vi "Autonomous Independent.vi"() -> ()   [LabVIEW 2014]
doc: "This VI is called when autonomous begins, and will automatically be terminated when autonomous ends. You can carry out timed or sensor driven robot movement independently without needing to return to the caller."
uses:
  Robot Global Data.vi
  <vilib>/Rock Robotics/Network Tables/SD Write Number.vi
  <vilib>/Rock Robotics/Network Tables/SD Read Number.vi
  <vilib>/Rock Robotics/WPI/RobotDrive/WPI_RobotDriveMecanumDrive_Cartesian.vi
  <vilib>/Rock Robotics/Network Tables/SD Write Numeric Array.vi
panel:
  out "Current Movement, for debugging":T1 {"Z Joystick Value" scale=-1.0..1.0; "Y Joystick Value" scale=1.0..-1.0; "X Joystick Value" scale=-1.0..1.0}
  in  "Array of robot movements":T2(array[cluster]) {"Z Joystick Value" scale=-1.0..1.0; "Y Joystick Value" scale=1.0..-1.0; "X Joystick Value" scale=-1.0..1.0}
  # "Be sure to right-click and choose Data Operations>>Make Current Value default if you want to save the array values with the VI"
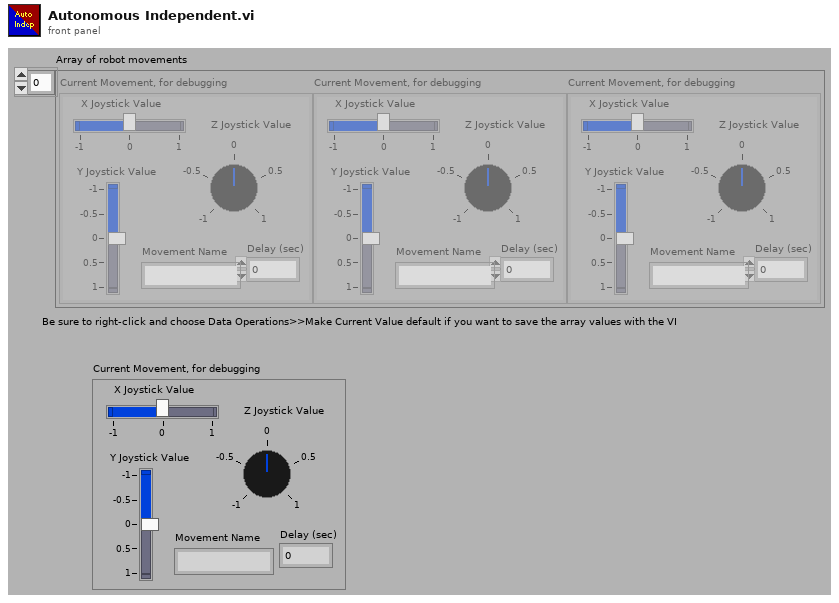
[diagram p1: front panel]
types:
  T1 = cluster{"X Joystick Value":dbl, "Y Joystick Value":dbl, "Z Joystick Value":dbl, "Delay (sec)":dbl, "Movement Name":string}
  T2 = cluster{"X Joystick Value":dbl, "Y Joystick Value":dbl, "Z Joystick Value":dbl, "Delay (sec)":dbl, "Movement Name":string}[]
  T3 = typedef "WPI_RobotDriveDevRef.ctl" = cluster{"DevStatus":errorcluster, "Motors[]":T4[], "Square Inputs":bool, "Max Output":dbl}
  T4 = typedef "WPI_MotorControlDeviceRef.ctl" = cluster{"DeviceStatus":errorcluster, "Type":T5, "PWM":cluster{"Controller":T6, "PWM Channel":T7, "DeadBand":T8}, "CAN":cluster{"Device Number":u8, "Control Mode":T9, "Semaphore":T10, "Max Vout":dbl, "TalonSRX Control Mode":T11}, "Invert":bool, "TransformRef":T12, "InvTransformRef":T12}
  T5 = typedef "WPI_MotorControlType.ctl" = enum16{"PWM", "CAN", "CANTalonSRX"}
  T6 = typedef "FPGA_TypedefDigitalModule.ctl" = enum16{"Controller 1"}
  T7 = typedef "FPGA_DIOPWMChannel.ctl" = enum8{"PWM 0", "PWM 1", "PWM 2", "PWM 3", "PWM 4", "PWM 5", "PWM 6", "PWM 7", "PWM 8", "PWM 9", "PWM MXP 0", "PWM MXP 1", "PWM MXP 2", "PWM MXP 3", "PWM MXP 4", "PWM MXP 5", "PWM MXP 6", "PWM MXP 7", "PWM MXP 8", "PWM MXP 9", "Invalid"}
  T8 = typedef "WPI_PWMDeadband.ctl" = cluster{"Name":string, "maxPositivePwm":i32, "minPositivePwm":i32, "centerPwm":i32, "maxNegativePwm":i32, "minNegativePwm":i32, "angularRange":u16}
  T9 = typedef "WPI_CANJaguar_ControlMode.ctl" = enum8{"Percent VBus", "Current", "Speed", "Position", "Voltage"}
  T10 = typedef "Semaphore RefNum" = refnum<k1>
  T11 = typedef "WPI_CANTalonSRX_APIControlMode.ctl" = enum8{"Percent VBus", "Speed", "Position", "Slave", "Unchanged / Invalid"}
  T12 = typedef "WPI_PWMTransform_ConPane.ctl" = refnum<vi>
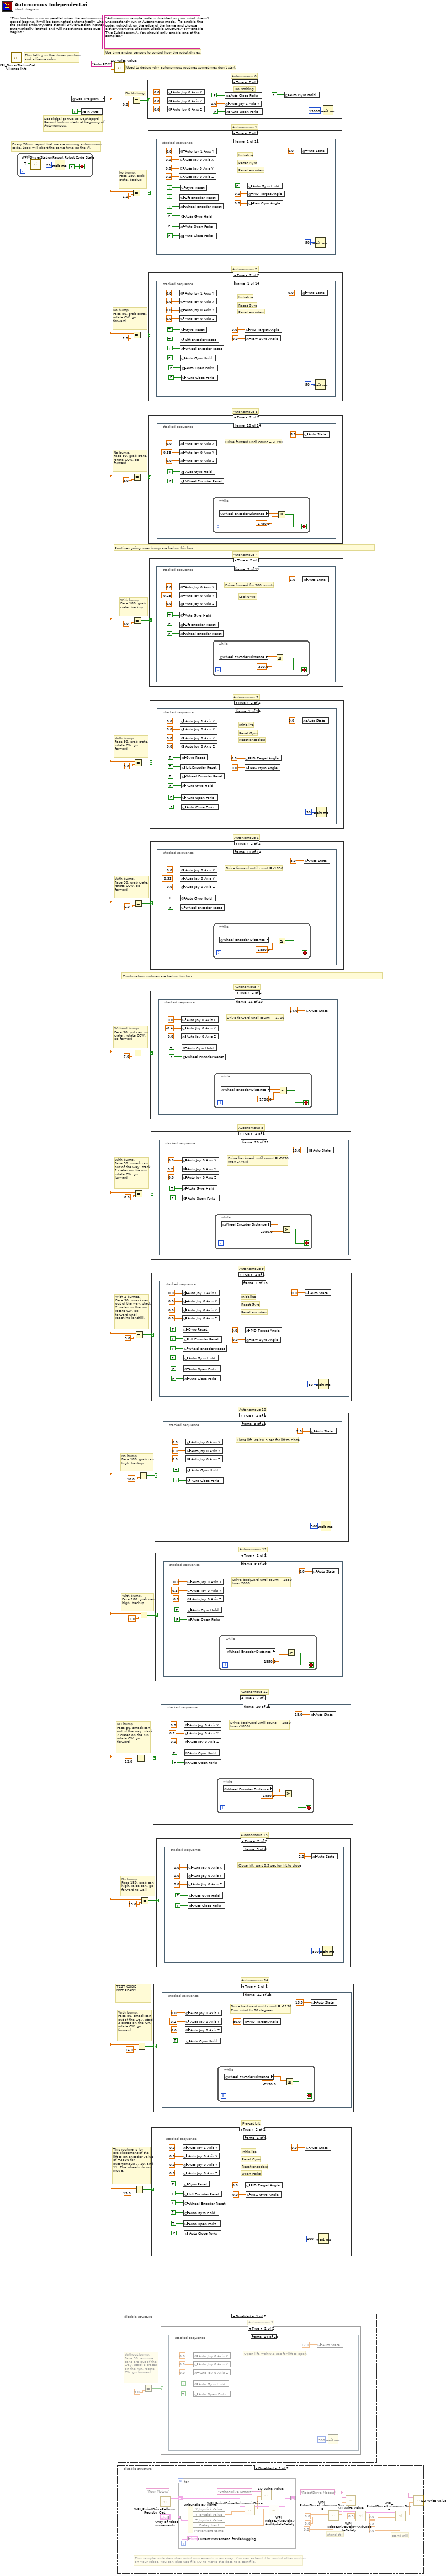
[diagram p0: block diagram]
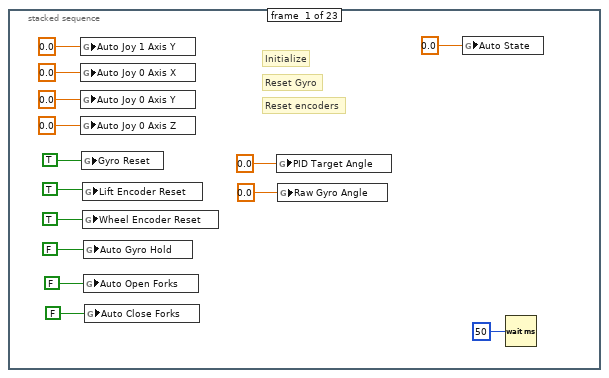
[diagram p3: hidden frame]
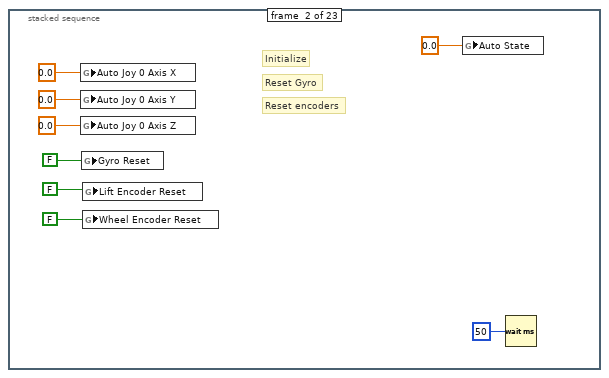
[diagram p4: hidden frame]
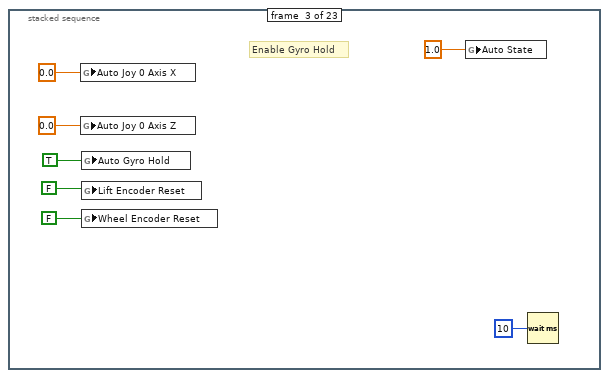
[diagram p5: hidden frame]
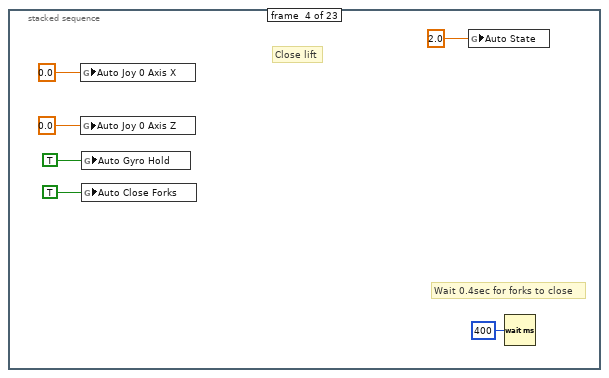
[diagram p6: hidden frame]
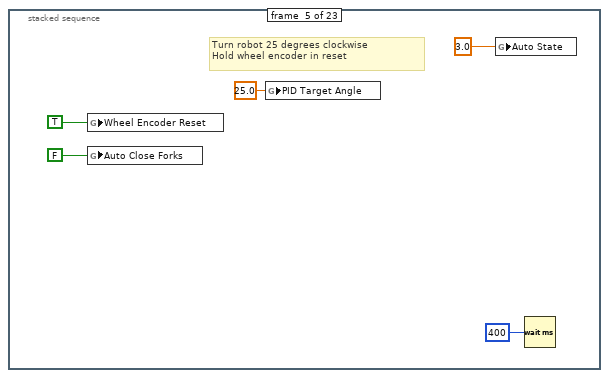
[diagram p7: hidden frame]
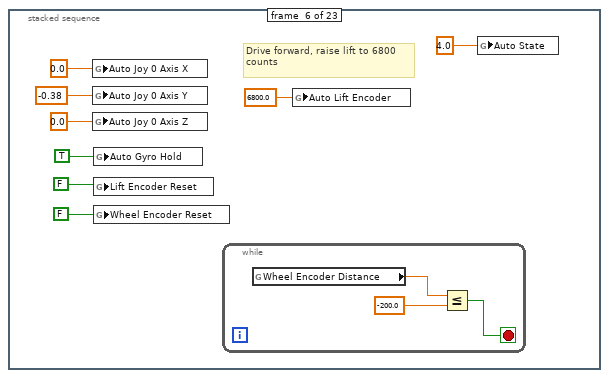
[diagram p8: hidden frame]
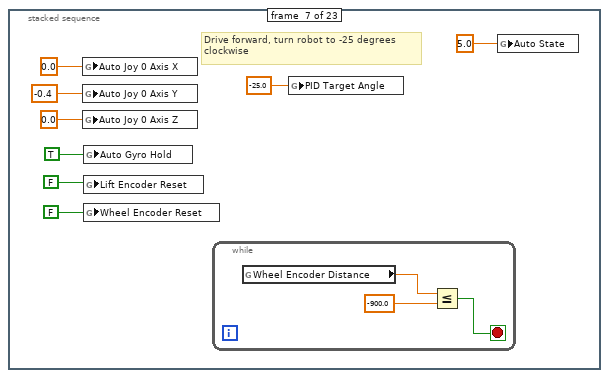
[diagram p9: hidden frame]
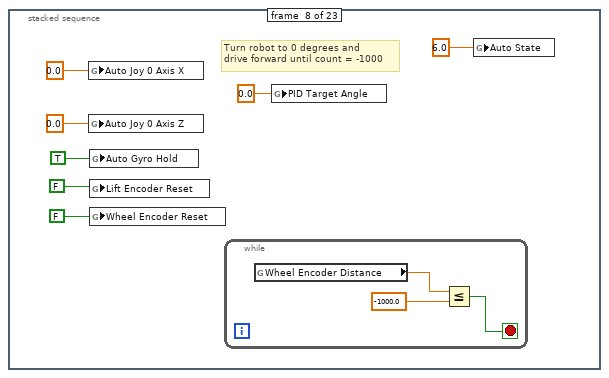
[diagram p10: hidden frame]
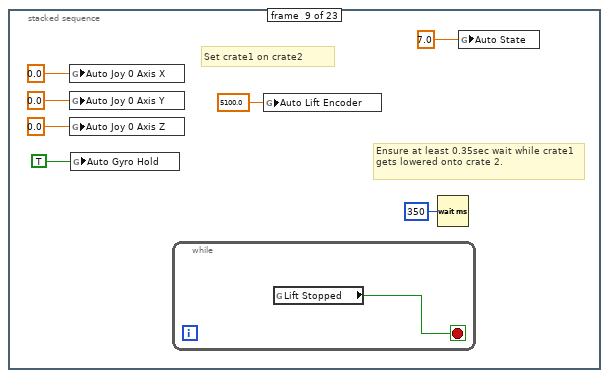
[diagram p11: hidden frame]
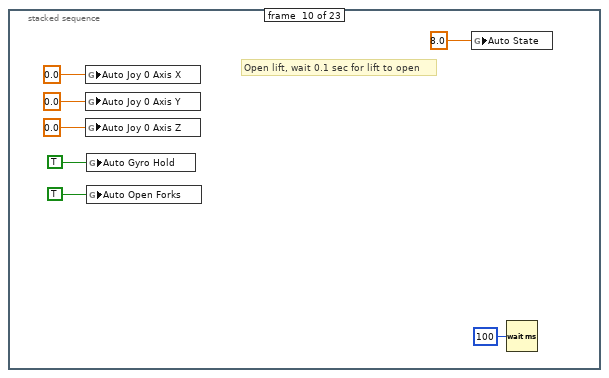
[diagram p12: hidden frame]
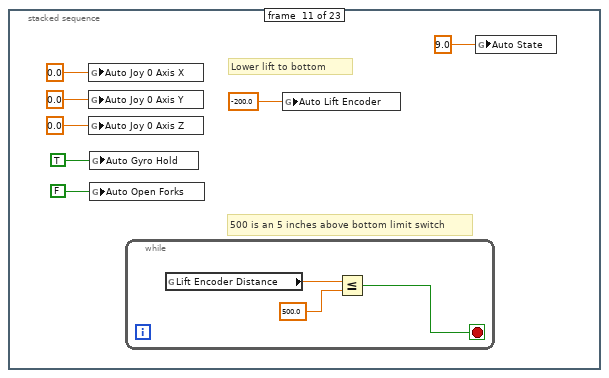
[diagram p13: hidden frame]
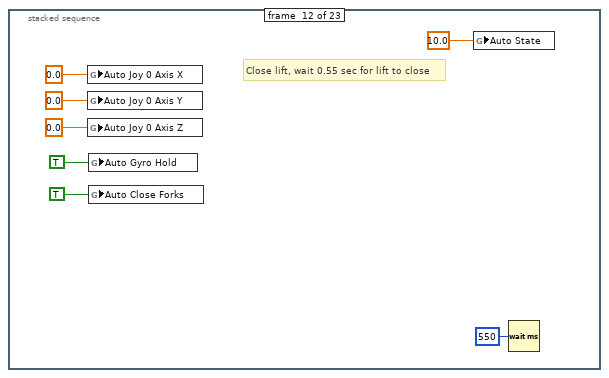
[diagram p14: hidden frame]
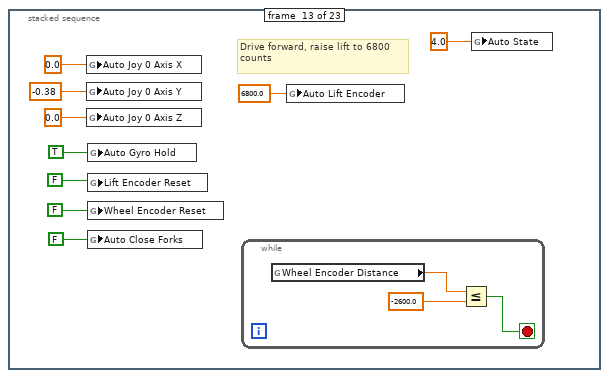
[diagram p15: hidden frame]
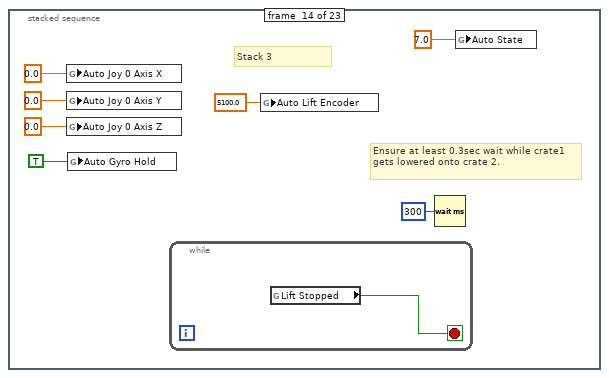
[diagram p16: hidden frame]
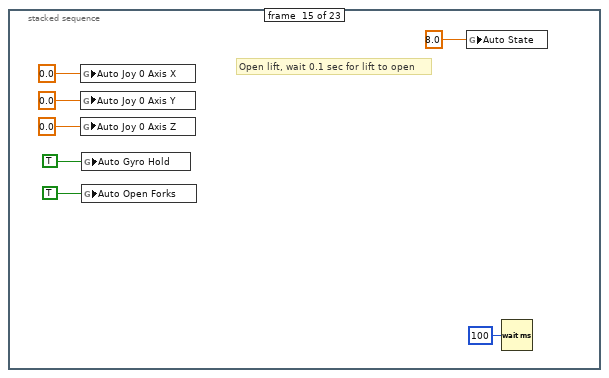
[diagram p17: hidden frame]
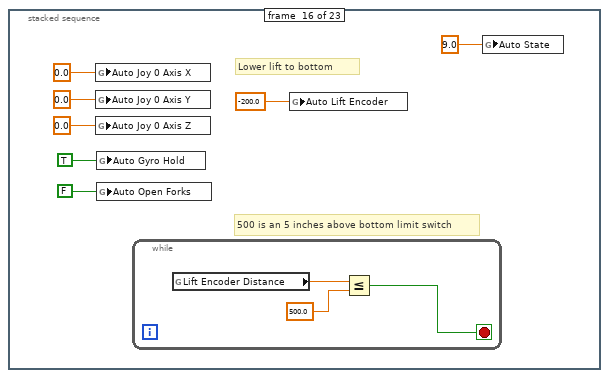
[diagram p18: hidden frame]
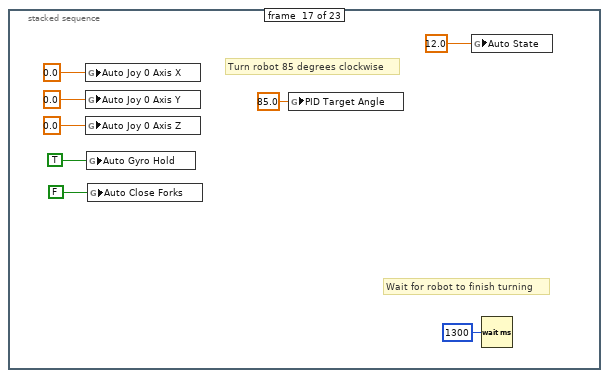
[diagram p19: hidden frame]
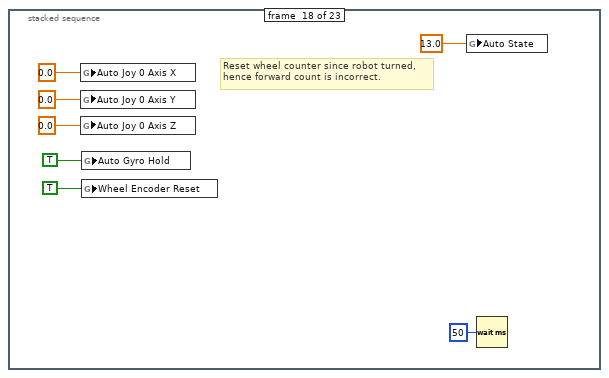
[diagram p20: hidden frame]
diagram:
  (unwired) "Autonomous sample code is disabled so your robot doesn't unexpectantly run in Autonomous mode.  To enable this code, right-click on the edge of the frame and choose either \"Remove Diagram Disable Structure\" or \"Enable This Subdiagram\". You should only enable one of the samples."
  (unwired) "This function is run in parallel when the autonomous period begins. It will be terminated automatically when the period ends.\n\nNote that all Driver Station inputs are automatically latched and will not change once auto begins."
  # "TEST CODE\nNOT READY"
  # "With bump.\nFace 90, smack can out of the way, stack 3 crates on the run, rotate CW, go forward"
  # "Autonomous 14"
  # "No bump.\nFace 180, grab can high, raise can, go forward to wall"
  # "Autonomous 13"
  # "Used to debug why autonomous routines sometimes don't start."
  # "NO bump.\nFace 90, smack can out of the way, stack 2 crates on the run, rotate CW, go forward"
  # "Autonomous 12"
  # "With bump.\nFace 180, grab can high, backup"
  # "Autonomous 11"
  # "No bump.\nFace 180, grab can high, backup"
  # "Autonomous 10"
  # "Set global to true so Dashboard Record funtion starts at begining of Autonomous."
  # "This routine is for pre-placement of the lift to an encoder value of +3500 for autonomous 7, 10, and 11. The wheels do not move."
  # "Pre-set Lift"
  # "With 2 bumps.\nFace 90, smack can out of the way, stack 2 crates on the run, rotate CW, go forward until reaching landfill."
  # "Autonomous 9"
  # "With bump.\nFace 90, smack can out of the way, stack 2 crates on the run, rotate CW, go forward"
  # "Autonomous 8"
  # "Without bump.\nFace 90, put can on crate , rotate CCW, go forward"
  # "Autonomous 7"
  # "Combination routines are below this box."
  # "With bump.\nFace 90, grab crate, rotate CCW, go forward"
  # "Autonomous 6"
  # "With bump.\nFace 90, grab crate, rotate CW, go forward"
  # "Autonomous 5"
  # "Routines going over bump are below this box."
  # "With bump.\nFace 180, grab crate, backup"
  # "Autonomous 4"
  # "No bump.\nFace 90, grab crate, rotate CCW, go forward"
  # "Autonomous 3"
  # "No bump.\nFace 90, grab crate, rotate CW, go forward"
  # "No bump.\nFace 180, grab crate, backup"
  # "Do Nothing"
  # "Autonomous 2"
  # "Autonomous 1"
  # "Autonomous 0"
  # "Every 20ms, report that we are running autonomous\ncode. Loop will abort the same time as the VI."
  # "Use time and/or sensors to control how the robot drives."
  # "This tells you the driver position\nand alliance color"
  n1 = call <vilib>:"WPI_DriverStationGet Alliance Info.vi"() -> ()  [unwired: 12 out]
  n2 = while {
    stop <- FALSE stop-if-true
    n3 = call <vilib>:"WPI_DriverStationReport Robot Code State.vi"("Autonomous"=TRUE) -> ()  [unwired: 10 in, 1 out]
    n4 = Wait (ms)(milliseconds to wait=u32 20) -> ()  [unwired: 1 out]
  }
  n5 = global read "Robot Global Data.vi" "Auto  Program"() -> (w1:dbl)
  n6 = global write "Robot Global Data.vi" "In Auto"(TRUE ("In Auto")) -> ()
  n7 = call-poly <vilib>:"SD Write Value.vi"("Numeric"=w1, "Name"="Auto PGM") -> ()  [unwired: 8 in, 2 out]
  n8 = disable-structure shown="Disabled" {
    frame Disabled {
      w50 = "RobotDrive Motors" ("Name")
      # "stand still"
      # "stand still"
      # "This sample code describes robot movements in an array. You can extend it to control other motors\non your robot. You can also use file I/O to move the data to a text file."
      n9 = call <vilib>:"WPI_RobotDriveRefNum Registry Get.vi"("refnum name"="Four Motors") -> ("RobotDriveDevRef"=w52:T3)  [unwired: 1 in, 9 out]
      n10 = for {
        shift-right: [w60] -> _
        shift-left: w52 -> [w61]
        tunnel: "Array of robot movements" -> [w56] mode=indexing
        n11 = Unbundle By Name(w56) -> ("X Joystick Value"=w59:dbl, "Y Joystick Value"=w58:dbl, "Z Joystick Value"=w55:dbl, "Delay (sec)"=w57:dbl)  [unwired: 1 out]
        n12 = call-poly <vilib>:"WPI_RobotDriveHolonomicDrive.vi"("Rotation"=w55, "Y"=w58, "X"=w59, "RobotDriveDevRef"=w61) -> ("Motor Values"=w54:dbl[], "RobotDriveDevRef"=w62:T3)  [unwired: 5 in, 1 out]
        n13 = call-poly <vilib>:"SD Write Value.vi"("Numeric Array"=w54, "Name"="RobotDrive Motors") -> ()  [unwired: 8 in, 2 out]
        n14 = call <vilib>:"WPI_RobotDriveDelayAndUpdateSafety.vi"("Delay (s)"=w57, "RobotDriveDevRef"=w62) -> ("RobotDriveDevRef 2"=w60:T3)  [unwired: 8 in, 1 out]
        "Current Movement, for debugging" <- w56
      }
      n15 = call-poly <vilib>:"WPI_RobotDriveHolonomicDrive.vi"("Rotation"=0.0, "Y"=0.0 ("X axis value"), "X"=0.0 ("X axis value")) -> ("Motor Values"=w48:dbl[], "RobotDriveDevRef"=w43:T3)  [unwired: 6 in, 1 out]
      n16 = call-poly <vilib>:"SD Write Value.vi"("Numeric Array"=w48, "Name"=w50) -> ()  [unwired: 8 in, 2 out]
      n17 = call <vilib>:"WPI_RobotDriveDelayAndUpdateSafety.vi"("Delay (s)"=0.5, "RobotDriveDevRef"=w43) -> ("RobotDriveDevRef 2"=w44:T3)  [unwired: 8 in, 1 out]
      n18 = call-poly <vilib>:"WPI_RobotDriveHolonomicDrive.vi"("Rotation"=0.0 ("X axis value"), "Y"=0.0 ("X axis value"), "X"=0.0 ("X axis value"), "RobotDriveDevRef"=w44) -> ("Motor Values"=w49:dbl[])  [unwired: 5 in, 2 out]
      n19 = call-poly <vilib>:"SD Write Value.vi"("Numeric Array"=w49, "Name"=w50) -> ()  [unwired: 8 in, 2 out]
    }
    frame Enabled {
    }
  }
  n20 = disable-structure shown="Disabled" {
    frame Disabled {
      # "Without bump.\nFace 90, assume cans are out of the way, stack 3 crates on the run, rotate CW, go forward"
      # "Autonomous 9"
      n21 = Equal?(y=9.0) -> (x=w64:dbl, x = y?=w65:bool)
      n22 = case shown="True" w65 {
        frame False {
        }
        frame True {
          n23 = stacked-sequence {
            frame #0 {
              # "Reset encoders"
              # "Reset Gyro"
              # "Initialize"
              n24 = global write "Robot Global Data.vi" "Auto Joy 1 Axis Y"(0.0 ("Auto Joy 0 Axis X")) -> ()
              n25 = global write "Robot Global Data.vi" "Auto Joy 0 Axis X"(0.0 ("Auto Joy 0 Axis X")) -> ()
              n26 = global write "Robot Global Data.vi" "Auto Joy 0 Axis Y"(0.0 ("Auto Joy 0 Axis X")) -> ()
              n27 = global write "Robot Global Data.vi" "Auto Joy 0 Axis Z"(0.0 ("Auto Joy 0 Axis X")) -> ()
              n28 = global write "Robot Global Data.vi" "Gyro Reset"(TRUE ("Auto Gyro Hold")) -> ()
              n29 = global write "Robot Global Data.vi" "Lift Encoder Reset"(TRUE ("Auto Gyro Hold")) -> ()
              n30 = global write "Robot Global Data.vi" "Wheel Encoder Reset"(TRUE ("Wheel Encoder Reset")) -> ()
              n31 = global write "Robot Global Data.vi" "Auto Gyro Hold"(FALSE ("Auto Gyro Hold")) -> ()
              n32 = global write "Robot Global Data.vi" "Auto Open Forks"(FALSE ("Auto Gyro Hold")) -> ()
              n33 = global write "Robot Global Data.vi" "Auto Close Forks"(FALSE ("Auto Gyro Hold")) -> ()
              n34 = global write "Robot Global Data.vi" "PID Target Angle"(0.0 ("Auto Joy 0 Axis Z")) -> ()
              n35 = global write "Robot Global Data.vi" "Raw Gyro Angle"(0.0 ("Auto Joy 0 Axis Z")) -> ()
              n36 = global write "Robot Global Data.vi" "Auto State"(0.0 ("Auto State")) -> ()
              n37 = Wait (ms)(milliseconds to wait=u32 50) -> ()  [unwired: 1 out]
            }
            frame #1 {
              # "Adjust this wait so it is long enought to allow alliance robots to get cans out of our way.\nSet to 2.0 seconds."
              # "Reset encoders"
              # "Reset Gyro"
              # "Initialize"
              n38 = global write "Robot Global Data.vi" "Auto Joy 0 Axis X"(0.0 ("Auto Joy 0 Axis X")) -> ()
              n39 = global write "Robot Global Data.vi" "Auto Joy 0 Axis Y"(0.0 ("Auto Joy 0 Axis X")) -> ()
              n40 = global write "Robot Global Data.vi" "Auto Joy 0 Axis Z"(0.0 ("Auto Joy 0 Axis X")) -> ()
              n41 = global write "Robot Global Data.vi" "Gyro Reset"(FALSE ("Auto Gyro Hold")) -> ()
              n42 = global write "Robot Global Data.vi" "Lift Encoder Reset"(FALSE ("Auto Gyro Hold")) -> ()
              n43 = global write "Robot Global Data.vi" "Wheel Encoder Reset"(FALSE ("Wheel Encoder Reset")) -> ()
              n44 = global write "Robot Global Data.vi" "Auto State"(0.0 ("Auto State")) -> ()
              n45 = Wait (ms)(milliseconds to wait=u32 2000) -> ()  [unwired: 1 out]
            }
            frame #2 {
              # "Drive forward"
              n46 = global write "Robot Global Data.vi" "Auto Joy 0 Axis X"(0.0 ("Auto Joy 0 Axis X")) -> ()
              n47 = global write "Robot Global Data.vi" "Auto Joy 0 Axis Z"(0.0 ("Auto Joy 0 Axis X")) -> ()
              n48 = global write "Robot Global Data.vi" "Auto Gyro Hold"(TRUE ("Auto Gyro Hold")) -> ()
              n49 = global write "Robot Global Data.vi" "Lift Encoder Reset"(FALSE ("Auto Gyro Hold")) -> ()
              n50 = global write "Robot Global Data.vi" "Wheel Encoder Reset"(FALSE ("Wheel Encoder Reset")) -> ()
              n51 = while {
                stop <- w97 stop-if-true
                n52 = global read "Robot Global Data.vi" "Wheel Encoder Distance"() -> (w99:dbl)
                n53 = Less Or Equal?(x=w99, y=-10.0) -> (x <= y?=w97:bool)
              }
              n54 = call-poly <vilib>:"SD Read Value.vi"("Name"="Speed1") -> ("Numeric"=w89:dbl)  [unwired: 8 in, 2 out]
              n55 = global write "Robot Global Data.vi" "Auto Joy 0 Axis Y"(w89) -> ()
              n56 = global write "Robot Global Data.vi" "Auto State"(1.0 ("Auto State")) -> ()
            }
            frame #3 {
              # "Wait 0.5sec for forks to close"
              # "Close lift, keep plowing forward"
              n57 = global write "Robot Global Data.vi" "Auto Joy 0 Axis X"(0.0 ("Auto Joy 0 Axis X")) -> ()
              n58 = global write "Robot Global Data.vi" "Auto Joy 0 Axis Z"(0.0 ("Auto Joy 0 Axis X")) -> ()
              n59 = global write "Robot Global Data.vi" "Auto Gyro Hold"(TRUE ("Auto Gyro Hold")) -> ()
              n60 = global write "Robot Global Data.vi" "Auto Close Forks"(TRUE ("Auto Gyro Hold")) -> ()
              n61 = global write "Robot Global Data.vi" "Auto State"(2.0 ("Auto State")) -> ()
              n62 = Wait (ms)(milliseconds to wait=u32 500) -> ()  [unwired: 1 out]
            }
            frame #4 {
              # "Ensure at least a 2.0sec wait while driving forward and lifting."
              # "Lift up crate for ????? counts"
              n63 = global write "Robot Global Data.vi" "Auto Joy 0 Axis X"(0.0 ("Auto Joy 0 Axis X")) -> ()
              n64 = global write "Robot Global Data.vi" "Auto Joy 0 Axis Z"(0.0 ("Auto Joy 0 Axis X")) -> ()
              n65 = global write "Robot Global Data.vi" "Auto Gyro Hold"(TRUE ("Auto Gyro Hold")) -> ()
              n66 = global write "Robot Global Data.vi" "Auto Close Forks"(FALSE ("Auto Gyro Hold")) -> ()
              n67 = while {
                stop <- w114 stop-if-true
                n68 = global read "Robot Global Data.vi" "Lift Stopped"() -> (w114:bool)
              }
              n69 = call-poly <vilib>:"SD Read Value.vi"("Name"="LE1") -> ("Numeric"=w106:dbl)  [unwired: 8 in, 2 out]
              n70 = global write "Robot Global Data.vi" "Auto Lift Encoder"(w106) -> ()
              n71 = Wait (ms)(milliseconds to wait=u32 2000) -> ()  [unwired: 1 out]
              n72 = global write "Robot Global Data.vi" "Auto State"(3.0 ("Auto State")) -> ()
            }
            frame #5 {
              # "Drive forward until count = -????"
              n73 = global write "Robot Global Data.vi" "Auto Joy 0 Axis X"(0.0 ("Auto Joy 0 Axis X")) -> ()
              n74 = global write "Robot Global Data.vi" "Auto Joy 0 Axis Z"(0.0 ("Auto Joy 0 Axis X")) -> ()
              n75 = global write "Robot Global Data.vi" "Auto Gyro Hold"(TRUE ("Auto Gyro Hold")) -> ()
              n76 = global write "Robot Global Data.vi" "Lift Encoder Reset"(FALSE ("Auto Gyro Hold")) -> ()
              n77 = global write "Robot Global Data.vi" "Wheel Encoder Reset"(FALSE ("Wheel Encoder Reset")) -> ()
              n78 = while {
                stop <- w123 stop-if-true
                n79 = global read "Robot Global Data.vi" "Wheel Encoder Distance"() -> (w124:dbl)
                n80 = call-poly <vilib>:"SD Read Value.vi"("Name"="WE1") -> ("Numeric"=w121:dbl)  [unwired: 8 in, 2 out]
                n81 = Less Or Equal?(x=w124, y=w121) -> (x <= y?=w123:bool)
              }
              n82 = global write "Robot Global Data.vi" "Auto State"(4.0 ("Auto State")) -> ()
            }
            frame #6 {
              # "Ensure at least 0.5sec wait while crate1 gets lowered onto crate 2."
              # "Set crate1 on crate2 and keep plowing"
              n83 = global write "Robot Global Data.vi" "Auto Joy 0 Axis X"(0.0 ("Auto Joy 0 Axis X")) -> ()
              n84 = global write "Robot Global Data.vi" "Auto Joy 0 Axis Z"(0.0 ("Auto Joy 0 Axis X")) -> ()
              n85 = global write "Robot Global Data.vi" "Auto Gyro Hold"(TRUE ("Auto Gyro Hold")) -> ()
              n86 = while {
                stop <- w132 stop-if-true
                n87 = global read "Robot Global Data.vi" "Lift Stopped"() -> (w132:bool)
              }
              n88 = call-poly <vilib>:"SD Read Value.vi"("Name"="LE2") -> ("Numeric"=w125:dbl)  [unwired: 8 in, 2 out]
              n89 = global write "Robot Global Data.vi" "Auto Lift Encoder"(w125) -> ()
              n90 = Wait (ms)(milliseconds to wait=u32 500) -> ()  [unwired: 1 out]
              n91 = global write "Robot Global Data.vi" "Auto State"(5.0 ("Auto State")) -> ()
            }
            frame #7 {
              # "Open lift, wait 0.3 sec for lift to open"
              n92 = global write "Robot Global Data.vi" "Auto Joy 0 Axis X"(0.0 ("Auto Joy 0 Axis X")) -> ()
              n93 = global write "Robot Global Data.vi" "Auto Joy 0 Axis Z"(0.0 ("Auto Joy 0 Axis X")) -> ()
              n94 = global write "Robot Global Data.vi" "Auto Gyro Hold"(TRUE ("Auto Gyro Hold")) -> ()
              n95 = global write "Robot Global Data.vi" "Auto Open Forks"(TRUE ("Auto Gyro Hold")) -> ()
              n96 = global write "Robot Global Data.vi" "Auto State"(6.0 ("Auto State")) -> ()
              n97 = Wait (ms)(milliseconds to wait=u32 300) -> ()  [unwired: 1 out]
            }
            frame #8 {
              # "100 is an inch above bottom limit switch"
              # "Lower lift to bottom and keep plowing"
              n98 = global write "Robot Global Data.vi" "Auto Joy 0 Axis X"(0.0 ("Auto Joy 0 Axis X")) -> ()
              n99 = global write "Robot Global Data.vi" "Auto Joy 0 Axis Z"(0.0 ("Auto Joy 0 Axis X")) -> ()
              n100 = global write "Robot Global Data.vi" "Auto Gyro Hold"(TRUE ("Auto Gyro Hold")) -> ()
              n101 = global write "Robot Global Data.vi" "Auto Open Forks"(FALSE ("Auto Gyro Hold")) -> ()
              n102 = while {
                stop <- w145 stop-if-true
                n103 = global read "Robot Global Data.vi" "Lift Encoder Distance"() -> (w147:dbl)
                n104 = Less Or Equal?(x=w147, y=100.0) -> (x <= y?=w145:bool)
              }
              n105 = global write "Robot Global Data.vi" "Auto Lift Encoder"(-200.0 ("Auto Joy 0 Axis X")) -> ()
              n106 = global write "Robot Global Data.vi" "Auto State"(7.0 ("Auto State")) -> ()
            }
            frame #9 {
              # "Close lift, wait 0.4 sec for lift to close and keep plowing with 2 crates"
              n107 = global write "Robot Global Data.vi" "Auto Joy 0 Axis X"(0.0 ("Auto Joy 0 Axis X")) -> ()
              n108 = global write "Robot Global Data.vi" "Auto Joy 0 Axis Z"(0.0 ("Auto Joy 0 Axis X")) -> ()
              n109 = global write "Robot Global Data.vi" "Auto Gyro Hold"(TRUE ("Auto Gyro Hold")) -> ()
              n110 = global write "Robot Global Data.vi" "Auto Close Forks"(TRUE ("Auto Gyro Hold")) -> ()
              n111 = global write "Robot Global Data.vi" "Auto State"(8.0 ("Auto State")) -> ()
              n112 = Wait (ms)(milliseconds to wait=u32 400) -> ()  [unwired: 1 out]
            }
            frame #10 {
              # "Ensure at least 2.0sec wait while crate1 and 2 gets raised onto crate 3."
              # "Ensure at least 0.5sec wait"
              # "Lift up can for ????? counts, keep plowing"
              n113 = global write "Robot Global Data.vi" "Auto Joy 0 Axis X"(0.0 ("Auto Joy 0 Axis X")) -> ()
              n114 = global write "Robot Global Data.vi" "Auto Joy 0 Axis Z"(0.0 ("Auto Joy 0 Axis X")) -> ()
              n115 = global write "Robot Global Data.vi" "Auto Gyro Hold"(TRUE ("Auto Gyro Hold")) -> ()
              n116 = global write "Robot Global Data.vi" "Auto Close Forks"(FALSE ("Auto Gyro Hold")) -> ()
              n117 = while {
                stop <- w162 stop-if-true
                n118 = global read "Robot Global Data.vi" "Lift Stopped"() -> (w162:bool)
              }
              n119 = call-poly <vilib>:"SD Read Value.vi"("Name"="LE3") -> ("Numeric"=w154:dbl)  [unwired: 8 in, 2 out]
              n120 = global write "Robot Global Data.vi" "Auto Lift Encoder"(w154) -> ()
              n121 = Wait (ms)(milliseconds to wait=u32 2000) -> ()  [unwired: 1 out]
              n122 = global write "Robot Global Data.vi" "Auto State"(9.0 ("Auto State")) -> ()
            }
            frame #11 {
              # "Drive forward until count = -????\nRobot should end up at base of\n3rd crate."
              n123 = global write "Robot Global Data.vi" "Auto Joy 0 Axis X"(0.0 ("Auto Joy 0 Axis X")) -> ()
              n124 = global write "Robot Global Data.vi" "Auto Joy 0 Axis Z"(0.0 ("Auto Joy 0 Axis X")) -> ()
              n125 = global write "Robot Global Data.vi" "Auto Gyro Hold"(TRUE ("Auto Gyro Hold")) -> ()
              n126 = global write "Robot Global Data.vi" "Lift Encoder Reset"(FALSE ("Auto Gyro Hold")) -> ()
              n127 = global write "Robot Global Data.vi" "Wheel Encoder Reset"(FALSE ("Wheel Encoder Reset")) -> ()
              n128 = while {
                stop <- w171 stop-if-true
                n129 = global read "Robot Global Data.vi" "Wheel Encoder Distance"() -> (w172:dbl)
                n130 = call-poly <vilib>:"SD Read Value.vi"("Name"="WE2") -> ("Numeric"=w169:dbl)  [unwired: 8 in, 2 out]
                n131 = Less Or Equal?(x=w172, y=w169) -> (x <= y?=w171:bool)
              }
              n132 = global write "Robot Global Data.vi" "Auto State"(10.0 ("Auto State")) -> ()
            }
            frame #12 {
              # "Ensure at least 0.5sec wait while crate1 gets lowered onto crate 2."
              # "Set crate1 and 2 on crate3"
              n133 = global write "Robot Global Data.vi" "Auto Joy 0 Axis X"(0.0 ("Auto Joy 0 Axis X")) -> ()
              n134 = global write "Robot Global Data.vi" "Auto Joy 0 Axis Y"(0.0 ("Auto Joy 0 Axis X")) -> ()
              n135 = global write "Robot Global Data.vi" "Auto Joy 0 Axis Z"(0.0 ("Auto Joy 0 Axis X")) -> ()
              n136 = global write "Robot Global Data.vi" "Auto Gyro Hold"(TRUE ("Auto Gyro Hold")) -> ()
              n137 = while {
                stop <- w181 stop-if-true
                n138 = global read "Robot Global Data.vi" "Lift Stopped"() -> (w181:bool)
              }
              n139 = call-poly <vilib>:"SD Read Value.vi"("Name"="LE4") -> ("Numeric"=w174:dbl)  [unwired: 8 in, 2 out]
              n140 = global write "Robot Global Data.vi" "Auto Lift Encoder"(w174) -> ()
              n141 = Wait (ms)(milliseconds to wait=u32 500) -> ()  [unwired: 1 out]
              n142 = global write "Robot Global Data.vi" "Auto State"(11.0 ("Auto State")) -> ()
            }
            frame #13 {
              # "Open lift, wait 0.3 sec for lift to open"
              n143 = global write "Robot Global Data.vi" "Auto Joy 0 Axis X"(0.0 ("Auto Joy 0 Axis X")) -> ()
              n144 = global write "Robot Global Data.vi" "Auto Joy 0 Axis Y"(0.0 ("Auto Joy 0 Axis X")) -> ()
              n145 = global write "Robot Global Data.vi" "Auto Joy 0 Axis Z"(0.0 ("Auto Joy 0 Axis X")) -> ()
              n146 = global write "Robot Global Data.vi" "Auto Gyro Hold"(TRUE ("Auto Gyro Hold")) -> ()
              n147 = global write "Robot Global Data.vi" "Auto Open Forks"(TRUE ("Auto Gyro Hold")) -> ()
              n148 = global write "Robot Global Data.vi" "Auto State"(12.0 ("Auto State")) -> ()
              n149 = Wait (ms)(milliseconds to wait=u32 300) -> ()  [unwired: 1 out]
            }
            frame #14 {
              # "100 is an inch above bottom limit switch"
              # "Lower lift to bottom and keep plowing"
              n150 = global write "Robot Global Data.vi" "Auto Joy 0 Axis X"(0.0 ("Auto Joy 0 Axis X")) -> ()
              n151 = global write "Robot Global Data.vi" "Auto Joy 0 Axis Y"(0.0 ("Auto Joy 0 Axis X")) -> ()
              n152 = global write "Robot Global Data.vi" "Auto Joy 0 Axis Z"(0.0 ("Auto Joy 0 Axis X")) -> ()
              n153 = global write "Robot Global Data.vi" "Auto Gyro Hold"(TRUE ("Auto Gyro Hold")) -> ()
              n154 = global write "Robot Global Data.vi" "Auto Open Forks"(FALSE ("Auto Gyro Hold")) -> ()
              n155 = while {
                stop <- w196 stop-if-true
                n156 = global read "Robot Global Data.vi" "Lift Encoder Distance"() -> (w198:dbl)
                n157 = Less Or Equal?(x=w198, y=100.0) -> (x <= y?=w196:bool)
              }
              n158 = global write "Robot Global Data.vi" "Auto Lift Encoder"(-200.0 ("Auto Joy 0 Axis X")) -> ()
              n159 = global write "Robot Global Data.vi" "Auto State"(13.0 ("Auto State")) -> ()
            }
            frame #15 {
              # "Close lift, wait 0.4 sec for lift to close and keep plowing with 2 crates"
              n160 = global write "Robot Global Data.vi" "Auto Joy 0 Axis X"(0.0 ("Auto Joy 0 Axis X")) -> ()
              n161 = global write "Robot Global Data.vi" "Auto Joy 0 Axis Y"(0.0 ("Auto Joy 0 Axis X")) -> ()
              n162 = global write "Robot Global Data.vi" "Auto Joy 0 Axis Z"(0.0 ("Auto Joy 0 Axis X")) -> ()
              n163 = global write "Robot Global Data.vi" "Auto Gyro Hold"(TRUE ("Auto Gyro Hold")) -> ()
              n164 = global write "Robot Global Data.vi" "Auto Close Forks"(TRUE ("Auto Gyro Hold")) -> ()
              n165 = global write "Robot Global Data.vi" "Auto State"(14.0 ("Auto State")) -> ()
              n166 = Wait (ms)(milliseconds to wait=u32 400) -> ()  [unwired: 1 out]
            }
            frame #16 {
              # "Ensure at least 0.5sec wait"
              # "Lift up crate for 1500 counts"
              n167 = global write "Robot Global Data.vi" "Auto Joy 0 Axis X"(0.0 ("Auto Joy 0 Axis X")) -> ()
              n168 = global write "Robot Global Data.vi" "Auto Joy 0 Axis Y"(0.0 ("Auto Joy 0 Axis X")) -> ()
              n169 = global write "Robot Global Data.vi" "Auto Joy 0 Axis Z"(0.0 ("Auto Joy 0 Axis X")) -> ()
              n170 = global write "Robot Global Data.vi" "Auto Gyro Hold"(TRUE ("Auto Gyro Hold")) -> ()
              n171 = global write "Robot Global Data.vi" "Auto Close Forks"(FALSE ("Auto Gyro Hold")) -> ()
              n172 = while {
                stop <- w214 stop-if-true
                n173 = global read "Robot Global Data.vi" "Lift Stopped"() -> (w214:bool)
              }
              n174 = global write "Robot Global Data.vi" "Auto Lift Encoder"(2000.0 ("Auto Joy 0 Axis X")) -> ()
              n175 = Wait (ms)(milliseconds to wait=u32 500) -> ()  [unwired: 1 out]
              n176 = global write "Robot Global Data.vi" "Auto State"(15.0 ("Auto State")) -> ()
            }
            frame #17 {
              # "Wait for robot to finish turning"
              # "Turn robot 90 degrees clockwise"
              n177 = global write "Robot Global Data.vi" "Auto Joy 0 Axis X"(0.0 ("Auto Joy 0 Axis X")) -> ()
              n178 = global write "Robot Global Data.vi" "Auto Joy 0 Axis Y"(0.0 ("Auto Joy 0 Axis X")) -> ()
              n179 = global write "Robot Global Data.vi" "Auto Joy 0 Axis Z"(0.0 ("Auto Joy 0 Axis X")) -> ()
              n180 = global write "Robot Global Data.vi" "Auto Gyro Hold"(TRUE ("Auto Gyro Hold")) -> ()
              n181 = global write "Robot Global Data.vi" "Auto Close Forks"(FALSE ("Auto Gyro Hold")) -> ()
              n182 = global write "Robot Global Data.vi" "PID Target Angle"(90.0 ("Auto Joy 0 Axis Z")) -> ()
              n183 = global write "Robot Global Data.vi" "Auto State"(16.0 ("Auto State")) -> ()
              n184 = Wait (ms)(milliseconds to wait=u32 2000) -> ()  [unwired: 1 out]
            }
            frame #18 {
              # "Reset wheel counter since robot turned,\nhence forward count is incorrect."
              n185 = global write "Robot Global Data.vi" "Auto Joy 0 Axis X"(0.0 ("Auto Joy 0 Axis X")) -> ()
              n186 = global write "Robot Global Data.vi" "Auto Joy 0 Axis Y"(0.0 ("Auto Joy 0 Axis X")) -> ()
              n187 = global write "Robot Global Data.vi" "Auto Joy 0 Axis Z"(0.0 ("Auto Joy 0 Axis X")) -> ()
              n188 = global write "Robot Global Data.vi" "Auto Gyro Hold"(TRUE ("Auto Gyro Hold")) -> ()
              n189 = global write "Robot Global Data.vi" "Wheel Encoder Reset"(TRUE ("Wheel Encoder Reset")) -> ()
              n190 = global write "Robot Global Data.vi" "Auto State"(17.0 ("Auto State")) -> ()
              n191 = Wait (ms)(milliseconds to wait=u32 50) -> ()  [unwired: 1 out]
            }
            frame #19 {
              # "Enable wheel counter."
              n192 = global write "Robot Global Data.vi" "Auto Joy 0 Axis X"(0.0 ("Auto Joy 0 Axis X")) -> ()
              n193 = global write "Robot Global Data.vi" "Auto Joy 0 Axis Y"(0.0 ("Auto Joy 0 Axis X")) -> ()
              n194 = global write "Robot Global Data.vi" "Auto Joy 0 Axis Z"(0.0 ("Auto Joy 0 Axis X")) -> ()
              n195 = global write "Robot Global Data.vi" "Auto Gyro Hold"(TRUE ("Auto Gyro Hold")) -> ()
              n196 = global write "Robot Global Data.vi" "Wheel Encoder Reset"(FALSE ("Wheel Encoder Reset")) -> ()
              n197 = global write "Robot Global Data.vi" "Auto State"(18.0 ("Auto State")) -> ()
              n198 = Wait (ms)(milliseconds to wait=u32 50) -> ()  [unwired: 1 out]
            }
            frame #20 {
              # "Drive forward until count = -???"
              n199 = global write "Robot Global Data.vi" "Auto Joy 0 Axis X"(0.0 ("Auto Joy 0 Axis X")) -> ()
              n200 = global write "Robot Global Data.vi" "Auto Joy 0 Axis Z"(0.0 ("Auto Joy 0 Axis X")) -> ()
              n201 = global write "Robot Global Data.vi" "Auto Gyro Hold"(TRUE ("Auto Gyro Hold")) -> ()
              n202 = global write "Robot Global Data.vi" "Wheel Encoder Reset"(FALSE ("Wheel Encoder Reset")) -> ()
              n203 = while {
                stop <- w244 stop-if-true
                n204 = global read "Robot Global Data.vi" "Wheel Encoder Distance"() -> (w245:dbl)
                n205 = call-poly <vilib>:"SD Read Value.vi"("Name"="WE3") -> ("Numeric"=w247:dbl)  [unwired: 8 in, 2 out]
                n206 = Less Or Equal?(x=w245, y=w247) -> (x <= y?=w244:bool)
              }
              n207 = call-poly <vilib>:"SD Read Value.vi"("Name"="Speed2") -> ("Numeric"=w237:dbl)  [unwired: 8 in, 2 out]
              n208 = global write "Robot Global Data.vi" "Auto Joy 0 Axis Y"(w237) -> ()
              n209 = global write "Robot Global Data.vi" "Auto State"(19.0 ("Auto State")) -> ()
            }
            frame #21 {
              # "100 is an inch above bottom limit switch\nNote: Trash Can keeps forks from engaing bottom limit\nswitch so use encoder!!!!"
              # "Stop robot, lower crate"
              n210 = global write "Robot Global Data.vi" "Auto Joy 0 Axis X"(0.0 ("Auto Joy 0 Axis X")) -> ()
              n211 = global write "Robot Global Data.vi" "Auto Joy 0 Axis Y"(0.0 ("Auto Joy 0 Axis X")) -> ()
              n212 = global write "Robot Global Data.vi" "Auto Joy 0 Axis Z"(0.0 ("Auto Joy 0 Axis X")) -> ()
              n213 = global write "Robot Global Data.vi" "Auto Gyro Hold"(TRUE ("Auto Gyro Hold")) -> ()
              n214 = while {
                stop <- w254 stop-if-true
                n215 = global read "Robot Global Data.vi" "Lift Encoder Distance"() -> (w256:dbl)
                n216 = Less Or Equal?(x=w256, y=100.0) -> (x <= y?=w254:bool)
              }
              n217 = global write "Robot Global Data.vi" "Auto Lift Encoder"(-200.0 ("Auto Joy 0 Axis X")) -> ()
              n218 = global write "Robot Global Data.vi" "Auto State"(20.0 ("Auto State")) -> ()
            }
            frame #22 {
              # "Open lift, wait 0.3 sec for lift to open"
              n219 = global write "Robot Global Data.vi" "Auto Joy 0 Axis X"(0.0 ("Auto Joy 0 Axis X")) -> ()
              n220 = global write "Robot Global Data.vi" "Auto Joy 0 Axis Y"(0.0 ("Auto Joy 0 Axis X")) -> ()
              n221 = global write "Robot Global Data.vi" "Auto Joy 0 Axis Z"(0.0 ("Auto Joy 0 Axis X")) -> ()
              n222 = global write "Robot Global Data.vi" "Auto Gyro Hold"(TRUE ("Auto Gyro Hold")) -> ()
              n223 = global write "Robot Global Data.vi" "Auto Open Forks"(TRUE ("Auto Gyro Hold")) -> ()
              n224 = global write "Robot Global Data.vi" "Auto State"(21.0 ("Auto State")) -> ()
              n225 = Wait (ms)(milliseconds to wait=u32 300) -> ()  [unwired: 1 out]
            }
            frame #23 {
              # "Drive backward until count = -????"
              n226 = global write "Robot Global Data.vi" "Auto Joy 0 Axis X"(0.0 ("Auto Joy 0 Axis X")) -> ()
              n227 = global write "Robot Global Data.vi" "Auto Joy 0 Axis Y"(0.2 ("Auto Joy 0 Axis X")) -> ()
              n228 = global write "Robot Global Data.vi" "Auto Joy 0 Axis Z"(0.0 ("Auto Joy 0 Axis X")) -> ()
              n229 = global write "Robot Global Data.vi" "Auto Gyro Hold"(TRUE ("Auto Gyro Hold")) -> ()
              n230 = global write "Robot Global Data.vi" "Auto Open Forks"(FALSE ("Auto Gyro Hold")) -> ()
              n231 = while {
                stop <- w273 stop-if-true
                n232 = global read "Robot Global Data.vi" "Wheel Encoder Distance"() -> (w272:dbl)
                n233 = call-poly <vilib>:"SD Read Value.vi"("Name"="WE4") -> ("Numeric"=w270:dbl)  [unwired: 8 in, 2 out]
                n234 = Greater Or Equal?(x=w272, y=w270) -> (x >= y?=w273:bool)
              }
              n235 = global write "Robot Global Data.vi" "Auto State"(22.0 ("Auto State")) -> ()
            }
            frame #24 {
              # "Stop and wait until teleop"
              n236 = global write "Robot Global Data.vi" "Auto Joy 0 Axis X"(0.0 ("Auto Joy 0 Axis X")) -> ()
              n237 = global write "Robot Global Data.vi" "Auto Joy 0 Axis Y"(0.0 ("Auto Joy 0 Axis X")) -> ()
              n238 = global write "Robot Global Data.vi" "Auto Joy 0 Axis Z"(0.0 ("Auto Joy 0 Axis X")) -> ()
              n239 = global write "Robot Global Data.vi" "Auto Gyro Hold"(FALSE ("Auto Gyro Hold")) -> ()
              n240 = global write "Robot Global Data.vi" "Auto State"(23.0 ("Auto State")) -> ()
              n241 = Wait (ms)(milliseconds to wait=u32 15000) -> ()  [unwired: 1 out]
            }
          }
        }
      }
    }
    frame Enabled {
    }
  }
  n242 = Equal?(x=w1, y=0.0) -> (x = y?=w33:bool)
  n243 = Equal?(x=w1, y=1.0) -> (x = y?=w32:bool)
  n244 = Equal?(x=w1, y=2.0) -> (x = y?=w30:bool)
  n245 = Equal?(x=w1, y=3.0) -> (x = y?=w22:bool)
  n246 = Equal?(x=w1, y=4.0) -> (x = y?=w27:bool)
  n247 = Equal?(x=w1, y=7.0) -> (x = y?=w20:bool)
  n248 = Equal?(x=w1, y=5.0) -> (x = y?=w25:bool)
  n249 = Equal?(x=w1, y=6.0) -> (x = y?=w23:bool)
  n250 = Equal?(x=w1, y=8.0) -> (x = y?=w18:bool)
  n251 = Equal?(x=w1, y=9.0) -> (x = y?=w16:bool)
  n252 = Equal?(x=w1, y=15.0) -> (x = y?=w14:bool)
  n253 = Equal?(x=w1, y=12.0) -> (x = y?=w7:bool)
  n254 = Equal?(x=w1, y=14.0) -> (x = y?=w2:bool)
  n255 = Equal?(x=w1, y=10.0) -> (x = y?=w11:bool)
  n256 = Equal?(x=w1, y=11.0) -> (x = y?=w9:bool)
  n257 = Equal?(x=w1, y=13.0) -> (x = y?=w4:bool)
  n258 = case shown="True" w33 {
    frame False {
    }
    frame True {
      # "Do Nothing"
      n259 = global write "Robot Global Data.vi" "Auto Joy 0 Axis X"(0.0 ("Auto Joy 0 Axis X")) -> ()
      n260 = global write "Robot Global Data.vi" "Auto Joy 0 Axis Y"(0.0 ("Auto Joy 0 Axis X")) -> ()
      n261 = global write "Robot Global Data.vi" "Auto Joy 0 Axis Z"(0.0 ("Auto Joy 0 Axis X")) -> ()
      n262 = global write "Robot Global Data.vi" "Auto Joy 1 Axis Y"(0.0 ("Auto Joy 0 Axis X")) -> ()
      n263 = global write "Robot Global Data.vi" "Auto Close Forks"(FALSE ("Auto Gyro Hold")) -> ()
      n264 = global write "Robot Global Data.vi" "Auto Open Forks"(FALSE ("Auto Gyro Hold")) -> ()
      n265 = global write "Robot Global Data.vi" "Auto Gyro Hold"(FALSE ("Auto Gyro Hold")) -> ()
      n266 = Wait (ms)(milliseconds to wait=u32 15000) -> ()  [unwired: 1 out]
    }
  }
  n267 = case shown="True" w32 {
    frame False {
    }
    frame True {
      n268 = stacked-sequence {
        frame #0 {
          # "Reset encoders"
          # "Reset Gyro"
          # "Initialize"
          n269 = global write "Robot Global Data.vi" "Auto Joy 0 Axis X"(0.0 ("Auto Joy 0 Axis X")) -> ()
          n270 = global write "Robot Global Data.vi" "Auto Joy 0 Axis Y"(0.0 ("Auto Joy 0 Axis X")) -> ()
          n271 = global write "Robot Global Data.vi" "Auto Joy 0 Axis Z"(0.0 ("Auto Joy 0 Axis X")) -> ()
          n272 = global write "Robot Global Data.vi" "Auto Joy 1 Axis Y"(0.0 ("Auto Joy 0 Axis X")) -> ()
          n273 = global write "Robot Global Data.vi" "Auto Open Forks"(FALSE ("Auto Gyro Hold")) -> ()
          n274 = global write "Robot Global Data.vi" "Lift Encoder Reset"(TRUE ("Auto Gyro Hold")) -> ()
          n275 = global write "Robot Global Data.vi" "Wheel Encoder Reset"(TRUE ("Wheel Encoder Reset")) -> ()
          n276 = global write "Robot Global Data.vi" "Auto Close Forks"(FALSE ("Auto Gyro Hold")) -> ()
          n277 = global write "Robot Global Data.vi" "Auto Gyro Hold"(FALSE ("Auto Gyro Hold")) -> ()
          n278 = global write "Robot Global Data.vi" "Gyro Reset"(TRUE ("Auto Gyro Hold")) -> ()
          n279 = global write "Robot Global Data.vi" "Auto Gyro Hold"(FALSE ("Auto Gyro Hold")) -> ()
          n280 = global write "Robot Global Data.vi" "PID Target Angle"(0.0 ("Auto Joy 0 Axis Z")) -> ()
          n281 = global write "Robot Global Data.vi" "Raw Gyro Angle"(0.0 ("Auto Joy 0 Axis Z")) -> ()
          n282 = global write "Robot Global Data.vi" "Auto State"(0.0 ("Auto State")) -> ()
          n283 = Wait (ms)(milliseconds to wait=u32 50) -> ()  [unwired: 1 out]
        }
        frame #1 {
          # "Initialize"
          n284 = global write "Robot Global Data.vi" "Auto Joy 0 Axis X"(0.0 ("Auto Joy 0 Axis X")) -> ()
          n285 = global write "Robot Global Data.vi" "Auto Joy 0 Axis Y"(0.0 ("Auto Joy 0 Axis X")) -> ()
          n286 = global write "Robot Global Data.vi" "Auto Joy 0 Axis Z"(0.0 ("Auto Joy 0 Axis X")) -> ()
          n287 = global write "Robot Global Data.vi" "Lift Encoder Reset"(FALSE ("Auto Gyro Hold")) -> ()
          n288 = global write "Robot Global Data.vi" "Wheel Encoder Reset"(FALSE ("Wheel Encoder Reset")) -> ()
          n289 = global write "Robot Global Data.vi" "Gyro Reset"(FALSE ("Auto Gyro Hold")) -> ()
          n290 = global write "Robot Global Data.vi" "Auto State"(0.0 ("Auto State")) -> ()
          n291 = Wait (ms)(milliseconds to wait=u32 50) -> ()  [unwired: 1 out]
        }
        frame #2 {
          # "Lock Gyro"
          # "Drive forward for 300 counts"
          n292 = global write "Robot Global Data.vi" "Auto Joy 0 Axis X"(0.0 ("Auto Joy 0 Axis X")) -> ()
          n293 = global write "Robot Global Data.vi" "Auto Joy 0 Axis Y"(-0.25 ("Auto Joy 0 Axis X")) -> ()
          n294 = global write "Robot Global Data.vi" "Auto Joy 0 Axis Z"(0.0 ("Auto Joy 0 Axis X")) -> ()
          n295 = global write "Robot Global Data.vi" "Auto Gyro Hold"(TRUE ("Auto Gyro Hold")) -> ()
          n296 = global write "Robot Global Data.vi" "Lift Encoder Reset"(FALSE ("Auto Gyro Hold")) -> ()
          n297 = global write "Robot Global Data.vi" "Wheel Encoder Reset"(FALSE ("Wheel Encoder Reset")) -> ()
          n298 = while {
            stop <- w318 stop-if-true
            n299 = global read "Robot Global Data.vi" "Wheel Encoder Distance"() -> (w320:dbl)
            n300 = Less Or Equal?(x=w320, y=-300.0) -> (x <= y?=w318:bool)
          }
          n301 = global write "Robot Global Data.vi" "Auto State"(1.0 ("Auto State")) -> ()
        }
        frame #3 {
          # "Stop robot and wait 0.1 sec"
          n302 = global write "Robot Global Data.vi" "Auto Joy 0 Axis X"(0.0 ("Auto Joy 0 Axis X")) -> ()
          n303 = global write "Robot Global Data.vi" "Auto Joy 0 Axis Y"(0.0 ("Auto Joy 0 Axis X")) -> ()
          n304 = global write "Robot Global Data.vi" "Auto Joy 0 Axis Z"(0.0 ("Auto Joy 0 Axis X")) -> ()
          n305 = global write "Robot Global Data.vi" "Auto Gyro Hold"(TRUE ("Auto Gyro Hold")) -> ()
          n306 = global write "Robot Global Data.vi" "Auto State"(2.0 ("Auto State")) -> ()
          n307 = Wait (ms)(milliseconds to wait=u32 100) -> ()  [unwired: 1 out]
        }
        frame #4 {
          # "Close lift, wait 0.5 sec for lift to close"
          n308 = global write "Robot Global Data.vi" "Auto Joy 0 Axis X"(0.0 ("Auto Joy 0 Axis X")) -> ()
          n309 = global write "Robot Global Data.vi" "Auto Joy 0 Axis Y"(0.0 ("Auto Joy 0 Axis X")) -> ()
          n310 = global write "Robot Global Data.vi" "Auto Joy 0 Axis Z"(0.0 ("Auto Joy 0 Axis X")) -> ()
          n311 = global write "Robot Global Data.vi" "Auto Gyro Hold"(TRUE ("Auto Gyro Hold")) -> ()
          n312 = global write "Robot Global Data.vi" "Auto Close Forks"(TRUE ("Auto Gyro Hold")) -> ()
          n313 = global write "Robot Global Data.vi" "Auto State"(3.0 ("Auto State")) -> ()
          n314 = Wait (ms)(milliseconds to wait=u32 500) -> ()  [unwired: 1 out]
        }
        frame #5 {
          # "Ensure at least 0.5sec wait"
          # "Lift up crate for 1500 counts"
          n315 = global write "Robot Global Data.vi" "Auto Joy 0 Axis X"(0.0 ("Auto Joy 0 Axis X")) -> ()
          n316 = global write "Robot Global Data.vi" "Auto Joy 0 Axis Y"(0.0 ("Auto Joy 0 Axis X")) -> ()
          n317 = global write "Robot Global Data.vi" "Auto Joy 0 Axis Z"(0.0 ("Auto Joy 0 Axis X")) -> ()
          n318 = global write "Robot Global Data.vi" "Auto Gyro Hold"(TRUE ("Auto Gyro Hold")) -> ()
          n319 = global write "Robot Global Data.vi" "Auto Close Forks"(FALSE ("Auto Gyro Hold")) -> ()
          n320 = while {
            stop <- w342 stop-if-true
            n321 = global read "Robot Global Data.vi" "Lift Stopped"() -> (w342:bool)
          }
          n322 = global write "Robot Global Data.vi" "Auto Lift Encoder"(1500.0 ("Auto Joy 0 Axis X")) -> ()
          n323 = Wait (ms)(milliseconds to wait=u32 500) -> ()  [unwired: 1 out]
          n324 = global write "Robot Global Data.vi" "Auto State"(4.0 ("Auto State")) -> ()
        }
        frame #6 {
          # "Drive backward until count = 1250"
          n325 = global write "Robot Global Data.vi" "Auto Joy 0 Axis X"(0.0 ("Auto Joy 0 Axis X")) -> ()
          n326 = global write "Robot Global Data.vi" "Auto Joy 0 Axis Y"(0.33 ("Auto Joy 0 Axis X")) -> ()
          n327 = global write "Robot Global Data.vi" "Auto Joy 0 Axis Z"(0.0 ("Auto Joy 0 Axis X")) -> ()
          n328 = global write "Robot Global Data.vi" "Auto Gyro Hold"(TRUE ("Auto Gyro Hold")) -> ()
          n329 = while {
            stop <- w350 stop-if-true
            n330 = global read "Robot Global Data.vi" "Wheel Encoder Distance"() -> (w348:dbl)
            n331 = Greater Or Equal?(x=w348, y=1250.0) -> (x >= y?=w350:bool)
          }
          n332 = global write "Robot Global Data.vi" "Auto State"(5.0 ("Auto State")) -> ()
        }
        frame #7 {
          # "100 is an inch above bottom limit switch\nNote: Trash Can keeps forks from engaing bottom limit\nswitch so use encoder!!!!"
          # "-200 is a dummy to get to bottom limit switch"
          # "Stop robot, lower crate"
          n333 = global write "Robot Global Data.vi" "Auto Joy 0 Axis X"(0.0 ("Auto Joy 0 Axis X")) -> ()
          n334 = global write "Robot Global Data.vi" "Auto Joy 0 Axis Y"(0.0 ("Auto Joy 0 Axis X")) -> ()
          n335 = global write "Robot Global Data.vi" "Auto Joy 0 Axis Z"(0.0 ("Auto Joy 0 Axis X")) -> ()
          n336 = global write "Robot Global Data.vi" "Auto Gyro Hold"(TRUE ("Auto Gyro Hold")) -> ()
          n337 = while {
            stop <- w357 stop-if-true
            n338 = global read "Robot Global Data.vi" "Lift Encoder Distance"() -> (w359:dbl)
            n339 = Less Or Equal?(x=w359, y=100.0) -> (x <= y?=w357:bool)
          }
          n340 = global write "Robot Global Data.vi" "Auto Lift Encoder"(-200.0 ("Auto Joy 0 Axis X")) -> ()
          n341 = global write "Robot Global Data.vi" "Auto State"(6.0 ("Auto State")) -> ()
        }
        frame #8 {
          # "Open lift, wait 0.5 sec for lift to open"
          n342 = global write "Robot Global Data.vi" "Auto Joy 0 Axis X"(0.0 ("Auto Joy 0 Axis X")) -> ()
          n343 = global write "Robot Global Data.vi" "Auto Joy 0 Axis Y"(0.0 ("Auto Joy 0 Axis X")) -> ()
          n344 = global write "Robot Global Data.vi" "Auto Joy 0 Axis Z"(0.0 ("Auto Joy 0 Axis X")) -> ()
          n345 = global write "Robot Global Data.vi" "Auto Gyro Hold"(TRUE ("Auto Gyro Hold")) -> ()
          n346 = global write "Robot Global Data.vi" "Auto Open Forks"(TRUE ("Auto Gyro Hold")) -> ()
          n347 = global write "Robot Global Data.vi" "Auto State"(7.0 ("Auto State")) -> ()
          n348 = Wait (ms)(milliseconds to wait=u32 500) -> ()  [unwired: 1 out]
        }
        frame #9 {
          # "Drive backward until count = 1500"
          n349 = global write "Robot Global Data.vi" "Auto Joy 0 Axis X"(0.0 ("Auto Joy 0 Axis X")) -> ()
          n350 = global write "Robot Global Data.vi" "Auto Joy 0 Axis Y"(0.3 ("Auto Joy 0 Axis X")) -> ()
          n351 = global write "Robot Global Data.vi" "Auto Joy 0 Axis Z"(0.0 ("Auto Joy 0 Axis X")) -> ()
          n352 = global write "Robot Global Data.vi" "Auto Gyro Hold"(TRUE ("Auto Gyro Hold")) -> ()
          n353 = global write "Robot Global Data.vi" "Auto Open Forks"(FALSE ("Auto Gyro Hold")) -> ()
          n354 = while {
            stop <- w375 stop-if-true
            n355 = global read "Robot Global Data.vi" "Wheel Encoder Distance"() -> (w374:dbl)
            n356 = Greater Or Equal?(x=w374, y=1500.0) -> (x >= y?=w375:bool)
          }
          n357 = global write "Robot Global Data.vi" "Auto State"(8.0 ("Auto State")) -> ()
        }
        frame #10 {
          # "Stop and wait until teleop"
          n358 = global write "Robot Global Data.vi" "Auto Joy 0 Axis X"(0.0 ("Auto Joy 0 Axis X")) -> ()
          n359 = global write "Robot Global Data.vi" "Auto Joy 0 Axis Y"(0.0 ("Auto Joy 0 Axis X")) -> ()
          n360 = global write "Robot Global Data.vi" "Auto Joy 0 Axis Z"(0.0 ("Auto Joy 0 Axis X")) -> ()
          n361 = global write "Robot Global Data.vi" "Auto Gyro Hold"(FALSE ("Auto Gyro Hold")) -> ()
          n362 = global write "Robot Global Data.vi" "Auto State"(9.0 ("Auto State")) -> ()
          n363 = Wait (ms)(milliseconds to wait=u32 15000) -> ()  [unwired: 1 out]
        }
      }
    }
  }
  n364 = case shown="True" w30 {
    frame False {
    }
    frame True {
      n365 = stacked-sequence {
        frame #0 {
          # "Reset encoders"
          # "Reset Gyro"
          # "Initialize"
          n366 = global write "Robot Global Data.vi" "Auto Joy 1 Axis Y"(0.0 ("Auto Joy 0 Axis X")) -> ()
          n367 = global write "Robot Global Data.vi" "Auto Joy 0 Axis X"(0.0 ("Auto Joy 0 Axis X")) -> ()
          n368 = global write "Robot Global Data.vi" "Auto Joy 0 Axis Y"(0.0 ("Auto Joy 0 Axis X")) -> ()
          n369 = global write "Robot Global Data.vi" "Auto Joy 0 Axis Z"(0.0 ("Auto Joy 0 Axis X")) -> ()
          n370 = global write "Robot Global Data.vi" "Gyro Reset"(TRUE ("Auto Gyro Hold")) -> ()
          n371 = global write "Robot Global Data.vi" "Lift Encoder Reset"(TRUE ("Auto Gyro Hold")) -> ()
          n372 = global write "Robot Global Data.vi" "Wheel Encoder Reset"(TRUE ("Wheel Encoder Reset")) -> ()
          n373 = global write "Robot Global Data.vi" "Auto Gyro Hold"(FALSE ("Auto Gyro Hold")) -> ()
          n374 = global write "Robot Global Data.vi" "Auto Open Forks"(FALSE ("Auto Gyro Hold")) -> ()
          n375 = global write "Robot Global Data.vi" "Auto Close Forks"(FALSE ("Auto Gyro Hold")) -> ()
          n376 = global write "Robot Global Data.vi" "PID Target Angle"(0.0 ("Auto Joy 0 Axis Z")) -> ()
          n377 = global write "Robot Global Data.vi" "Raw Gyro Angle"(0.0 ("Auto Joy 0 Axis Z")) -> ()
          n378 = global write "Robot Global Data.vi" "Auto State"(0.0 ("Auto State")) -> ()
          n379 = Wait (ms)(milliseconds to wait=u32 50) -> ()  [unwired: 1 out]
        }
        frame #1 {
          # "Reset encoders"
          # "Reset Gyro"
          # "Initialize"
          n380 = global write "Robot Global Data.vi" "Auto Joy 0 Axis X"(0.0 ("Auto Joy 0 Axis X")) -> ()
          n381 = global write "Robot Global Data.vi" "Auto Joy 0 Axis Y"(0.0 ("Auto Joy 0 Axis X")) -> ()
          n382 = global write "Robot Global Data.vi" "Auto Joy 0 Axis Z"(0.0 ("Auto Joy 0 Axis X")) -> ()
          n383 = global write "Robot Global Data.vi" "Gyro Reset"(FALSE ("Auto Gyro Hold")) -> ()
          n384 = global write "Robot Global Data.vi" "Lift Encoder Reset"(FALSE ("Auto Gyro Hold")) -> ()
          n385 = global write "Robot Global Data.vi" "Wheel Encoder Reset"(FALSE ("Wheel Encoder Reset")) -> ()
          n386 = global write "Robot Global Data.vi" "Auto State"(0.0 ("Auto State")) -> ()
          n387 = Wait (ms)(milliseconds to wait=u32 50) -> ()  [unwired: 1 out]
        }
        frame #2 {
          # "Lock Gyro"
          # "Drive forward for 50 counts"
          n388 = global write "Robot Global Data.vi" "Auto Joy 0 Axis X"(0.0 ("Auto Joy 0 Axis X")) -> ()
          n389 = global write "Robot Global Data.vi" "Auto Joy 0 Axis Y"(-0.25 ("Auto Joy 0 Axis X")) -> ()
          n390 = global write "Robot Global Data.vi" "Auto Joy 0 Axis Z"(0.0 ("Auto Joy 0 Axis X")) -> ()
          n391 = global write "Robot Global Data.vi" "Auto Gyro Hold"(TRUE ("Auto Gyro Hold")) -> ()
          n392 = global write "Robot Global Data.vi" "Lift Encoder Reset"(FALSE ("Auto Gyro Hold")) -> ()
          n393 = global write "Robot Global Data.vi" "Wheel Encoder Reset"(FALSE ("Wheel Encoder Reset")) -> ()
          n394 = while {
            stop <- w411 stop-if-true
            n395 = global read "Robot Global Data.vi" "Wheel Encoder Distance"() -> (w413:dbl)
            n396 = Less Or Equal?(x=w413, y=-50.0) -> (x <= y?=w411:bool)
          }
          n397 = global write "Robot Global Data.vi" "Auto State"(1.0 ("Auto State")) -> ()
        }
        frame #3 {
          # "Stop robot and wait 0.1 sec"
          n398 = global write "Robot Global Data.vi" "Auto Joy 0 Axis X"(0.0 ("Auto Joy 0 Axis X")) -> ()
          n399 = global write "Robot Global Data.vi" "Auto Joy 0 Axis Y"(0.0 ("Auto Joy 0 Axis X")) -> ()
          n400 = global write "Robot Global Data.vi" "Auto Joy 0 Axis Z"(0.0 ("Auto Joy 0 Axis X")) -> ()
          n401 = global write "Robot Global Data.vi" "Auto Gyro Hold"(TRUE ("Auto Gyro Hold")) -> ()
          n402 = global write "Robot Global Data.vi" "Auto State"(2.0 ("Auto State")) -> ()
          n403 = Wait (ms)(milliseconds to wait=u32 100) -> ()  [unwired: 1 out]
        }
        frame #4 {
          # "Close lift, wait 0.5 sec for lift to close"
          n404 = global write "Robot Global Data.vi" "Auto Joy 0 Axis X"(0.0 ("Auto Joy 0 Axis X")) -> ()
          n405 = global write "Robot Global Data.vi" "Auto Joy 0 Axis Y"(0.0 ("Auto Joy 0 Axis X")) -> ()
          n406 = global write "Robot Global Data.vi" "Auto Joy 0 Axis Z"(0.0 ("Auto Joy 0 Axis X")) -> ()
          n407 = global write "Robot Global Data.vi" "Auto Gyro Hold"(TRUE ("Auto Gyro Hold")) -> ()
          n408 = global write "Robot Global Data.vi" "Auto Close Forks"(TRUE ("Auto Gyro Hold")) -> ()
          n409 = global write "Robot Global Data.vi" "Auto State"(3.0 ("Auto State")) -> ()
          n410 = Wait (ms)(milliseconds to wait=u32 500) -> ()  [unwired: 1 out]
        }
        frame #5 {
          # "Ensure at least 0.5sec wait"
          # "Lift up crate for 2500 counts"
          n411 = global write "Robot Global Data.vi" "Auto Joy 0 Axis X"(0.0 ("Auto Joy 0 Axis X")) -> ()
          n412 = global write "Robot Global Data.vi" "Auto Joy 0 Axis Y"(0.0 ("Auto Joy 0 Axis X")) -> ()
          n413 = global write "Robot Global Data.vi" "Auto Joy 0 Axis Z"(0.0 ("Auto Joy 0 Axis X")) -> ()
          n414 = global write "Robot Global Data.vi" "Auto Gyro Hold"(TRUE ("Auto Gyro Hold")) -> ()
          n415 = global write "Robot Global Data.vi" "Auto Close Forks"(FALSE ("Auto Gyro Hold")) -> ()
          n416 = while {
            stop <- w435 stop-if-true
            n417 = global read "Robot Global Data.vi" "Lift Stopped"() -> (w435:bool)
          }
          n418 = global write "Robot Global Data.vi" "Auto Lift Encoder"(2500.0 ("Auto Joy 0 Axis X")) -> ()
          n419 = Wait (ms)(milliseconds to wait=u32 500) -> ()  [unwired: 1 out]
          n420 = global write "Robot Global Data.vi" "Auto State"(4.0 ("Auto State")) -> ()
        }
        frame #6 {
          # "Wait for robot to finish turning"
          # "Turn robot 90 degrees clockwise"
          n421 = global write "Robot Global Data.vi" "Auto Joy 0 Axis X"(0.0 ("Auto Joy 0 Axis X")) -> ()
          n422 = global write "Robot Global Data.vi" "Auto Joy 0 Axis Y"(0.0 ("Auto Joy 0 Axis X")) -> ()
          n423 = global write "Robot Global Data.vi" "Auto Joy 0 Axis Z"(0.0 ("Auto Joy 0 Axis X")) -> ()
          n424 = global write "Robot Global Data.vi" "Auto Gyro Hold"(TRUE ("Auto Gyro Hold")) -> ()
          n425 = global write "Robot Global Data.vi" "PID Target Angle"(90.0 ("Auto Joy 0 Axis Z")) -> ()
          n426 = global write "Robot Global Data.vi" "Auto State"(5.0 ("Auto State")) -> ()
          n427 = Wait (ms)(milliseconds to wait=u32 2000) -> ()  [unwired: 1 out]
        }
        frame #7 {
          # "Reset wheel counter since robot turned,\nhence forward count is incorrect."
          n428 = global write "Robot Global Data.vi" "Auto Joy 0 Axis X"(0.0 ("Auto Joy 0 Axis X")) -> ()
          n429 = global write "Robot Global Data.vi" "Auto Joy 0 Axis Y"(0.0 ("Auto Joy 0 Axis X")) -> ()
          n430 = global write "Robot Global Data.vi" "Auto Joy 0 Axis Z"(0.0 ("Auto Joy 0 Axis X")) -> ()
          n431 = global write "Robot Global Data.vi" "Auto Gyro Hold"(TRUE ("Auto Gyro Hold")) -> ()
          n432 = global write "Robot Global Data.vi" "Wheel Encoder Reset"(TRUE ("Wheel Encoder Reset")) -> ()
          n433 = global write "Robot Global Data.vi" "Auto State"(6.0 ("Auto State")) -> ()
          n434 = Wait (ms)(milliseconds to wait=u32 50) -> ()  [unwired: 1 out]
        }
        frame #8 {
          # "Enable wheel counter."
          n435 = global write "Robot Global Data.vi" "Auto Joy 0 Axis X"(0.0 ("Auto Joy 0 Axis X")) -> ()
          n436 = global write "Robot Global Data.vi" "Auto Joy 0 Axis Y"(0.0 ("Auto Joy 0 Axis X")) -> ()
          n437 = global write "Robot Global Data.vi" "Auto Joy 0 Axis Z"(0.0 ("Auto Joy 0 Axis X")) -> ()
          n438 = global write "Robot Global Data.vi" "Auto Gyro Hold"(TRUE ("Auto Gyro Hold")) -> ()
          n439 = global write "Robot Global Data.vi" "Wheel Encoder Reset"(FALSE ("Wheel Encoder Reset")) -> ()
          n440 = global write "Robot Global Data.vi" "Auto State"(7.0 ("Auto State")) -> ()
          n441 = Wait (ms)(milliseconds to wait=u32 50) -> ()  [unwired: 1 out]
        }
        frame #9 {
          # "Drive forward until count = -1650"
          n442 = global write "Robot Global Data.vi" "Auto Joy 0 Axis X"(0.0 ("Auto Joy 0 Axis X")) -> ()
          n443 = global write "Robot Global Data.vi" "Auto Joy 0 Axis Y"(-0.33 ("Auto Joy 0 Axis X")) -> ()
          n444 = global write "Robot Global Data.vi" "Auto Joy 0 Axis Z"(0.0 ("Auto Joy 0 Axis X")) -> ()
          n445 = global write "Robot Global Data.vi" "Auto Gyro Hold"(TRUE ("Auto Gyro Hold")) -> ()
          n446 = global write "Robot Global Data.vi" "Wheel Encoder Reset"(FALSE ("Wheel Encoder Reset")) -> ()
          n447 = while {
            stop <- w465 stop-if-true
            n448 = global read "Robot Global Data.vi" "Wheel Encoder Distance"() -> (w464:dbl)
            n449 = Less Or Equal?(x=w464, y=-1650.0) -> (x <= y?=w465:bool)
          }
          n450 = global write "Robot Global Data.vi" "Auto State"(8.0 ("Auto State")) -> ()
        }
        frame #10 {
          # "100 is an inch above bottom limit switch\nNote: Trash Can keeps forks from engaing bottom limit\nswitch so use encoder!!!!"
          # "-200 is a dummy to get to bottom limit switch"
          # "Stop robot, lower crate"
          n451 = global write "Robot Global Data.vi" "Auto Joy 0 Axis X"(0.0 ("Auto Joy 0 Axis X")) -> ()
          n452 = global write "Robot Global Data.vi" "Auto Joy 0 Axis Y"(0.0 ("Auto Joy 0 Axis X")) -> ()
          n453 = global write "Robot Global Data.vi" "Auto Joy 0 Axis Z"(0.0 ("Auto Joy 0 Axis X")) -> ()
          n454 = global write "Robot Global Data.vi" "Auto Gyro Hold"(TRUE ("Auto Gyro Hold")) -> ()
          n455 = while {
            stop <- w472 stop-if-true
            n456 = global read "Robot Global Data.vi" "Lift Encoder Distance"() -> (w474:dbl)
            n457 = Less Or Equal?(x=w474, y=100.0) -> (x <= y?=w472:bool)
          }
          n458 = global write "Robot Global Data.vi" "Auto Lift Encoder"(-200.0 ("Auto Joy 0 Axis X")) -> ()
          n459 = global write "Robot Global Data.vi" "Auto State"(9.0 ("Auto State")) -> ()
        }
        frame #11 {
          # "Open lift, wait 0.5 sec for lift to open"
          n460 = global write "Robot Global Data.vi" "Auto Joy 0 Axis X"(0.0 ("Auto Joy 0 Axis X")) -> ()
          n461 = global write "Robot Global Data.vi" "Auto Joy 0 Axis Y"(0.0 ("Auto Joy 0 Axis X")) -> ()
          n462 = global write "Robot Global Data.vi" "Auto Joy 0 Axis Z"(0.0 ("Auto Joy 0 Axis X")) -> ()
          n463 = global write "Robot Global Data.vi" "Auto Gyro Hold"(TRUE ("Auto Gyro Hold")) -> ()
          n464 = global write "Robot Global Data.vi" "Auto Open Forks"(TRUE ("Auto Gyro Hold")) -> ()
          n465 = global write "Robot Global Data.vi" "Auto State"(10.0 ("Auto State")) -> ()
          n466 = Wait (ms)(milliseconds to wait=u32 500) -> ()  [unwired: 1 out]
        }
        frame #12 {
          # "Drive backward until count = -1800"
          n467 = global write "Robot Global Data.vi" "Auto Joy 0 Axis X"(0.0 ("Auto Joy 0 Axis X")) -> ()
          n468 = global write "Robot Global Data.vi" "Auto Joy 0 Axis Y"(0.25 ("Auto Joy 0 Axis X")) -> ()
          n469 = global write "Robot Global Data.vi" "Auto Joy 0 Axis Z"(0.0 ("Auto Joy 0 Axis X")) -> ()
          n470 = global write "Robot Global Data.vi" "Auto Gyro Hold"(TRUE ("Auto Gyro Hold")) -> ()
          n471 = global write "Robot Global Data.vi" "Auto Open Forks"(FALSE ("Auto Gyro Hold")) -> ()
          n472 = while {
            stop <- w490 stop-if-true
            n473 = global read "Robot Global Data.vi" "Wheel Encoder Distance"() -> (w489:dbl)
            n474 = Greater Or Equal?(x=w489, y=-1800.0) -> (x >= y?=w490:bool)
          }
          n475 = global write "Robot Global Data.vi" "Auto State"(11.0 ("Auto State")) -> ()
        }
        frame #13 {
          # "Stop and wait until teleop"
          n476 = global write "Robot Global Data.vi" "Auto Joy 0 Axis X"(0.0 ("Auto Joy 0 Axis X")) -> ()
          n477 = global write "Robot Global Data.vi" "Auto Joy 0 Axis Y"(0.0 ("Auto Joy 0 Axis X")) -> ()
          n478 = global write "Robot Global Data.vi" "Auto Joy 0 Axis Z"(0.0 ("Auto Joy 0 Axis X")) -> ()
          n479 = global write "Robot Global Data.vi" "Auto Gyro Hold"(FALSE ("Auto Gyro Hold")) -> ()
          n480 = global write "Robot Global Data.vi" "Auto State"(12.0 ("Auto State")) -> ()
          n481 = Wait (ms)(milliseconds to wait=u32 15000) -> ()  [unwired: 1 out]
        }
      }
    }
  }
  n482 = case shown="True" w22 {
    frame False {
    }
    frame True {
      n483 = stacked-sequence {
        frame #0 {
          # "Reset encoders"
          # "Reset Gyro"
          # "Initialize"
          n484 = global write "Robot Global Data.vi" "Auto Joy 1 Axis Y"(0.0 ("Auto Joy 0 Axis X")) -> ()
          n485 = global write "Robot Global Data.vi" "Auto Joy 0 Axis X"(0.0 ("Auto Joy 0 Axis X")) -> ()
          n486 = global write "Robot Global Data.vi" "Auto Joy 0 Axis Y"(0.0 ("Auto Joy 0 Axis X")) -> ()
          n487 = global write "Robot Global Data.vi" "Auto Joy 0 Axis Z"(0.0 ("Auto Joy 0 Axis X")) -> ()
          n488 = global write "Robot Global Data.vi" "Gyro Reset"(TRUE ("Auto Gyro Hold")) -> ()
          n489 = global write "Robot Global Data.vi" "Lift Encoder Reset"(TRUE ("Auto Gyro Hold")) -> ()
          n490 = global write "Robot Global Data.vi" "Wheel Encoder Reset"(TRUE ("Wheel Encoder Reset")) -> ()
          n491 = global write "Robot Global Data.vi" "Auto Open Forks"(FALSE ("Auto Gyro Hold")) -> ()
          n492 = global write "Robot Global Data.vi" "Auto Gyro Hold"(FALSE ("Auto Gyro Hold")) -> ()
          n493 = global write "Robot Global Data.vi" "Auto Close Forks"(FALSE ("Auto Gyro Hold")) -> ()
          n494 = global write "Robot Global Data.vi" "PID Target Angle"(0.0 ("Auto Joy 0 Axis Z")) -> ()
          n495 = global write "Robot Global Data.vi" "Raw Gyro Angle"(0.0 ("Auto Joy 0 Axis Z")) -> ()
          n496 = global write "Robot Global Data.vi" "Auto State"(0.0 ("Auto State")) -> ()
          n497 = Wait (ms)(milliseconds to wait=u32 50) -> ()  [unwired: 1 out]
        }
        frame #1 {
          # "Reset encoders"
          # "Reset Gyro"
          # "Initialize"
          n498 = global write "Robot Global Data.vi" "Auto Joy 0 Axis X"(0.0 ("Auto Joy 0 Axis X")) -> ()
          n499 = global write "Robot Global Data.vi" "Auto Joy 0 Axis Y"(0.0 ("Auto Joy 0 Axis X")) -> ()
          n500 = global write "Robot Global Data.vi" "Auto Joy 0 Axis Z"(0.0 ("Auto Joy 0 Axis X")) -> ()
          n501 = global write "Robot Global Data.vi" "Gyro Reset"(FALSE ("Auto Gyro Hold")) -> ()
          n502 = global write "Robot Global Data.vi" "Lift Encoder Reset"(FALSE ("Auto Gyro Hold")) -> ()
          n503 = global write "Robot Global Data.vi" "Wheel Encoder Reset"(FALSE ("Wheel Encoder Reset")) -> ()
          n504 = global write "Robot Global Data.vi" "Auto State"(0.0 ("Auto State")) -> ()
          n505 = Wait (ms)(milliseconds to wait=u32 50) -> ()  [unwired: 1 out]
        }
        frame #2 {
          # "Drive forward for 50 counts"
          n506 = global write "Robot Global Data.vi" "Auto Joy 0 Axis X"(0.0 ("Auto Joy 0 Axis X")) -> ()
          n507 = global write "Robot Global Data.vi" "Auto Joy 0 Axis Y"(-0.25 ("Auto Joy 0 Axis X")) -> ()
          n508 = global write "Robot Global Data.vi" "Auto Joy 0 Axis Z"(0.0 ("Auto Joy 0 Axis X")) -> ()
          n509 = global write "Robot Global Data.vi" "Auto Gyro Hold"(TRUE ("Auto Gyro Hold")) -> ()
          n510 = global write "Robot Global Data.vi" "Lift Encoder Reset"(FALSE ("Auto Gyro Hold")) -> ()
          n511 = global write "Robot Global Data.vi" "Wheel Encoder Reset"(FALSE ("Wheel Encoder Reset")) -> ()
          n512 = while {
            stop <- w526 stop-if-true
            n513 = global read "Robot Global Data.vi" "Wheel Encoder Distance"() -> (w528:dbl)
            n514 = Less Or Equal?(x=w528, y=-50.0) -> (x <= y?=w526:bool)
          }
          n515 = global write "Robot Global Data.vi" "Auto State"(1.0 ("Auto State")) -> ()
        }
        frame #3 {
          # "Stop robot and wait 0.1 sec"
          n516 = global write "Robot Global Data.vi" "Auto Joy 0 Axis X"(0.0 ("Auto Joy 0 Axis X")) -> ()
          n517 = global write "Robot Global Data.vi" "Auto Joy 0 Axis Y"(0.0 ("Auto Joy 0 Axis X")) -> ()
          n518 = global write "Robot Global Data.vi" "Auto Joy 0 Axis Z"(0.0 ("Auto Joy 0 Axis X")) -> ()
          n519 = global write "Robot Global Data.vi" "Auto Gyro Hold"(TRUE ("Auto Gyro Hold")) -> ()
          n520 = global write "Robot Global Data.vi" "Auto State"(2.0 ("Auto State")) -> ()
          n521 = Wait (ms)(milliseconds to wait=u32 100) -> ()  [unwired: 1 out]
        }
        frame #4 {
          # "Close lift, wait 0.5 sec for lift to close"
          n522 = global write "Robot Global Data.vi" "Auto Joy 0 Axis X"(0.0 ("Auto Joy 0 Axis X")) -> ()
          n523 = global write "Robot Global Data.vi" "Auto Joy 0 Axis Y"(0.0 ("Auto Joy 0 Axis X")) -> ()
          n524 = global write "Robot Global Data.vi" "Auto Joy 0 Axis Z"(0.0 ("Auto Joy 0 Axis X")) -> ()
          n525 = global write "Robot Global Data.vi" "Auto Gyro Hold"(TRUE ("Auto Gyro Hold")) -> ()
          n526 = global write "Robot Global Data.vi" "Auto Close Forks"(TRUE ("Auto Gyro Hold")) -> ()
          n527 = global write "Robot Global Data.vi" "Auto State"(3.0 ("Auto State")) -> ()
          n528 = Wait (ms)(milliseconds to wait=u32 500) -> ()  [unwired: 1 out]
        }
        frame #5 {
          # "Ensure at least 0.5sec wait"
          # "Lift up crate for 2500 counts"
          n529 = global write "Robot Global Data.vi" "Auto Joy 0 Axis X"(0.0 ("Auto Joy 0 Axis X")) -> ()
          n530 = global write "Robot Global Data.vi" "Auto Joy 0 Axis Y"(0.0 ("Auto Joy 0 Axis X")) -> ()
          n531 = global write "Robot Global Data.vi" "Auto Joy 0 Axis Z"(0.0 ("Auto Joy 0 Axis X")) -> ()
          n532 = global write "Robot Global Data.vi" "Auto Gyro Hold"(TRUE ("Auto Gyro Hold")) -> ()
          n533 = global write "Robot Global Data.vi" "Auto Close Forks"(FALSE ("Auto Gyro Hold")) -> ()
          n534 = while {
            stop <- w550 stop-if-true
            n535 = global read "Robot Global Data.vi" "Lift Stopped"() -> (w550:bool)
          }
          n536 = global write "Robot Global Data.vi" "Auto Lift Encoder"(2500.0 ("Auto Joy 0 Axis X")) -> ()
          n537 = Wait (ms)(milliseconds to wait=u32 500) -> ()  [unwired: 1 out]
          n538 = global write "Robot Global Data.vi" "Auto State"(4.0 ("Auto State")) -> ()
        }
        frame #6 {
          # "Wait for robot to finish turning"
          # "Turn robot 90 degrees clockwise"
          n539 = global write "Robot Global Data.vi" "Auto Joy 0 Axis X"(0.0 ("Auto Joy 0 Axis X")) -> ()
          n540 = global write "Robot Global Data.vi" "Auto Joy 0 Axis Y"(0.0 ("Auto Joy 0 Axis X")) -> ()
          n541 = global write "Robot Global Data.vi" "Auto Joy 0 Axis Z"(0.0 ("Auto Joy 0 Axis X")) -> ()
          n542 = global write "Robot Global Data.vi" "Auto Gyro Hold"(TRUE ("Auto Gyro Hold")) -> ()
          n543 = global write "Robot Global Data.vi" "PID Target Angle"(-90.0 ("Auto Joy 0 Axis Z")) -> ()
          n544 = global write "Robot Global Data.vi" "Auto State"(5.0 ("Auto State")) -> ()
          n545 = Wait (ms)(milliseconds to wait=u32 2000) -> ()  [unwired: 1 out]
        }
        frame #7 {
          # "Reset wheel counter since robot turned,\nhence forward count is incorrect."
          n546 = global write "Robot Global Data.vi" "Auto Joy 0 Axis X"(0.0 ("Auto Joy 0 Axis X")) -> ()
          n547 = global write "Robot Global Data.vi" "Auto Joy 0 Axis Y"(0.0 ("Auto Joy 0 Axis X")) -> ()
          n548 = global write "Robot Global Data.vi" "Auto Joy 0 Axis Z"(0.0 ("Auto Joy 0 Axis X")) -> ()
          n549 = global write "Robot Global Data.vi" "Auto Gyro Hold"(TRUE ("Auto Gyro Hold")) -> ()
          n550 = global write "Robot Global Data.vi" "Wheel Encoder Reset"(TRUE ("Wheel Encoder Reset")) -> ()
          n551 = global write "Robot Global Data.vi" "Auto State"(6.0 ("Auto State")) -> ()
          n552 = Wait (ms)(milliseconds to wait=u32 50) -> ()  [unwired: 1 out]
        }
        frame #8 {
          # "Enable wheel counter."
          n553 = global write "Robot Global Data.vi" "Auto Joy 0 Axis X"(0.0 ("Auto Joy 0 Axis X")) -> ()
          n554 = global write "Robot Global Data.vi" "Auto Joy 0 Axis Y"(0.0 ("Auto Joy 0 Axis X")) -> ()
          n555 = global write "Robot Global Data.vi" "Auto Joy 0 Axis Z"(0.0 ("Auto Joy 0 Axis X")) -> ()
          n556 = global write "Robot Global Data.vi" "Auto Gyro Hold"(TRUE ("Auto Gyro Hold")) -> ()
          n557 = global write "Robot Global Data.vi" "Wheel Encoder Reset"(FALSE ("Wheel Encoder Reset")) -> ()
          n558 = global write "Robot Global Data.vi" "Auto State"(7.0 ("Auto State")) -> ()
          n559 = Wait (ms)(milliseconds to wait=u32 50) -> ()  [unwired: 1 out]
        }
        frame #9 {
          # "Drive forward until count = -1750"
          n560 = global write "Robot Global Data.vi" "Auto Joy 0 Axis X"(0.0 ("Auto Joy 0 Axis X")) -> ()
          n561 = global write "Robot Global Data.vi" "Auto Joy 0 Axis Y"(-0.33 ("Auto Joy 0 Axis X")) -> ()
          n562 = global write "Robot Global Data.vi" "Auto Joy 0 Axis Z"(0.0 ("Auto Joy 0 Axis X")) -> ()
          n563 = global write "Robot Global Data.vi" "Auto Gyro Hold"(TRUE ("Auto Gyro Hold")) -> ()
          n564 = global write "Robot Global Data.vi" "Wheel Encoder Reset"(FALSE ("Wheel Encoder Reset")) -> ()
          n565 = while {
            stop <- w580 stop-if-true
            n566 = global read "Robot Global Data.vi" "Wheel Encoder Distance"() -> (w579:dbl)
            n567 = Less Or Equal?(x=w579, y=-1750.0) -> (x <= y?=w580:bool)
          }
          n568 = global write "Robot Global Data.vi" "Auto State"(8.0 ("Auto State")) -> ()
        }
        frame #10 {
          # "100 is an inch above bottom limit switch\nNote: Trash Can keeps forks from engaing bottom limit\nswitch so use encoder!!!!"
          # "Stop robot, lower crate"
          n569 = global write "Robot Global Data.vi" "Auto Joy 0 Axis X"(0.0 ("Auto Joy 0 Axis X")) -> ()
          n570 = global write "Robot Global Data.vi" "Auto Joy 0 Axis Y"(0.0 ("Auto Joy 0 Axis X")) -> ()
          n571 = global write "Robot Global Data.vi" "Auto Joy 0 Axis Z"(0.0 ("Auto Joy 0 Axis X")) -> ()
          n572 = global write "Robot Global Data.vi" "Auto Gyro Hold"(TRUE ("Auto Gyro Hold")) -> ()
          n573 = while {
            stop <- w587 stop-if-true
            n574 = global read "Robot Global Data.vi" "Lift Encoder Distance"() -> (w589:dbl)
            n575 = Less Or Equal?(x=w589, y=100.0) -> (x <= y?=w587:bool)
          }
          n576 = global write "Robot Global Data.vi" "Auto Lift Encoder"(-200.0 ("Auto Joy 0 Axis X")) -> ()
          n577 = global write "Robot Global Data.vi" "Auto State"(9.0 ("Auto State")) -> ()
        }
        frame #11 {
          # "Open lift, wait 0.5 sec for lift to open"
          n578 = global write "Robot Global Data.vi" "Auto Joy 0 Axis X"(0.0 ("Auto Joy 0 Axis X")) -> ()
          n579 = global write "Robot Global Data.vi" "Auto Joy 0 Axis Y"(0.0 ("Auto Joy 0 Axis X")) -> ()
          n580 = global write "Robot Global Data.vi" "Auto Joy 0 Axis Z"(0.0 ("Auto Joy 0 Axis X")) -> ()
          n581 = global write "Robot Global Data.vi" "Auto Gyro Hold"(TRUE ("Auto Gyro Hold")) -> ()
          n582 = global write "Robot Global Data.vi" "Auto Open Forks"(TRUE ("Auto Gyro Hold")) -> ()
          n583 = global write "Robot Global Data.vi" "Auto State"(10.0 ("Auto State")) -> ()
          n584 = Wait (ms)(milliseconds to wait=u32 500) -> ()  [unwired: 1 out]
        }
        frame #12 {
          # "Drive backward until count = -1850"
          n585 = global write "Robot Global Data.vi" "Auto Joy 0 Axis X"(0.0 ("Auto Joy 0 Axis X")) -> ()
          n586 = global write "Robot Global Data.vi" "Auto Joy 0 Axis Y"(0.25 ("Auto Joy 0 Axis X")) -> ()
          n587 = global write "Robot Global Data.vi" "Auto Joy 0 Axis Z"(0.0 ("Auto Joy 0 Axis X")) -> ()
          n588 = global write "Robot Global Data.vi" "Auto Gyro Hold"(TRUE ("Auto Gyro Hold")) -> ()
          n589 = global write "Robot Global Data.vi" "Auto Open Forks"(FALSE ("Auto Gyro Hold")) -> ()
          n590 = while {
            stop <- w605 stop-if-true
            n591 = global read "Robot Global Data.vi" "Wheel Encoder Distance"() -> (w604:dbl)
            n592 = Greater Or Equal?(x=w604, y=-1850.0) -> (x >= y?=w605:bool)
          }
          n593 = global write "Robot Global Data.vi" "Auto State"(11.0 ("Auto State")) -> ()
        }
        frame #13 {
          # "Stop and wait until teleop"
          n594 = global write "Robot Global Data.vi" "Auto Joy 0 Axis X"(0.0 ("Auto Joy 0 Axis X")) -> ()
          n595 = global write "Robot Global Data.vi" "Auto Joy 0 Axis Y"(0.0 ("Auto Joy 0 Axis X")) -> ()
          n596 = global write "Robot Global Data.vi" "Auto Joy 0 Axis Z"(0.0 ("Auto Joy 0 Axis X")) -> ()
          n597 = global write "Robot Global Data.vi" "Auto Gyro Hold"(FALSE ("Auto Gyro Hold")) -> ()
          n598 = global write "Robot Global Data.vi" "Auto State"(12.0 ("Auto State")) -> ()
          n599 = Wait (ms)(milliseconds to wait=u32 15000) -> ()  [unwired: 1 out]
        }
      }
    }
  }
  n600 = case shown="True" w27 {
    frame False {
    }
    frame True {
      n601 = stacked-sequence {
        frame #0 {
          # "Reset encoders"
          # "Reset Gyro"
          # "Initialize"
          n602 = global write "Robot Global Data.vi" "Auto Joy 0 Axis X"(0.0 ("Auto Joy 0 Axis X")) -> ()
          n603 = global write "Robot Global Data.vi" "Auto Joy 0 Axis Y"(0.0 ("Auto Joy 0 Axis X")) -> ()
          n604 = global write "Robot Global Data.vi" "Auto Joy 0 Axis Z"(0.0 ("Auto Joy 0 Axis X")) -> ()
          n605 = global write "Robot Global Data.vi" "Auto Joy 1 Axis Y"(0.0 ("Auto Joy 0 Axis X")) -> ()
          n606 = global write "Robot Global Data.vi" "Lift Encoder Reset"(TRUE ("Auto Gyro Hold")) -> ()
          n607 = global write "Robot Global Data.vi" "Wheel Encoder Reset"(TRUE ("Wheel Encoder Reset")) -> ()
          n608 = global write "Robot Global Data.vi" "Auto Gyro Hold"(FALSE ("Auto Gyro Hold")) -> ()
          n609 = global write "Robot Global Data.vi" "Gyro Reset"(TRUE ("Auto Gyro Hold")) -> ()
          n610 = global write "Robot Global Data.vi" "Auto Open Forks"(FALSE ("Auto Gyro Hold")) -> ()
          n611 = global write "Robot Global Data.vi" "Auto Close Forks"(FALSE ("Auto Gyro Hold")) -> ()
          n612 = global write "Robot Global Data.vi" "PID Target Angle"(0.0 ("Auto Joy 0 Axis Z")) -> ()
          n613 = global write "Robot Global Data.vi" "Raw Gyro Angle"(0.0 ("Auto Joy 0 Axis Z")) -> ()
          n614 = global write "Robot Global Data.vi" "Auto State"(0.0 ("Auto State")) -> ()
          n615 = Wait (ms)(milliseconds to wait=u32 50) -> ()  [unwired: 1 out]
        }
        frame #1 {
          # "Initialize"
          n616 = global write "Robot Global Data.vi" "Auto Joy 0 Axis X"(0.0 ("Auto Joy 0 Axis X")) -> ()
          n617 = global write "Robot Global Data.vi" "Auto Joy 0 Axis Y"(0.0 ("Auto Joy 0 Axis X")) -> ()
          n618 = global write "Robot Global Data.vi" "Auto Joy 0 Axis Z"(0.0 ("Auto Joy 0 Axis X")) -> ()
          n619 = global write "Robot Global Data.vi" "Lift Encoder Reset"(FALSE ("Auto Gyro Hold")) -> ()
          n620 = global write "Robot Global Data.vi" "Wheel Encoder Reset"(FALSE ("Wheel Encoder Reset")) -> ()
          n621 = global write "Robot Global Data.vi" "Gyro Reset"(FALSE ("Auto Gyro Hold")) -> ()
          n622 = global write "Robot Global Data.vi" "Auto State"(0.0 ("Auto State")) -> ()
          n623 = Wait (ms)(milliseconds to wait=u32 50) -> ()  [unwired: 1 out]
        }
        frame #2 {
          # "Lock Gyro"
          # "Drive forward for 300 counts"
          n624 = global write "Robot Global Data.vi" "Auto Joy 0 Axis X"(0.0 ("Auto Joy 0 Axis X")) -> ()
          n625 = global write "Robot Global Data.vi" "Auto Joy 0 Axis Y"(-0.25 ("Auto Joy 0 Axis X")) -> ()
          n626 = global write "Robot Global Data.vi" "Auto Joy 0 Axis Z"(0.0 ("Auto Joy 0 Axis X")) -> ()
          n627 = global write "Robot Global Data.vi" "Auto Gyro Hold"(TRUE ("Auto Gyro Hold")) -> ()
          n628 = global write "Robot Global Data.vi" "Lift Encoder Reset"(FALSE ("Auto Gyro Hold")) -> ()
          n629 = global write "Robot Global Data.vi" "Wheel Encoder Reset"(FALSE ("Wheel Encoder Reset")) -> ()
          n630 = while {
            stop <- w641 stop-if-true
            n631 = global read "Robot Global Data.vi" "Wheel Encoder Distance"() -> (w643:dbl)
            n632 = Less Or Equal?(x=w643, y=-300.0) -> (x <= y?=w641:bool)
          }
          n633 = global write "Robot Global Data.vi" "Auto State"(1.0 ("Auto State")) -> ()
        }
        frame #3 {
          # "Stop robot and wait 0.1 sec"
          n634 = global write "Robot Global Data.vi" "Auto Joy 0 Axis X"(0.0 ("Auto Joy 0 Axis X")) -> ()
          n635 = global write "Robot Global Data.vi" "Auto Joy 0 Axis Y"(0.0 ("Auto Joy 0 Axis X")) -> ()
          n636 = global write "Robot Global Data.vi" "Auto Joy 0 Axis Z"(0.0 ("Auto Joy 0 Axis X")) -> ()
          n637 = global write "Robot Global Data.vi" "Auto Gyro Hold"(TRUE ("Auto Gyro Hold")) -> ()
          n638 = global write "Robot Global Data.vi" "Auto State"(2.0 ("Auto State")) -> ()
          n639 = Wait (ms)(milliseconds to wait=u32 100) -> ()  [unwired: 1 out]
        }
        frame #4 {
          # "Close lift, wait 0.5 sec for lift to close"
          n640 = global write "Robot Global Data.vi" "Auto Joy 0 Axis X"(0.0 ("Auto Joy 0 Axis X")) -> ()
          n641 = global write "Robot Global Data.vi" "Auto Joy 0 Axis Y"(0.0 ("Auto Joy 0 Axis X")) -> ()
          n642 = global write "Robot Global Data.vi" "Auto Joy 0 Axis Z"(0.0 ("Auto Joy 0 Axis X")) -> ()
          n643 = global write "Robot Global Data.vi" "Auto Gyro Hold"(TRUE ("Auto Gyro Hold")) -> ()
          n644 = global write "Robot Global Data.vi" "Auto Close Forks"(TRUE ("Auto Gyro Hold")) -> ()
          n645 = global write "Robot Global Data.vi" "Auto State"(3.0 ("Auto State")) -> ()
          n646 = Wait (ms)(milliseconds to wait=u32 500) -> ()  [unwired: 1 out]
        }
        frame #5 {
          # "Ensure at least 0.5sec wait"
          # "Lift up crate for 2500 counts"
          n647 = global write "Robot Global Data.vi" "Auto Joy 0 Axis X"(0.0 ("Auto Joy 0 Axis X")) -> ()
          n648 = global write "Robot Global Data.vi" "Auto Joy 0 Axis Y"(0.0 ("Auto Joy 0 Axis X")) -> ()
          n649 = global write "Robot Global Data.vi" "Auto Joy 0 Axis Z"(0.0 ("Auto Joy 0 Axis X")) -> ()
          n650 = global write "Robot Global Data.vi" "Auto Gyro Hold"(TRUE ("Auto Gyro Hold")) -> ()
          n651 = global write "Robot Global Data.vi" "Auto Close Forks"(FALSE ("Auto Gyro Hold")) -> ()
          n652 = while {
            stop <- w665 stop-if-true
            n653 = global read "Robot Global Data.vi" "Lift Stopped"() -> (w665:bool)
          }
          n654 = global write "Robot Global Data.vi" "Auto Lift Encoder"(2500.0 ("Auto Joy 0 Axis X")) -> ()
          n655 = Wait (ms)(milliseconds to wait=u32 500) -> ()  [unwired: 1 out]
          n656 = global write "Robot Global Data.vi" "Auto State"(4.0 ("Auto State")) -> ()
        }
        frame #6 {
          # "Drive backward until count = 1400\n(was 1350)"
          n657 = global write "Robot Global Data.vi" "Auto Joy 0 Axis X"(0.0 ("Auto Joy 0 Axis X")) -> ()
          n658 = global write "Robot Global Data.vi" "Auto Joy 0 Axis Y"(0.33 ("Auto Joy 0 Axis X")) -> ()
          n659 = global write "Robot Global Data.vi" "Auto Joy 0 Axis Z"(0.0 ("Auto Joy 0 Axis X")) -> ()
          n660 = global write "Robot Global Data.vi" "Auto Gyro Hold"(TRUE ("Auto Gyro Hold")) -> ()
          n661 = while {
            stop <- w673 stop-if-true
            n662 = global read "Robot Global Data.vi" "Wheel Encoder Distance"() -> (w671:dbl)
            n663 = Greater Or Equal?(x=w671, y=1400.0) -> (x >= y?=w673:bool)
          }
          n664 = global write "Robot Global Data.vi" "Auto State"(5.0 ("Auto State")) -> ()
        }
        frame #7 {
          # "100 is an inch above bottom limit switch\nNote: Trash Can keeps forks from engaing bottom limit\nswitch so use encoder!!!!"
          # "-200 is a dummy to get to bottom limit switch"
          # "Stop robot, lower crate"
          n665 = global write "Robot Global Data.vi" "Auto Joy 0 Axis X"(0.0 ("Auto Joy 0 Axis X")) -> ()
          n666 = global write "Robot Global Data.vi" "Auto Joy 0 Axis Y"(0.0 ("Auto Joy 0 Axis X")) -> ()
          n667 = global write "Robot Global Data.vi" "Auto Joy 0 Axis Z"(0.0 ("Auto Joy 0 Axis X")) -> ()
          n668 = global write "Robot Global Data.vi" "Auto Gyro Hold"(TRUE ("Auto Gyro Hold")) -> ()
          n669 = while {
            stop <- w680 stop-if-true
            n670 = global read "Robot Global Data.vi" "Lift Encoder Distance"() -> (w682:dbl)
            n671 = Less Or Equal?(x=w682, y=100.0) -> (x <= y?=w680:bool)
          }
          n672 = global write "Robot Global Data.vi" "Auto Lift Encoder"(-200.0 ("Auto Joy 0 Axis X")) -> ()
          n673 = global write "Robot Global Data.vi" "Auto State"(6.0 ("Auto State")) -> ()
        }
        frame #8 {
          # "Open lift, wait 0.5 sec for lift to open"
          n674 = global write "Robot Global Data.vi" "Auto Joy 0 Axis X"(0.0 ("Auto Joy 0 Axis X")) -> ()
          n675 = global write "Robot Global Data.vi" "Auto Joy 0 Axis Y"(0.0 ("Auto Joy 0 Axis X")) -> ()
          n676 = global write "Robot Global Data.vi" "Auto Joy 0 Axis Z"(0.0 ("Auto Joy 0 Axis X")) -> ()
          n677 = global write "Robot Global Data.vi" "Auto Gyro Hold"(TRUE ("Auto Gyro Hold")) -> ()
          n678 = global write "Robot Global Data.vi" "Auto Open Forks"(TRUE ("Auto Gyro Hold")) -> ()
          n679 = global write "Robot Global Data.vi" "Auto State"(7.0 ("Auto State")) -> ()
          n680 = Wait (ms)(milliseconds to wait=u32 500) -> ()  [unwired: 1 out]
        }
        frame #9 {
          # "Drive backward until count = 1600\n(was 1700)"
          n681 = global write "Robot Global Data.vi" "Auto Joy 0 Axis X"(0.0 ("Auto Joy 0 Axis X")) -> ()
          n682 = global write "Robot Global Data.vi" "Auto Joy 0 Axis Y"(0.3 ("Auto Joy 0 Axis X")) -> ()
          n683 = global write "Robot Global Data.vi" "Auto Joy 0 Axis Z"(0.0 ("Auto Joy 0 Axis X")) -> ()
          n684 = global write "Robot Global Data.vi" "Auto Gyro Hold"(TRUE ("Auto Gyro Hold")) -> ()
          n685 = global write "Robot Global Data.vi" "Auto Open Forks"(FALSE ("Auto Gyro Hold")) -> ()
          n686 = while {
            stop <- w698 stop-if-true
            n687 = global read "Robot Global Data.vi" "Wheel Encoder Distance"() -> (w697:dbl)
            n688 = Greater Or Equal?(x=w697, y=1600.0) -> (x >= y?=w698:bool)
          }
          n689 = global write "Robot Global Data.vi" "Auto State"(8.0 ("Auto State")) -> ()
        }
        frame #10 {
          # "Stop and wait until teleop"
          n690 = global write "Robot Global Data.vi" "Auto Joy 0 Axis X"(0.0 ("Auto Joy 0 Axis X")) -> ()
          n691 = global write "Robot Global Data.vi" "Auto Joy 0 Axis Y"(0.0 ("Auto Joy 0 Axis X")) -> ()
          n692 = global write "Robot Global Data.vi" "Auto Joy 0 Axis Z"(0.0 ("Auto Joy 0 Axis X")) -> ()
          n693 = global write "Robot Global Data.vi" "Auto Gyro Hold"(FALSE ("Auto Gyro Hold")) -> ()
          n694 = global write "Robot Global Data.vi" "Auto State"(9.0 ("Auto State")) -> ()
          n695 = Wait (ms)(milliseconds to wait=u32 15000) -> ()  [unwired: 1 out]
        }
      }
    }
  }
  n696 = case shown="True" w25 {
    frame False {
    }
    frame True {
      n697 = stacked-sequence {
        frame #0 {
          # "Reset encoders"
          # "Reset Gyro"
          # "Initialize"
          n698 = global write "Robot Global Data.vi" "Auto Joy 1 Axis Y"(0.0 ("Auto Joy 0 Axis X")) -> ()
          n699 = global write "Robot Global Data.vi" "Auto Joy 0 Axis X"(0.0 ("Auto Joy 0 Axis X")) -> ()
          n700 = global write "Robot Global Data.vi" "Auto Joy 0 Axis Y"(0.0 ("Auto Joy 0 Axis X")) -> ()
          n701 = global write "Robot Global Data.vi" "Auto Joy 0 Axis Z"(0.0 ("Auto Joy 0 Axis X")) -> ()
          n702 = global write "Robot Global Data.vi" "Gyro Reset"(TRUE ("Auto Gyro Hold")) -> ()
          n703 = global write "Robot Global Data.vi" "Lift Encoder Reset"(TRUE ("Auto Gyro Hold")) -> ()
          n704 = global write "Robot Global Data.vi" "Wheel Encoder Reset"(TRUE ("Wheel Encoder Reset")) -> ()
          n705 = global write "Robot Global Data.vi" "Auto Gyro Hold"(FALSE ("Auto Gyro Hold")) -> ()
          n706 = global write "Robot Global Data.vi" "Auto Open Forks"(FALSE ("Auto Gyro Hold")) -> ()
          n707 = global write "Robot Global Data.vi" "Auto Close Forks"(FALSE ("Auto Gyro Hold")) -> ()
          n708 = global write "Robot Global Data.vi" "PID Target Angle"(0.0 ("Auto Joy 0 Axis Z")) -> ()
          n709 = global write "Robot Global Data.vi" "Raw Gyro Angle"(0.0 ("Auto Joy 0 Axis Z")) -> ()
          n710 = global write "Robot Global Data.vi" "Auto State"(0.0 ("Auto State")) -> ()
          n711 = Wait (ms)(milliseconds to wait=u32 50) -> ()  [unwired: 1 out]
        }
        frame #1 {
          # "Reset encoders"
          # "Reset Gyro"
          # "Initialize"
          n712 = global write "Robot Global Data.vi" "Auto Joy 0 Axis X"(0.0 ("Auto Joy 0 Axis X")) -> ()
          n713 = global write "Robot Global Data.vi" "Auto Joy 0 Axis Y"(0.0 ("Auto Joy 0 Axis X")) -> ()
          n714 = global write "Robot Global Data.vi" "Auto Joy 0 Axis Z"(0.0 ("Auto Joy 0 Axis X")) -> ()
          n715 = global write "Robot Global Data.vi" "Gyro Reset"(FALSE ("Auto Gyro Hold")) -> ()
          n716 = global write "Robot Global Data.vi" "Lift Encoder Reset"(FALSE ("Auto Gyro Hold")) -> ()
          n717 = global write "Robot Global Data.vi" "Wheel Encoder Reset"(FALSE ("Wheel Encoder Reset")) -> ()
          n718 = global write "Robot Global Data.vi" "Auto State"(0.0 ("Auto State")) -> ()
          n719 = Wait (ms)(milliseconds to wait=u32 50) -> ()  [unwired: 1 out]
        }
        frame #2 {
          # "Lock Gyro"
          # "Drive forward for 50 counts"
          n720 = global write "Robot Global Data.vi" "Auto Joy 0 Axis X"(0.0 ("Auto Joy 0 Axis X")) -> ()
          n721 = global write "Robot Global Data.vi" "Auto Joy 0 Axis Y"(-0.25 ("Auto Joy 0 Axis X")) -> ()
          n722 = global write "Robot Global Data.vi" "Auto Joy 0 Axis Z"(0.0 ("Auto Joy 0 Axis X")) -> ()
          n723 = global write "Robot Global Data.vi" "Auto Gyro Hold"(TRUE ("Auto Gyro Hold")) -> ()
          n724 = global write "Robot Global Data.vi" "Lift Encoder Reset"(FALSE ("Auto Gyro Hold")) -> ()
          n725 = global write "Robot Global Data.vi" "Wheel Encoder Reset"(FALSE ("Wheel Encoder Reset")) -> ()
          n726 = while {
            stop <- w734 stop-if-true
            n727 = global read "Robot Global Data.vi" "Wheel Encoder Distance"() -> (w736:dbl)
            n728 = Less Or Equal?(x=w736, y=-50.0) -> (x <= y?=w734:bool)
          }
          n729 = global write "Robot Global Data.vi" "Auto State"(1.0 ("Auto State")) -> ()
        }
        frame #3 {
          # "Stop robot and wait 0.1 sec"
          n730 = global write "Robot Global Data.vi" "Auto Joy 0 Axis X"(0.0 ("Auto Joy 0 Axis X")) -> ()
          n731 = global write "Robot Global Data.vi" "Auto Joy 0 Axis Y"(0.0 ("Auto Joy 0 Axis X")) -> ()
          n732 = global write "Robot Global Data.vi" "Auto Joy 0 Axis Z"(0.0 ("Auto Joy 0 Axis X")) -> ()
          n733 = global write "Robot Global Data.vi" "Auto Gyro Hold"(TRUE ("Auto Gyro Hold")) -> ()
          n734 = global write "Robot Global Data.vi" "Auto State"(2.0 ("Auto State")) -> ()
          n735 = Wait (ms)(milliseconds to wait=u32 100) -> ()  [unwired: 1 out]
        }
        frame #4 {
          # "Close lift, wait 0.5 sec for lift to close"
          n736 = global write "Robot Global Data.vi" "Auto Joy 0 Axis X"(0.0 ("Auto Joy 0 Axis X")) -> ()
          n737 = global write "Robot Global Data.vi" "Auto Joy 0 Axis Y"(0.0 ("Auto Joy 0 Axis X")) -> ()
          n738 = global write "Robot Global Data.vi" "Auto Joy 0 Axis Z"(0.0 ("Auto Joy 0 Axis X")) -> ()
          n739 = global write "Robot Global Data.vi" "Auto Gyro Hold"(TRUE ("Auto Gyro Hold")) -> ()
          n740 = global write "Robot Global Data.vi" "Auto Close Forks"(TRUE ("Auto Gyro Hold")) -> ()
          n741 = global write "Robot Global Data.vi" "Auto State"(3.0 ("Auto State")) -> ()
          n742 = Wait (ms)(milliseconds to wait=u32 500) -> ()  [unwired: 1 out]
        }
        frame #5 {
          # "Ensure at least 0.5sec wait"
          # "Lift up crate for 2500 counts"
          n743 = global write "Robot Global Data.vi" "Auto Joy 0 Axis X"(0.0 ("Auto Joy 0 Axis X")) -> ()
          n744 = global write "Robot Global Data.vi" "Auto Joy 0 Axis Y"(0.0 ("Auto Joy 0 Axis X")) -> ()
          n745 = global write "Robot Global Data.vi" "Auto Joy 0 Axis Z"(0.0 ("Auto Joy 0 Axis X")) -> ()
          n746 = global write "Robot Global Data.vi" "Auto Gyro Hold"(TRUE ("Auto Gyro Hold")) -> ()
          n747 = global write "Robot Global Data.vi" "Auto Close Forks"(FALSE ("Auto Gyro Hold")) -> ()
          n748 = while {
            stop <- w758 stop-if-true
            n749 = global read "Robot Global Data.vi" "Lift Stopped"() -> (w758:bool)
          }
          n750 = global write "Robot Global Data.vi" "Auto Lift Encoder"(2500.0 ("Auto Joy 0 Axis X")) -> ()
          n751 = Wait (ms)(milliseconds to wait=u32 500) -> ()  [unwired: 1 out]
          n752 = global write "Robot Global Data.vi" "Auto State"(4.0 ("Auto State")) -> ()
        }
        frame #6 {
          # "Wait for robot to finish turning"
          # "Turn robot 90 degrees clockwise"
          n753 = global write "Robot Global Data.vi" "Auto Joy 0 Axis X"(0.0 ("Auto Joy 0 Axis X")) -> ()
          n754 = global write "Robot Global Data.vi" "Auto Joy 0 Axis Y"(0.0 ("Auto Joy 0 Axis X")) -> ()
          n755 = global write "Robot Global Data.vi" "Auto Joy 0 Axis Z"(0.0 ("Auto Joy 0 Axis X")) -> ()
          n756 = global write "Robot Global Data.vi" "Auto Gyro Hold"(TRUE ("Auto Gyro Hold")) -> ()
          n757 = global write "Robot Global Data.vi" "PID Target Angle"(90.0 ("Auto Joy 0 Axis Z")) -> ()
          n758 = global write "Robot Global Data.vi" "Auto State"(5.0 ("Auto State")) -> ()
          n759 = Wait (ms)(milliseconds to wait=u32 2000) -> ()  [unwired: 1 out]
        }
        frame #7 {
          # "Reset wheel counter since robot turned,\nhence forward count is incorrect."
          n760 = global write "Robot Global Data.vi" "Auto Joy 0 Axis X"(0.0 ("Auto Joy 0 Axis X")) -> ()
          n761 = global write "Robot Global Data.vi" "Auto Joy 0 Axis Y"(0.0 ("Auto Joy 0 Axis X")) -> ()
          n762 = global write "Robot Global Data.vi" "Auto Joy 0 Axis Z"(0.0 ("Auto Joy 0 Axis X")) -> ()
          n763 = global write "Robot Global Data.vi" "Auto Gyro Hold"(TRUE ("Auto Gyro Hold")) -> ()
          n764 = global write "Robot Global Data.vi" "Wheel Encoder Reset"(TRUE ("Wheel Encoder Reset")) -> ()
          n765 = global write "Robot Global Data.vi" "Auto State"(6.0 ("Auto State")) -> ()
          n766 = Wait (ms)(milliseconds to wait=u32 50) -> ()  [unwired: 1 out]
        }
        frame #8 {
          # "Enable wheel counter."
          n767 = global write "Robot Global Data.vi" "Auto Joy 0 Axis X"(0.0 ("Auto Joy 0 Axis X")) -> ()
          n768 = global write "Robot Global Data.vi" "Auto Joy 0 Axis Y"(0.0 ("Auto Joy 0 Axis X")) -> ()
          n769 = global write "Robot Global Data.vi" "Auto Joy 0 Axis Z"(0.0 ("Auto Joy 0 Axis X")) -> ()
          n770 = global write "Robot Global Data.vi" "Auto Gyro Hold"(TRUE ("Auto Gyro Hold")) -> ()
          n771 = global write "Robot Global Data.vi" "Wheel Encoder Reset"(FALSE ("Wheel Encoder Reset")) -> ()
          n772 = global write "Robot Global Data.vi" "Auto State"(7.0 ("Auto State")) -> ()
          n773 = Wait (ms)(milliseconds to wait=u32 50) -> ()  [unwired: 1 out]
        }
        frame #9 {
          # "Drive forward until count = -1850"
          n774 = global write "Robot Global Data.vi" "Auto Joy 0 Axis X"(0.0 ("Auto Joy 0 Axis X")) -> ()
          n775 = global write "Robot Global Data.vi" "Auto Joy 0 Axis Y"(-0.33 ("Auto Joy 0 Axis X")) -> ()
          n776 = global write "Robot Global Data.vi" "Auto Joy 0 Axis Z"(0.0 ("Auto Joy 0 Axis X")) -> ()
          n777 = global write "Robot Global Data.vi" "Auto Gyro Hold"(TRUE ("Auto Gyro Hold")) -> ()
          n778 = global write "Robot Global Data.vi" "Wheel Encoder Reset"(FALSE ("Wheel Encoder Reset")) -> ()
          n779 = while {
            stop <- w788 stop-if-true
            n780 = global read "Robot Global Data.vi" "Wheel Encoder Distance"() -> (w787:dbl)
            n781 = Less Or Equal?(x=w787, y=-1850.0) -> (x <= y?=w788:bool)
          }
          n782 = global write "Robot Global Data.vi" "Auto State"(8.0 ("Auto State")) -> ()
        }
        frame #10 {
          # "100 is an inch above bottom limit switch\nNote: Trash Can keeps forks from engaing bottom limit\nswitch so use encoder!!!!"
          # "-200 is a dummy to get to bottom limit switch"
          # "Stop robot, lower crate"
          n783 = global write "Robot Global Data.vi" "Auto Joy 0 Axis X"(0.0 ("Auto Joy 0 Axis X")) -> ()
          n784 = global write "Robot Global Data.vi" "Auto Joy 0 Axis Y"(0.0 ("Auto Joy 0 Axis X")) -> ()
          n785 = global write "Robot Global Data.vi" "Auto Joy 0 Axis Z"(0.0 ("Auto Joy 0 Axis X")) -> ()
          n786 = global write "Robot Global Data.vi" "Auto Gyro Hold"(TRUE ("Auto Gyro Hold")) -> ()
          n787 = while {
            stop <- w795 stop-if-true
            n788 = global read "Robot Global Data.vi" "Lift Encoder Distance"() -> (w797:dbl)
            n789 = Less Or Equal?(x=w797, y=100.0) -> (x <= y?=w795:bool)
          }
          n790 = global write "Robot Global Data.vi" "Auto Lift Encoder"(-200.0 ("Auto Joy 0 Axis X")) -> ()
          n791 = global write "Robot Global Data.vi" "Auto State"(9.0 ("Auto State")) -> ()
        }
        frame #11 {
          # "Open lift, wait 0.5 sec for lift to open"
          n792 = global write "Robot Global Data.vi" "Auto Joy 0 Axis X"(0.0 ("Auto Joy 0 Axis X")) -> ()
          n793 = global write "Robot Global Data.vi" "Auto Joy 0 Axis Y"(0.0 ("Auto Joy 0 Axis X")) -> ()
          n794 = global write "Robot Global Data.vi" "Auto Joy 0 Axis Z"(0.0 ("Auto Joy 0 Axis X")) -> ()
          n795 = global write "Robot Global Data.vi" "Auto Gyro Hold"(TRUE ("Auto Gyro Hold")) -> ()
          n796 = global write "Robot Global Data.vi" "Auto Open Forks"(TRUE ("Auto Gyro Hold")) -> ()
          n797 = global write "Robot Global Data.vi" "Auto State"(10.0 ("Auto State")) -> ()
          n798 = Wait (ms)(milliseconds to wait=u32 500) -> ()  [unwired: 1 out]
        }
        frame #12 {
          # "Drive backward until count = -1950"
          n799 = global write "Robot Global Data.vi" "Auto Joy 0 Axis X"(0.0 ("Auto Joy 0 Axis X")) -> ()
          n800 = global write "Robot Global Data.vi" "Auto Joy 0 Axis Y"(0.25 ("Auto Joy 0 Axis X")) -> ()
          n801 = global write "Robot Global Data.vi" "Auto Joy 0 Axis Z"(0.0 ("Auto Joy 0 Axis X")) -> ()
          n802 = global write "Robot Global Data.vi" "Auto Gyro Hold"(TRUE ("Auto Gyro Hold")) -> ()
          n803 = global write "Robot Global Data.vi" "Auto Open Forks"(FALSE ("Auto Gyro Hold")) -> ()
          n804 = while {
            stop <- w813 stop-if-true
            n805 = global read "Robot Global Data.vi" "Wheel Encoder Distance"() -> (w812:dbl)
            n806 = Greater Or Equal?(x=w812, y=-1950.0) -> (x >= y?=w813:bool)
          }
          n807 = global write "Robot Global Data.vi" "Auto State"(11.0 ("Auto State")) -> ()
        }
        frame #13 {
          # "Stop and wait until teleop"
          n808 = global write "Robot Global Data.vi" "Auto Joy 0 Axis X"(0.0 ("Auto Joy 0 Axis X")) -> ()
          n809 = global write "Robot Global Data.vi" "Auto Joy 0 Axis Y"(0.0 ("Auto Joy 0 Axis X")) -> ()
          n810 = global write "Robot Global Data.vi" "Auto Joy 0 Axis Z"(0.0 ("Auto Joy 0 Axis X")) -> ()
          n811 = global write "Robot Global Data.vi" "Auto Gyro Hold"(FALSE ("Auto Gyro Hold")) -> ()
          n812 = global write "Robot Global Data.vi" "Auto State"(12.0 ("Auto State")) -> ()
          n813 = Wait (ms)(milliseconds to wait=u32 15000) -> ()  [unwired: 1 out]
        }
      }
    }
  }
  n814 = case shown="True" w23 {
    frame False {
    }
    frame True {
      n815 = stacked-sequence {
        frame #0 {
          # "Reset encoders"
          # "Reset Gyro"
          # "Initialize"
          n816 = global write "Robot Global Data.vi" "Auto Joy 1 Axis Y"(0.0 ("Auto Joy 0 Axis X")) -> ()
          n817 = global write "Robot Global Data.vi" "Auto Joy 0 Axis X"(0.0 ("Auto Joy 0 Axis X")) -> ()
          n818 = global write "Robot Global Data.vi" "Auto Joy 0 Axis Y"(0.0 ("Auto Joy 0 Axis X")) -> ()
          n819 = global write "Robot Global Data.vi" "Auto Joy 0 Axis Z"(0.0 ("Auto Joy 0 Axis X")) -> ()
          n820 = global write "Robot Global Data.vi" "Auto Open Forks"(FALSE ("Auto Gyro Hold")) -> ()
          n821 = global write "Robot Global Data.vi" "Gyro Reset"(TRUE ("Auto Gyro Hold")) -> ()
          n822 = global write "Robot Global Data.vi" "Auto Close Forks"(FALSE ("Auto Gyro Hold")) -> ()
          n823 = global write "Robot Global Data.vi" "Lift Encoder Reset"(TRUE ("Auto Gyro Hold")) -> ()
          n824 = global write "Robot Global Data.vi" "Wheel Encoder Reset"(TRUE ("Wheel Encoder Reset")) -> ()
          n825 = global write "Robot Global Data.vi" "Auto Gyro Hold"(FALSE ("Auto Gyro Hold")) -> ()
          n826 = global write "Robot Global Data.vi" "PID Target Angle"(0.0 ("Auto Joy 0 Axis Z")) -> ()
          n827 = global write "Robot Global Data.vi" "Raw Gyro Angle"(0.0 ("Auto Joy 0 Axis Z")) -> ()
          n828 = global write "Robot Global Data.vi" "Auto State"(0.0 ("Auto State")) -> ()
          n829 = Wait (ms)(milliseconds to wait=u32 50) -> ()  [unwired: 1 out]
        }
        frame #1 {
          # "Reset encoders"
          # "Reset Gyro"
          # "Initialize"
          n830 = global write "Robot Global Data.vi" "Auto Joy 0 Axis X"(0.0 ("Auto Joy 0 Axis X")) -> ()
          n831 = global write "Robot Global Data.vi" "Auto Joy 0 Axis Y"(0.0 ("Auto Joy 0 Axis X")) -> ()
          n832 = global write "Robot Global Data.vi" "Auto Joy 0 Axis Z"(0.0 ("Auto Joy 0 Axis X")) -> ()
          n833 = global write "Robot Global Data.vi" "Gyro Reset"(FALSE ("Auto Gyro Hold")) -> ()
          n834 = global write "Robot Global Data.vi" "Lift Encoder Reset"(FALSE ("Auto Gyro Hold")) -> ()
          n835 = global write "Robot Global Data.vi" "Wheel Encoder Reset"(FALSE ("Wheel Encoder Reset")) -> ()
          n836 = global write "Robot Global Data.vi" "Auto State"(0.0 ("Auto State")) -> ()
          n837 = Wait (ms)(milliseconds to wait=u32 50) -> ()  [unwired: 1 out]
        }
        frame #2 {
          # "Drive forward for 50 counts"
          n838 = global write "Robot Global Data.vi" "Auto Joy 0 Axis X"(0.0 ("Auto Joy 0 Axis X")) -> ()
          n839 = global write "Robot Global Data.vi" "Auto Joy 0 Axis Y"(-0.25 ("Auto Joy 0 Axis X")) -> ()
          n840 = global write "Robot Global Data.vi" "Auto Joy 0 Axis Z"(0.0 ("Auto Joy 0 Axis X")) -> ()
          n841 = global write "Robot Global Data.vi" "Auto Gyro Hold"(TRUE ("Auto Gyro Hold")) -> ()
          n842 = global write "Robot Global Data.vi" "Lift Encoder Reset"(FALSE ("Auto Gyro Hold")) -> ()
          n843 = global write "Robot Global Data.vi" "Wheel Encoder Reset"(FALSE ("Wheel Encoder Reset")) -> ()
          n844 = while {
            stop <- w849 stop-if-true
            n845 = global read "Robot Global Data.vi" "Wheel Encoder Distance"() -> (w851:dbl)
            n846 = Less Or Equal?(x=w851, y=-50.0) -> (x <= y?=w849:bool)
          }
          n847 = global write "Robot Global Data.vi" "Auto State"(1.0 ("Auto State")) -> ()
        }
        frame #3 {
          # "Stop robot and wait 0.1 sec"
          n848 = global write "Robot Global Data.vi" "Auto Joy 0 Axis X"(0.0 ("Auto Joy 0 Axis X")) -> ()
          n849 = global write "Robot Global Data.vi" "Auto Joy 0 Axis Y"(0.0 ("Auto Joy 0 Axis X")) -> ()
          n850 = global write "Robot Global Data.vi" "Auto Joy 0 Axis Z"(0.0 ("Auto Joy 0 Axis X")) -> ()
          n851 = global write "Robot Global Data.vi" "Auto Gyro Hold"(TRUE ("Auto Gyro Hold")) -> ()
          n852 = global write "Robot Global Data.vi" "Auto State"(2.0 ("Auto State")) -> ()
          n853 = Wait (ms)(milliseconds to wait=u32 100) -> ()  [unwired: 1 out]
        }
        frame #4 {
          # "Close lift, wait 0.5 sec for lift to close"
          n854 = global write "Robot Global Data.vi" "Auto Joy 0 Axis X"(0.0 ("Auto Joy 0 Axis X")) -> ()
          n855 = global write "Robot Global Data.vi" "Auto Joy 0 Axis Y"(0.0 ("Auto Joy 0 Axis X")) -> ()
          n856 = global write "Robot Global Data.vi" "Auto Joy 0 Axis Z"(0.0 ("Auto Joy 0 Axis X")) -> ()
          n857 = global write "Robot Global Data.vi" "Auto Gyro Hold"(TRUE ("Auto Gyro Hold")) -> ()
          n858 = global write "Robot Global Data.vi" "Auto Close Forks"(TRUE ("Auto Gyro Hold")) -> ()
          n859 = global write "Robot Global Data.vi" "Auto State"(3.0 ("Auto State")) -> ()
          n860 = Wait (ms)(milliseconds to wait=u32 500) -> ()  [unwired: 1 out]
        }
        frame #5 {
          # "Ensure at least 0.5sec wait"
          # "Lift up crate for 2500 counts"
          n861 = global write "Robot Global Data.vi" "Auto Joy 0 Axis X"(0.0 ("Auto Joy 0 Axis X")) -> ()
          n862 = global write "Robot Global Data.vi" "Auto Joy 0 Axis Y"(0.0 ("Auto Joy 0 Axis X")) -> ()
          n863 = global write "Robot Global Data.vi" "Auto Joy 0 Axis Z"(0.0 ("Auto Joy 0 Axis X")) -> ()
          n864 = global write "Robot Global Data.vi" "Auto Gyro Hold"(TRUE ("Auto Gyro Hold")) -> ()
          n865 = global write "Robot Global Data.vi" "Auto Close Forks"(FALSE ("Auto Gyro Hold")) -> ()
          n866 = while {
            stop <- w873 stop-if-true
            n867 = global read "Robot Global Data.vi" "Lift Stopped"() -> (w873:bool)
          }
          n868 = global write "Robot Global Data.vi" "Auto Lift Encoder"(2500.0 ("Auto Joy 0 Axis X")) -> ()
          n869 = Wait (ms)(milliseconds to wait=u32 500) -> ()  [unwired: 1 out]
          n870 = global write "Robot Global Data.vi" "Auto State"(4.0 ("Auto State")) -> ()
        }
        frame #6 {
          # "Wait for robot to finish turning"
          # "Turn robot 90 degrees clockwise"
          n871 = global write "Robot Global Data.vi" "Auto Joy 0 Axis X"(0.0 ("Auto Joy 0 Axis X")) -> ()
          n872 = global write "Robot Global Data.vi" "Auto Joy 0 Axis Y"(0.0 ("Auto Joy 0 Axis X")) -> ()
          n873 = global write "Robot Global Data.vi" "Auto Joy 0 Axis Z"(0.0 ("Auto Joy 0 Axis X")) -> ()
          n874 = global write "Robot Global Data.vi" "Auto Gyro Hold"(TRUE ("Auto Gyro Hold")) -> ()
          n875 = global write "Robot Global Data.vi" "PID Target Angle"(-90.0 ("Auto Joy 0 Axis Z")) -> ()
          n876 = global write "Robot Global Data.vi" "Auto State"(5.0 ("Auto State")) -> ()
          n877 = Wait (ms)(milliseconds to wait=u32 2000) -> ()  [unwired: 1 out]
        }
        frame #7 {
          # "Reset wheel counter since robot turned,\nhence forward count is incorrect."
          n878 = global write "Robot Global Data.vi" "Auto Joy 0 Axis X"(0.0 ("Auto Joy 0 Axis X")) -> ()
          n879 = global write "Robot Global Data.vi" "Auto Joy 0 Axis Y"(0.0 ("Auto Joy 0 Axis X")) -> ()
          n880 = global write "Robot Global Data.vi" "Auto Joy 0 Axis Z"(0.0 ("Auto Joy 0 Axis X")) -> ()
          n881 = global write "Robot Global Data.vi" "Auto Gyro Hold"(TRUE ("Auto Gyro Hold")) -> ()
          n882 = global write "Robot Global Data.vi" "Wheel Encoder Reset"(TRUE ("Wheel Encoder Reset")) -> ()
          n883 = global write "Robot Global Data.vi" "Auto State"(6.0 ("Auto State")) -> ()
          n884 = Wait (ms)(milliseconds to wait=u32 50) -> ()  [unwired: 1 out]
        }
        frame #8 {
          # "Enable wheel counter."
          n885 = global write "Robot Global Data.vi" "Auto Joy 0 Axis X"(0.0 ("Auto Joy 0 Axis X")) -> ()
          n886 = global write "Robot Global Data.vi" "Auto Joy 0 Axis Y"(0.0 ("Auto Joy 0 Axis X")) -> ()
          n887 = global write "Robot Global Data.vi" "Auto Joy 0 Axis Z"(0.0 ("Auto Joy 0 Axis X")) -> ()
          n888 = global write "Robot Global Data.vi" "Auto Gyro Hold"(TRUE ("Auto Gyro Hold")) -> ()
          n889 = global write "Robot Global Data.vi" "Wheel Encoder Reset"(FALSE ("Wheel Encoder Reset")) -> ()
          n890 = global write "Robot Global Data.vi" "Auto State"(7.0 ("Auto State")) -> ()
          n891 = Wait (ms)(milliseconds to wait=u32 50) -> ()  [unwired: 1 out]
        }
        frame #9 {
          # "Drive forward until count = -1850"
          n892 = global write "Robot Global Data.vi" "Auto Joy 0 Axis X"(0.0 ("Auto Joy 0 Axis X")) -> ()
          n893 = global write "Robot Global Data.vi" "Auto Joy 0 Axis Y"(-0.33 ("Auto Joy 0 Axis X")) -> ()
          n894 = global write "Robot Global Data.vi" "Auto Joy 0 Axis Z"(0.0 ("Auto Joy 0 Axis X")) -> ()
          n895 = global write "Robot Global Data.vi" "Auto Gyro Hold"(TRUE ("Auto Gyro Hold")) -> ()
          n896 = global write "Robot Global Data.vi" "Wheel Encoder Reset"(FALSE ("Wheel Encoder Reset")) -> ()
          n897 = while {
            stop <- w903 stop-if-true
            n898 = global read "Robot Global Data.vi" "Wheel Encoder Distance"() -> (w902:dbl)
            n899 = Less Or Equal?(x=w902, y=-1850.0) -> (x <= y?=w903:bool)
          }
          n900 = global write "Robot Global Data.vi" "Auto State"(8.0 ("Auto State")) -> ()
        }
        frame #10 {
          # "100 is an inch above bottom limit switch\nNote: Trash Can keeps forks from engaing bottom limit\nswitch so use encoder!!!!"
          # "Stop robot, lower crate"
          n901 = global write "Robot Global Data.vi" "Auto Joy 0 Axis X"(0.0 ("Auto Joy 0 Axis X")) -> ()
          n902 = global write "Robot Global Data.vi" "Auto Joy 0 Axis Y"(0.0 ("Auto Joy 0 Axis X")) -> ()
          n903 = global write "Robot Global Data.vi" "Auto Joy 0 Axis Z"(0.0 ("Auto Joy 0 Axis X")) -> ()
          n904 = global write "Robot Global Data.vi" "Auto Gyro Hold"(TRUE ("Auto Gyro Hold")) -> ()
          n905 = while {
            stop <- w910 stop-if-true
            n906 = global read "Robot Global Data.vi" "Lift Encoder Distance"() -> (w912:dbl)
            n907 = Less Or Equal?(x=w912, y=100.0) -> (x <= y?=w910:bool)
          }
          n908 = global write "Robot Global Data.vi" "Auto Lift Encoder"(-200.0 ("Auto Joy 0 Axis X")) -> ()
          n909 = global write "Robot Global Data.vi" "Auto State"(9.0 ("Auto State")) -> ()
        }
        frame #11 {
          # "Open lift, wait 0.5 sec for lift to open"
          n910 = global write "Robot Global Data.vi" "Auto Joy 0 Axis X"(0.0 ("Auto Joy 0 Axis X")) -> ()
          n911 = global write "Robot Global Data.vi" "Auto Joy 0 Axis Y"(0.0 ("Auto Joy 0 Axis X")) -> ()
          n912 = global write "Robot Global Data.vi" "Auto Joy 0 Axis Z"(0.0 ("Auto Joy 0 Axis X")) -> ()
          n913 = global write "Robot Global Data.vi" "Auto Gyro Hold"(TRUE ("Auto Gyro Hold")) -> ()
          n914 = global write "Robot Global Data.vi" "Auto Open Forks"(TRUE ("Auto Gyro Hold")) -> ()
          n915 = global write "Robot Global Data.vi" "Auto State"(10.0 ("Auto State")) -> ()
          n916 = Wait (ms)(milliseconds to wait=u32 500) -> ()  [unwired: 1 out]
        }
        frame #12 {
          # "Drive backward until count = -1950"
          n917 = global write "Robot Global Data.vi" "Auto Joy 0 Axis X"(0.0 ("Auto Joy 0 Axis X")) -> ()
          n918 = global write "Robot Global Data.vi" "Auto Joy 0 Axis Y"(0.25 ("Auto Joy 0 Axis X")) -> ()
          n919 = global write "Robot Global Data.vi" "Auto Joy 0 Axis Z"(0.0 ("Auto Joy 0 Axis X")) -> ()
          n920 = global write "Robot Global Data.vi" "Auto Gyro Hold"(TRUE ("Auto Gyro Hold")) -> ()
          n921 = global write "Robot Global Data.vi" "Auto Open Forks"(FALSE ("Auto Gyro Hold")) -> ()
          n922 = while {
            stop <- w928 stop-if-true
            n923 = global read "Robot Global Data.vi" "Wheel Encoder Distance"() -> (w927:dbl)
            n924 = Greater Or Equal?(x=w927, y=-1950.0) -> (x >= y?=w928:bool)
          }
          n925 = global write "Robot Global Data.vi" "Auto State"(11.0 ("Auto State")) -> ()
        }
        frame #13 {
          # "Stop and wait until teleop"
          n926 = global write "Robot Global Data.vi" "Auto Joy 0 Axis X"(0.0 ("Auto Joy 0 Axis X")) -> ()
          n927 = global write "Robot Global Data.vi" "Auto Joy 0 Axis Y"(0.0 ("Auto Joy 0 Axis X")) -> ()
          n928 = global write "Robot Global Data.vi" "Auto Joy 0 Axis Z"(0.0 ("Auto Joy 0 Axis X")) -> ()
          n929 = global write "Robot Global Data.vi" "Auto Gyro Hold"(FALSE ("Auto Gyro Hold")) -> ()
          n930 = global write "Robot Global Data.vi" "Auto State"(12.0 ("Auto State")) -> ()
          n931 = Wait (ms)(milliseconds to wait=u32 15000) -> ()  [unwired: 1 out]
        }
      }
    }
  }
  n932 = case shown="True" w20 {
    frame False {
    }
    frame True {
      n933 = stacked-sequence {
        frame #0 {
          # "Pre-set Lift Encoder to +3500 before starting!!!!!!!!!!!"
          # "Reset encoders"
          # "Reset Gyro"
          # "Initialize"
          n934 = global write "Robot Global Data.vi" "Auto Joy 1 Axis Y"(0.0 ("Auto Joy 0 Axis X")) -> ()
          n935 = global write "Robot Global Data.vi" "Auto Joy 0 Axis X"(0.0 ("Auto Joy 0 Axis X")) -> ()
          n936 = global write "Robot Global Data.vi" "Auto Joy 0 Axis Y"(0.0 ("Auto Joy 0 Axis X")) -> ()
          n937 = global write "Robot Global Data.vi" "Auto Joy 0 Axis Z"(0.0 ("Auto Joy 0 Axis X")) -> ()
          n938 = global write "Robot Global Data.vi" "Gyro Reset"(TRUE ("Auto Gyro Hold")) -> ()
          n939 = global write "Robot Global Data.vi" "Wheel Encoder Reset"(TRUE ("Wheel Encoder Reset")) -> ()
          n940 = global write "Robot Global Data.vi" "Auto Gyro Hold"(FALSE ("Auto Gyro Hold")) -> ()
          n941 = global write "Robot Global Data.vi" "Auto Open Forks"(FALSE ("Auto Gyro Hold")) -> ()
          n942 = global write "Robot Global Data.vi" "Auto Close Forks"(FALSE ("Auto Gyro Hold")) -> ()
          n943 = global write "Robot Global Data.vi" "Lift Encoder Reset"(TRUE ("Auto Gyro Hold")) -> ()
          n944 = global write "Robot Global Data.vi" "Auto Lift Encoder"(0.0 ("Auto Joy 0 Axis X")) -> ()
          n945 = global write "Robot Global Data.vi" "PID Target Angle"(0.0 ("Auto Joy 0 Axis Z")) -> ()
          n946 = global write "Robot Global Data.vi" "Raw Gyro Angle"(0.0 ("Auto Joy 0 Axis Z")) -> ()
          n947 = global write "Robot Global Data.vi" "Auto State"(0.0 ("Auto State")) -> ()
          n948 = Wait (ms)(milliseconds to wait=u32 100) -> ()  [unwired: 1 out]
        }
        frame #1 {
          # "Reset encoders"
          # "Reset Gyro"
          # "Initialize"
          n949 = global write "Robot Global Data.vi" "Auto Joy 0 Axis X"(0.0 ("Auto Joy 0 Axis X")) -> ()
          n950 = global write "Robot Global Data.vi" "Auto Joy 0 Axis Y"(0.0 ("Auto Joy 0 Axis X")) -> ()
          n951 = global write "Robot Global Data.vi" "Auto Joy 0 Axis Z"(0.0 ("Auto Joy 0 Axis X")) -> ()
          n952 = global write "Robot Global Data.vi" "Gyro Reset"(FALSE ("Auto Gyro Hold")) -> ()
          n953 = global write "Robot Global Data.vi" "Lift Encoder Reset"(FALSE ("Auto Gyro Hold")) -> ()
          n954 = global write "Robot Global Data.vi" "Wheel Encoder Reset"(FALSE ("Wheel Encoder Reset")) -> ()
          n955 = global write "Robot Global Data.vi" "Auto State"(0.0 ("Auto State")) -> ()
          n956 = Wait (ms)(milliseconds to wait=u32 50) -> ()  [unwired: 1 out]
        }
        frame #2 {
          # "Drive forward for 10 counts"
          n957 = global write "Robot Global Data.vi" "Auto Joy 0 Axis X"(0.0 ("Auto Joy 0 Axis X")) -> ()
          n958 = global write "Robot Global Data.vi" "Auto Joy 0 Axis Y"(-0.25 ("Auto Joy 0 Axis X")) -> ()
          n959 = global write "Robot Global Data.vi" "Auto Joy 0 Axis Z"(0.0 ("Auto Joy 0 Axis X")) -> ()
          n960 = global write "Robot Global Data.vi" "Auto Gyro Hold"(TRUE ("Auto Gyro Hold")) -> ()
          n961 = global write "Robot Global Data.vi" "Lift Encoder Reset"(FALSE ("Auto Gyro Hold")) -> ()
          n962 = global write "Robot Global Data.vi" "Wheel Encoder Reset"(FALSE ("Wheel Encoder Reset")) -> ()
          n963 = while {
            stop <- w965 stop-if-true
            n964 = global read "Robot Global Data.vi" "Wheel Encoder Distance"() -> (w967:dbl)
            n965 = Less Or Equal?(x=w967, y=-10.0) -> (x <= y?=w965:bool)
          }
          n966 = global write "Robot Global Data.vi" "Auto State"(1.0 ("Auto State")) -> ()
        }
        frame #3 {
          # "Stop robot and wait 0.1 sec"
          n967 = global write "Robot Global Data.vi" "Auto Joy 0 Axis X"(0.0 ("Auto Joy 0 Axis X")) -> ()
          n968 = global write "Robot Global Data.vi" "Auto Joy 0 Axis Y"(0.0 ("Auto Joy 0 Axis X")) -> ()
          n969 = global write "Robot Global Data.vi" "Auto Joy 0 Axis Z"(0.0 ("Auto Joy 0 Axis X")) -> ()
          n970 = global write "Robot Global Data.vi" "Auto Gyro Hold"(TRUE ("Auto Gyro Hold")) -> ()
          n971 = global write "Robot Global Data.vi" "Auto State"(2.0 ("Auto State")) -> ()
          n972 = Wait (ms)(milliseconds to wait=u32 100) -> ()  [unwired: 1 out]
        }
        frame #4 {
          # "Close lift, wait 0.5 sec for lift to close"
          n973 = global write "Robot Global Data.vi" "Auto Joy 0 Axis X"(0.0 ("Auto Joy 0 Axis X")) -> ()
          n974 = global write "Robot Global Data.vi" "Auto Joy 0 Axis Y"(0.0 ("Auto Joy 0 Axis X")) -> ()
          n975 = global write "Robot Global Data.vi" "Auto Joy 0 Axis Z"(0.0 ("Auto Joy 0 Axis X")) -> ()
          n976 = global write "Robot Global Data.vi" "Auto Gyro Hold"(TRUE ("Auto Gyro Hold")) -> ()
          n977 = global write "Robot Global Data.vi" "Auto Close Forks"(TRUE ("Auto Gyro Hold")) -> ()
          n978 = global write "Robot Global Data.vi" "Auto State"(3.0 ("Auto State")) -> ()
          n979 = Wait (ms)(milliseconds to wait=u32 500) -> ()  [unwired: 1 out]
        }
        frame #5 {
          # "Wait a min of 2.0sec"
          # "Lift up can to 6000 counts"
          n980 = global write "Robot Global Data.vi" "Auto Joy 0 Axis X"(0.0 ("Auto Joy 0 Axis X")) -> ()
          n981 = global write "Robot Global Data.vi" "Auto Joy 0 Axis Y"(0.0 ("Auto Joy 0 Axis X")) -> ()
          n982 = global write "Robot Global Data.vi" "Auto Joy 0 Axis Z"(0.0 ("Auto Joy 0 Axis X")) -> ()
          n983 = global write "Robot Global Data.vi" "Auto Gyro Hold"(TRUE ("Auto Gyro Hold")) -> ()
          n984 = global write "Robot Global Data.vi" "Auto Close Forks"(FALSE ("Auto Gyro Hold")) -> ()
          n985 = while {
            stop <- w989 stop-if-true
            n986 = global read "Robot Global Data.vi" "Lift Stopped"() -> (w989:bool)
          }
          n987 = global write "Robot Global Data.vi" "Auto Lift Encoder"(6000.0 ("Auto Joy 0 Axis X")) -> ()
          n988 = Wait (ms)(milliseconds to wait=u32 2000) -> ()  [unwired: 1 out]
          n989 = global write "Robot Global Data.vi" "Auto State"(4.0 ("Auto State")) -> ()
        }
        frame #6 {
          # "Drive forward until count = -350"
          n990 = global write "Robot Global Data.vi" "Auto Joy 0 Axis X"(0.0 ("Auto Joy 0 Axis X")) -> ()
          n991 = global write "Robot Global Data.vi" "Auto Joy 0 Axis Y"(-0.25 ("Auto Joy 0 Axis X")) -> ()
          n992 = global write "Robot Global Data.vi" "Auto Joy 0 Axis Z"(0.0 ("Auto Joy 0 Axis X")) -> ()
          n993 = global write "Robot Global Data.vi" "Auto Gyro Hold"(TRUE ("Auto Gyro Hold")) -> ()
          n994 = global write "Robot Global Data.vi" "Lift Encoder Reset"(FALSE ("Auto Gyro Hold")) -> ()
          n995 = global write "Robot Global Data.vi" "Wheel Encoder Reset"(FALSE ("Wheel Encoder Reset")) -> ()
          n996 = while {
            stop <- w997 stop-if-true
            n997 = global read "Robot Global Data.vi" "Wheel Encoder Distance"() -> (w999:dbl)
            n998 = Less Or Equal?(x=w999, y=-350.0) -> (x <= y?=w997:bool)
          }
          n999 = global write "Robot Global Data.vi" "Auto State"(5.0 ("Auto State")) -> ()
        }
        frame #7 {
          # "Ensure at least 0.5sec wait"
          # "Set can on crate"
          n1000 = global write "Robot Global Data.vi" "Auto Joy 0 Axis X"(0.0 ("Auto Joy 0 Axis X")) -> ()
          n1001 = global write "Robot Global Data.vi" "Auto Joy 0 Axis Y"(0.0 ("Auto Joy 0 Axis X")) -> ()
          n1002 = global write "Robot Global Data.vi" "Auto Joy 0 Axis Z"(0.0 ("Auto Joy 0 Axis X")) -> ()
          n1003 = global write "Robot Global Data.vi" "Auto Gyro Hold"(TRUE ("Auto Gyro Hold")) -> ()
          n1004 = while {
            stop <- w1007 stop-if-true
            n1005 = global read "Robot Global Data.vi" "Lift Stopped"() -> (w1007:bool)
          }
          n1006 = global write "Robot Global Data.vi" "Auto Lift Encoder"(5000.0 ("Auto Joy 0 Axis X")) -> ()
          n1007 = Wait (ms)(milliseconds to wait=u32 500) -> ()  [unwired: 1 out]
          n1008 = global write "Robot Global Data.vi" "Auto State"(6.0 ("Auto State")) -> ()
        }
        frame #8 {
          # "Open lift, wait 0.3 sec for lift to open"
          n1009 = global write "Robot Global Data.vi" "Auto Joy 0 Axis X"(0.0 ("Auto Joy 0 Axis X")) -> ()
          n1010 = global write "Robot Global Data.vi" "Auto Joy 0 Axis Y"(0.0 ("Auto Joy 0 Axis X")) -> ()
          n1011 = global write "Robot Global Data.vi" "Auto Joy 0 Axis Z"(0.0 ("Auto Joy 0 Axis X")) -> ()
          n1012 = global write "Robot Global Data.vi" "Auto Gyro Hold"(TRUE ("Auto Gyro Hold")) -> ()
          n1013 = global write "Robot Global Data.vi" "Auto Open Forks"(TRUE ("Auto Gyro Hold")) -> ()
          n1014 = global write "Robot Global Data.vi" "Auto State"(7.0 ("Auto State")) -> ()
          n1015 = Wait (ms)(milliseconds to wait=u32 300) -> ()  [unwired: 1 out]
        }
        frame #9 {
          # "Lower lift to bottom"
          n1016 = global write "Robot Global Data.vi" "Auto Joy 0 Axis X"(0.0 ("Auto Joy 0 Axis X")) -> ()
          n1017 = global write "Robot Global Data.vi" "Auto Joy 0 Axis Y"(0.0 ("Auto Joy 0 Axis X")) -> ()
          n1018 = global write "Robot Global Data.vi" "Auto Joy 0 Axis Z"(0.0 ("Auto Joy 0 Axis X")) -> ()
          n1019 = global write "Robot Global Data.vi" "Auto Gyro Hold"(TRUE ("Auto Gyro Hold")) -> ()
          n1020 = global write "Robot Global Data.vi" "Auto Open Forks"(FALSE ("Auto Gyro Hold")) -> ()
          n1021 = while {
            stop <- w1022 stop-if-true
            n1022 = global read "Robot Global Data.vi" "Bottom Limit"() -> (w1022:bool)
          }
          n1023 = global write "Robot Global Data.vi" "Auto Lift Encoder"(-20000.0 ("Auto Joy 0 Axis X")) -> ()
          n1024 = global write "Robot Global Data.vi" "Auto State"(8.0 ("Auto State")) -> ()
        }
        frame #10 {
          # "Close lift, wait 0.4 sec for lift to close"
          n1025 = global write "Robot Global Data.vi" "Auto Joy 0 Axis X"(0.0 ("Auto Joy 0 Axis X")) -> ()
          n1026 = global write "Robot Global Data.vi" "Auto Joy 0 Axis Y"(0.0 ("Auto Joy 0 Axis X")) -> ()
          n1027 = global write "Robot Global Data.vi" "Auto Joy 0 Axis Z"(0.0 ("Auto Joy 0 Axis X")) -> ()
          n1028 = global write "Robot Global Data.vi" "Auto Gyro Hold"(TRUE ("Auto Gyro Hold")) -> ()
          n1029 = global write "Robot Global Data.vi" "Auto Close Forks"(TRUE ("Auto Gyro Hold")) -> ()
          n1030 = global write "Robot Global Data.vi" "Auto State"(9.0 ("Auto State")) -> ()
          n1031 = Wait (ms)(milliseconds to wait=u32 400) -> ()  [unwired: 1 out]
        }
        frame #11 {
          # "Ensure at least 0.5sec wait"
          # "Lift up can for 1500 counts"
          n1032 = global write "Robot Global Data.vi" "Auto Joy 0 Axis X"(0.0 ("Auto Joy 0 Axis X")) -> ()
          n1033 = global write "Robot Global Data.vi" "Auto Joy 0 Axis Y"(0.0 ("Auto Joy 0 Axis X")) -> ()
          n1034 = global write "Robot Global Data.vi" "Auto Joy 0 Axis Z"(0.0 ("Auto Joy 0 Axis X")) -> ()
          n1035 = global write "Robot Global Data.vi" "Auto Gyro Hold"(TRUE ("Auto Gyro Hold")) -> ()
          n1036 = global write "Robot Global Data.vi" "Auto Close Forks"(FALSE ("Auto Gyro Hold")) -> ()
          n1037 = while {
            stop <- w1038 stop-if-true
            n1038 = global read "Robot Global Data.vi" "Lift Stopped"() -> (w1038:bool)
          }
          n1039 = global write "Robot Global Data.vi" "Auto Lift Encoder"(1500.0 ("Auto Joy 0 Axis X")) -> ()
          n1040 = Wait (ms)(milliseconds to wait=u32 500) -> ()  [unwired: 1 out]
          n1041 = global write "Robot Global Data.vi" "Auto State"(10.0 ("Auto State")) -> ()
        }
        frame #12 {
          # "Wait for robot to finish turning"
          # "Turn robot 90 degrees clockwise"
          n1042 = global write "Robot Global Data.vi" "Auto Joy 0 Axis X"(0.0 ("Auto Joy 0 Axis X")) -> ()
          n1043 = global write "Robot Global Data.vi" "Auto Joy 0 Axis Y"(0.0 ("Auto Joy 0 Axis X")) -> ()
          n1044 = global write "Robot Global Data.vi" "Auto Joy 0 Axis Z"(0.0 ("Auto Joy 0 Axis X")) -> ()
          n1045 = global write "Robot Global Data.vi" "Auto Gyro Hold"(TRUE ("Auto Gyro Hold")) -> ()
          n1046 = global write "Robot Global Data.vi" "Auto Close Forks"(FALSE ("Auto Gyro Hold")) -> ()
          n1047 = global write "Robot Global Data.vi" "PID Target Angle"(-90.0 ("Auto Joy 0 Axis Z")) -> ()
          n1048 = global write "Robot Global Data.vi" "Auto State"(11.0 ("Auto State")) -> ()
          n1049 = Wait (ms)(milliseconds to wait=u32 2000) -> ()  [unwired: 1 out]
        }
        frame #13 {
          # "Reset wheel counter since robot turned,\nhence forward count is incorrect."
          n1050 = global write "Robot Global Data.vi" "Auto Joy 0 Axis X"(0.0 ("Auto Joy 0 Axis X")) -> ()
          n1051 = global write "Robot Global Data.vi" "Auto Joy 0 Axis Y"(0.0 ("Auto Joy 0 Axis X")) -> ()
          n1052 = global write "Robot Global Data.vi" "Auto Joy 0 Axis Z"(0.0 ("Auto Joy 0 Axis X")) -> ()
          n1053 = global write "Robot Global Data.vi" "Auto Gyro Hold"(TRUE ("Auto Gyro Hold")) -> ()
          n1054 = global write "Robot Global Data.vi" "Wheel Encoder Reset"(TRUE ("Wheel Encoder Reset")) -> ()
          n1055 = global write "Robot Global Data.vi" "Auto State"(12.0 ("Auto State")) -> ()
          n1056 = Wait (ms)(milliseconds to wait=u32 50) -> ()  [unwired: 1 out]
        }
        frame #14 {
          # "Enable wheel counter."
          n1057 = global write "Robot Global Data.vi" "Auto Joy 0 Axis X"(0.0 ("Auto Joy 0 Axis X")) -> ()
          n1058 = global write "Robot Global Data.vi" "Auto Joy 0 Axis Y"(0.0 ("Auto Joy 0 Axis X")) -> ()
          n1059 = global write "Robot Global Data.vi" "Auto Joy 0 Axis Z"(0.0 ("Auto Joy 0 Axis X")) -> ()
          n1060 = global write "Robot Global Data.vi" "Auto Gyro Hold"(TRUE ("Auto Gyro Hold")) -> ()
          n1061 = global write "Robot Global Data.vi" "Wheel Encoder Reset"(FALSE ("Wheel Encoder Reset")) -> ()
          n1062 = global write "Robot Global Data.vi" "Auto State"(13.0 ("Auto State")) -> ()
          n1063 = Wait (ms)(milliseconds to wait=u32 50) -> ()  [unwired: 1 out]
        }
        frame #15 {
          # "Drive forward until count = -1700"
          n1064 = global write "Robot Global Data.vi" "Auto Joy 0 Axis X"(0.0 ("Auto Joy 0 Axis X")) -> ()
          n1065 = global write "Robot Global Data.vi" "Auto Joy 0 Axis Y"(-0.4 ("Auto Joy 0 Axis X")) -> ()
          n1066 = global write "Robot Global Data.vi" "Auto Joy 0 Axis Z"(0.0 ("Auto Joy 0 Axis X")) -> ()
          n1067 = global write "Robot Global Data.vi" "Auto Gyro Hold"(TRUE ("Auto Gyro Hold")) -> ()
          n1068 = global write "Robot Global Data.vi" "Wheel Encoder Reset"(FALSE ("Wheel Encoder Reset")) -> ()
          n1069 = while {
            stop <- w1069 stop-if-true
            n1070 = global read "Robot Global Data.vi" "Wheel Encoder Distance"() -> (w1068:dbl)
            n1071 = Less Or Equal?(x=w1068, y=-1700.0) -> (x <= y?=w1069:bool)
          }
          n1072 = global write "Robot Global Data.vi" "Auto State"(14.0 ("Auto State")) -> ()
        }
        frame #16 {
          # "100 is an inch above bottom limit switch\nNote: Trash Can keeps forks from engaing bottom limit\nswitch so use encoder!!!!"
          # "Stop robot, lower crate"
          n1073 = global write "Robot Global Data.vi" "Auto Joy 0 Axis X"(0.0 ("Auto Joy 0 Axis X")) -> ()
          n1074 = global write "Robot Global Data.vi" "Auto Joy 0 Axis Y"(0.0 ("Auto Joy 0 Axis X")) -> ()
          n1075 = global write "Robot Global Data.vi" "Auto Joy 0 Axis Z"(0.0 ("Auto Joy 0 Axis X")) -> ()
          n1076 = global write "Robot Global Data.vi" "Auto Gyro Hold"(TRUE ("Auto Gyro Hold")) -> ()
          n1077 = while {
            stop <- w1076 stop-if-true
            n1078 = global read "Robot Global Data.vi" "Lift Encoder Distance"() -> (w1078:dbl)
            n1079 = Less Or Equal?(x=w1078, y=100.0) -> (x <= y?=w1076:bool)
          }
          n1080 = global write "Robot Global Data.vi" "Auto Lift Encoder"(-200.0 ("Auto Joy 0 Axis X")) -> ()
          n1081 = global write "Robot Global Data.vi" "Auto State"(15.0 ("Auto State")) -> ()
        }
        frame #17 {
          # "Open lift, wait 0.3 sec for lift to open"
          n1082 = global write "Robot Global Data.vi" "Auto Joy 0 Axis X"(0.0 ("Auto Joy 0 Axis X")) -> ()
          n1083 = global write "Robot Global Data.vi" "Auto Joy 0 Axis Y"(0.0 ("Auto Joy 0 Axis X")) -> ()
          n1084 = global write "Robot Global Data.vi" "Auto Joy 0 Axis Z"(0.0 ("Auto Joy 0 Axis X")) -> ()
          n1085 = global write "Robot Global Data.vi" "Auto Gyro Hold"(TRUE ("Auto Gyro Hold")) -> ()
          n1086 = global write "Robot Global Data.vi" "Auto Open Forks"(TRUE ("Auto Gyro Hold")) -> ()
          n1087 = global write "Robot Global Data.vi" "Auto State"(16.0 ("Auto State")) -> ()
          n1088 = Wait (ms)(milliseconds to wait=u32 300) -> ()  [unwired: 1 out]
        }
        frame #18 {
          # "Drive backward until count = -1900"
          n1089 = global write "Robot Global Data.vi" "Auto Joy 0 Axis X"(0.0 ("Auto Joy 0 Axis X")) -> ()
          n1090 = global write "Robot Global Data.vi" "Auto Joy 0 Axis Y"(0.2 ("Auto Joy 0 Axis X")) -> ()
          n1091 = global write "Robot Global Data.vi" "Auto Joy 0 Axis Z"(0.0 ("Auto Joy 0 Axis X")) -> ()
          n1092 = global write "Robot Global Data.vi" "Auto Gyro Hold"(TRUE ("Auto Gyro Hold")) -> ()
          n1093 = global write "Robot Global Data.vi" "Auto Open Forks"(FALSE ("Auto Gyro Hold")) -> ()
          n1094 = while {
            stop <- w1094 stop-if-true
            n1095 = global read "Robot Global Data.vi" "Wheel Encoder Distance"() -> (w1093:dbl)
            n1096 = Greater Or Equal?(x=w1093, y=-1900.0) -> (x >= y?=w1094:bool)
          }
          n1097 = global write "Robot Global Data.vi" "Auto State"(17.0 ("Auto State")) -> ()
        }
        frame #19 {
          # "Stop and wait until teleop"
          n1098 = global write "Robot Global Data.vi" "Auto Joy 0 Axis X"(0.0 ("Auto Joy 0 Axis X")) -> ()
          n1099 = global write "Robot Global Data.vi" "Auto Joy 0 Axis Y"(0.0 ("Auto Joy 0 Axis X")) -> ()
          n1100 = global write "Robot Global Data.vi" "Auto Joy 0 Axis Z"(0.0 ("Auto Joy 0 Axis X")) -> ()
          n1101 = global write "Robot Global Data.vi" "Auto Gyro Hold"(FALSE ("Auto Gyro Hold")) -> ()
          n1102 = global write "Robot Global Data.vi" "Auto State"(18.0 ("Auto State")) -> ()
          n1103 = Wait (ms)(milliseconds to wait=u32 15000) -> ()  [unwired: 1 out]
        }
      }
    }
  }
  n1104 = case shown="True" w18 {
    frame False {
    }
    frame True {
      n1105 = stacked-sequence {
        frame #0 {
          # "Reset encoders"
          # "Reset Gyro"
          # "Initialize"
          n1106 = global write "Robot Global Data.vi" "Auto Joy 1 Axis Y"(0.0 ("Auto Joy 0 Axis X")) -> ()
          n1107 = global write "Robot Global Data.vi" "Auto Joy 0 Axis X"(0.0 ("Auto Joy 0 Axis X")) -> ()
          n1108 = global write "Robot Global Data.vi" "Auto Joy 0 Axis Y"(0.0 ("Auto Joy 0 Axis X")) -> ()
          n1109 = global write "Robot Global Data.vi" "Auto Joy 0 Axis Z"(0.0 ("Auto Joy 0 Axis X")) -> ()
          n1110 = global write "Robot Global Data.vi" "Gyro Reset"(TRUE ("Auto Gyro Hold")) -> ()
          n1111 = global write "Robot Global Data.vi" "Lift Encoder Reset"(TRUE ("Auto Gyro Hold")) -> ()
          n1112 = global write "Robot Global Data.vi" "Wheel Encoder Reset"(TRUE ("Wheel Encoder Reset")) -> ()
          n1113 = global write "Robot Global Data.vi" "Auto Gyro Hold"(FALSE ("Auto Gyro Hold")) -> ()
          n1114 = global write "Robot Global Data.vi" "Auto Open Forks"(FALSE ("Auto Gyro Hold")) -> ()
          n1115 = global write "Robot Global Data.vi" "Auto Close Forks"(FALSE ("Auto Gyro Hold")) -> ()
          n1116 = global write "Robot Global Data.vi" "PID Target Angle"(0.0 ("Auto Joy 0 Axis Z")) -> ()
          n1117 = global write "Robot Global Data.vi" "Raw Gyro Angle"(0.0 ("Auto Joy 0 Axis Z")) -> ()
          n1118 = global write "Robot Global Data.vi" "Auto State"(0.0 ("Auto State")) -> ()
          n1119 = Wait (ms)(milliseconds to wait=u32 50) -> ()  [unwired: 1 out]
        }
        frame #1 {
          # "Reset encoders"
          # "Reset Gyro"
          # "Initialize"
          n1120 = global write "Robot Global Data.vi" "Auto Joy 0 Axis X"(0.0 ("Auto Joy 0 Axis X")) -> ()
          n1121 = global write "Robot Global Data.vi" "Auto Joy 0 Axis Y"(0.0 ("Auto Joy 0 Axis X")) -> ()
          n1122 = global write "Robot Global Data.vi" "Auto Joy 0 Axis Z"(0.0 ("Auto Joy 0 Axis X")) -> ()
          n1123 = global write "Robot Global Data.vi" "Gyro Reset"(FALSE ("Auto Gyro Hold")) -> ()
          n1124 = global write "Robot Global Data.vi" "Lift Encoder Reset"(FALSE ("Auto Gyro Hold")) -> ()
          n1125 = global write "Robot Global Data.vi" "Wheel Encoder Reset"(FALSE ("Wheel Encoder Reset")) -> ()
          n1126 = global write "Robot Global Data.vi" "Auto State"(0.0 ("Auto State")) -> ()
          n1127 = Wait (ms)(milliseconds to wait=u32 50) -> ()  [unwired: 1 out]
        }
        frame #2 {
          # "Enable Gyro Hold"
          n1128 = global write "Robot Global Data.vi" "Auto Joy 0 Axis X"(0.0 ("Auto Joy 0 Axis X")) -> ()
          n1129 = global write "Robot Global Data.vi" "Auto Joy 0 Axis Z"(0.0 ("Auto Joy 0 Axis X")) -> ()
          n1130 = global write "Robot Global Data.vi" "Auto Gyro Hold"(TRUE ("Auto Gyro Hold")) -> ()
          n1131 = global write "Robot Global Data.vi" "Lift Encoder Reset"(FALSE ("Auto Gyro Hold")) -> ()
          n1132 = global write "Robot Global Data.vi" "Wheel Encoder Reset"(FALSE ("Wheel Encoder Reset")) -> ()
          n1133 = global write "Robot Global Data.vi" "Auto State"(1.0 ("Auto State")) -> ()
          n1134 = Wait (ms)(milliseconds to wait=u32 50) -> ()  [unwired: 1 out]
        }
        frame #3 {
          # "Wait 0.4sec for forks to close"
          # "Close lift"
          n1135 = global write "Robot Global Data.vi" "Auto Joy 0 Axis X"(0.0 ("Auto Joy 0 Axis X")) -> ()
          n1136 = global write "Robot Global Data.vi" "Auto Joy 0 Axis Z"(0.0 ("Auto Joy 0 Axis X")) -> ()
          n1137 = global write "Robot Global Data.vi" "Auto Gyro Hold"(TRUE ("Auto Gyro Hold")) -> ()
          n1138 = global write "Robot Global Data.vi" "Auto Close Forks"(TRUE ("Auto Gyro Hold")) -> ()
          n1139 = global write "Robot Global Data.vi" "Auto State"(2.0 ("Auto State")) -> ()
          n1140 = Wait (ms)(milliseconds to wait=u32 400) -> ()  [unwired: 1 out]
        }
        frame #4 {
          # "Turn robot 35 degrees counterclockwise\nHold wheel encoder in reset"
          n1141 = global write "Robot Global Data.vi" "Wheel Encoder Reset"(TRUE ("Wheel Encoder Reset")) -> ()
          n1142 = global write "Robot Global Data.vi" "Auto Close Forks"(FALSE ("Auto Gyro Hold")) -> ()
          n1143 = global write "Robot Global Data.vi" "PID Target Angle"(-35.0 ("Auto Joy 0 Axis Z")) -> ()
          n1144 = global write "Robot Global Data.vi" "Auto State"(3.0 ("Auto State")) -> ()
          n1145 = Wait (ms)(milliseconds to wait=u32 400) -> ()  [unwired: 1 out]
        }
        frame #5 {
          # "Drive forward"
          n1146 = global write "Robot Global Data.vi" "Auto Joy 0 Axis X"(0.0 ("Auto Joy 0 Axis X")) -> ()
          n1147 = global write "Robot Global Data.vi" "Auto Joy 0 Axis Y"(-0.3 ("Auto Joy 0 Axis Y")) -> ()
          n1148 = global write "Robot Global Data.vi" "Auto Joy 0 Axis Z"(0.0 ("Auto Joy 0 Axis X")) -> ()
          n1149 = global write "Robot Global Data.vi" "Auto Gyro Hold"(TRUE ("Auto Gyro Hold")) -> ()
          n1150 = global write "Robot Global Data.vi" "Lift Encoder Reset"(FALSE ("Auto Gyro Hold")) -> ()
          n1151 = global write "Robot Global Data.vi" "Wheel Encoder Reset"(FALSE ("Wheel Encoder Reset")) -> ()
          n1152 = while {
            stop <- w1149 stop-if-true
            n1153 = global read "Robot Global Data.vi" "Wheel Encoder Distance"() -> (w1150:dbl)
            n1154 = Less Or Equal?(x=w1150, y=-200.0) -> (x <= y?=w1149:bool)
          }
          n1155 = global write "Robot Global Data.vi" "Auto State"(4.0 ("Auto State")) -> ()
        }
        frame #6 {
          # "Drive forward, turn robot to +35 degrees clockwise, raise lift to 7000 counts"
          n1156 = global write "Robot Global Data.vi" "Auto Joy 0 Axis X"(0.0 ("Auto Joy 0 Axis X")) -> ()
          n1157 = global write "Robot Global Data.vi" "Auto Joy 0 Axis Y"(-0.3 ("Auto Joy 0 Axis Y")) -> ()
          n1158 = global write "Robot Global Data.vi" "Auto Joy 0 Axis Z"(0.0 ("Auto Joy 0 Axis X")) -> ()
          n1159 = global write "Robot Global Data.vi" "Auto Gyro Hold"(TRUE ("Auto Gyro Hold")) -> ()
          n1160 = global write "Robot Global Data.vi" "Lift Encoder Reset"(FALSE ("Auto Gyro Hold")) -> ()
          n1161 = global write "Robot Global Data.vi" "Wheel Encoder Reset"(FALSE ("Wheel Encoder Reset")) -> ()
          n1162 = while {
            stop <- w1161 stop-if-true
            n1163 = global read "Robot Global Data.vi" "Wheel Encoder Distance"() -> (w1162:dbl)
            n1164 = Less Or Equal?(x=w1162, y=-1625.0) -> (x <= y?=w1161:bool)
          }
          n1165 = global write "Robot Global Data.vi" "PID Target Angle"(35.0 ("Auto Joy 0 Axis Z")) -> ()
          n1166 = global write "Robot Global Data.vi" "Auto Lift Encoder"(7000.0 ("Auto Lift Encoder")) -> ()
          n1167 = global write "Robot Global Data.vi" "Auto State"(5.0 ("Auto State")) -> ()
        }
        frame #7 {
          # "Turn robot to 0 degrees and \ndrive forward until count = -1800"
          n1168 = global write "Robot Global Data.vi" "Auto Joy 0 Axis X"(0.0 ("Auto Joy 0 Axis X")) -> ()
          n1169 = global write "Robot Global Data.vi" "Auto Joy 0 Axis Z"(0.0 ("Auto Joy 0 Axis X")) -> ()
          n1170 = global write "Robot Global Data.vi" "Auto Gyro Hold"(TRUE ("Auto Gyro Hold")) -> ()
          n1171 = global write "Robot Global Data.vi" "Lift Encoder Reset"(FALSE ("Auto Gyro Hold")) -> ()
          n1172 = global write "Robot Global Data.vi" "Wheel Encoder Reset"(FALSE ("Wheel Encoder Reset")) -> ()
          n1173 = while {
            stop <- w1171 stop-if-true
            n1174 = global read "Robot Global Data.vi" "Wheel Encoder Distance"() -> (w1172:dbl)
            n1175 = Less Or Equal?(x=w1172, y=-1800.0) -> (x <= y?=w1171:bool)
          }
          n1176 = global write "Robot Global Data.vi" "PID Target Angle"(0.0 ("Auto Joy 0 Axis Z")) -> ()
          n1177 = global write "Robot Global Data.vi" "Auto State"(6.0 ("Auto State")) -> ()
        }
        frame #8 {
          # "Ensure at least 0.5sec wait while crate1 gets lowered onto crate 2."
          # "Set crate1 on crate2"
          n1178 = global write "Robot Global Data.vi" "Auto Joy 0 Axis X"(0.0 ("Auto Joy 0 Axis X")) -> ()
          n1179 = global write "Robot Global Data.vi" "Auto Joy 0 Axis Y"(0.0 ("Auto Joy 0 Axis X")) -> ()
          n1180 = global write "Robot Global Data.vi" "Auto Joy 0 Axis Z"(0.0 ("Auto Joy 0 Axis X")) -> ()
          n1181 = global write "Robot Global Data.vi" "Auto Gyro Hold"(TRUE ("Auto Gyro Hold")) -> ()
          n1182 = while {
            stop <- w1180 stop-if-true
            n1183 = global read "Robot Global Data.vi" "Lift Stopped"() -> (w1180:bool)
          }
          n1184 = global write "Robot Global Data.vi" "Auto Lift Encoder"(5400.0 ("Auto Lift Encoder")) -> ()
          n1185 = Wait (ms)(milliseconds to wait=u32 400) -> ()  [unwired: 1 out]
          n1186 = global write "Robot Global Data.vi" "Auto State"(7.0 ("Auto State")) -> ()
        }
        frame #9 {
          # "Open lift, wait 0.25 sec for lift to open"
          n1187 = global write "Robot Global Data.vi" "Auto Joy 0 Axis X"(0.0 ("Auto Joy 0 Axis X")) -> ()
          n1188 = global write "Robot Global Data.vi" "Auto Joy 0 Axis Y"(0.0 ("Auto Joy 0 Axis X")) -> ()
          n1189 = global write "Robot Global Data.vi" "Auto Joy 0 Axis Z"(0.0 ("Auto Joy 0 Axis X")) -> ()
          n1190 = global write "Robot Global Data.vi" "Auto Gyro Hold"(TRUE ("Auto Gyro Hold")) -> ()
          n1191 = global write "Robot Global Data.vi" "Auto Open Forks"(TRUE ("Auto Gyro Hold")) -> ()
          n1192 = global write "Robot Global Data.vi" "Auto State"(8.0 ("Auto State")) -> ()
          n1193 = Wait (ms)(milliseconds to wait=u32 250) -> ()  [unwired: 1 out]
        }
        frame #10 {
          # "100 is an inch above bottom limit switch"
          # "Lower lift to bottom"
          n1194 = global write "Robot Global Data.vi" "Auto Joy 0 Axis X"(0.0 ("Auto Joy 0 Axis X")) -> ()
          n1195 = global write "Robot Global Data.vi" "Auto Joy 0 Axis Y"(0.0 ("Auto Joy 0 Axis X")) -> ()
          n1196 = global write "Robot Global Data.vi" "Auto Joy 0 Axis Z"(0.0 ("Auto Joy 0 Axis X")) -> ()
          n1197 = global write "Robot Global Data.vi" "Auto Gyro Hold"(TRUE ("Auto Gyro Hold")) -> ()
          n1198 = global write "Robot Global Data.vi" "Auto Open Forks"(FALSE ("Auto Gyro Hold")) -> ()
          n1199 = while {
            stop <- w1195 stop-if-true
            n1200 = global read "Robot Global Data.vi" "Lift Encoder Distance"() -> (w1197:dbl)
            n1201 = Less Or Equal?(x=w1197, y=100.0) -> (x <= y?=w1195:bool)
          }
          n1202 = global write "Robot Global Data.vi" "Auto Lift Encoder"(-200.0 ("Auto Joy 0 Axis X")) -> ()
          n1203 = global write "Robot Global Data.vi" "Auto State"(9.0 ("Auto State")) -> ()
        }
        frame #11 {
          # "Close lift, wait 0.4 sec for lift to close"
          n1204 = global write "Robot Global Data.vi" "Auto Joy 0 Axis X"(0.0 ("Auto Joy 0 Axis X")) -> ()
          n1205 = global write "Robot Global Data.vi" "Auto Joy 0 Axis Y"(0.0 ("Auto Joy 0 Axis X")) -> ()
          n1206 = global write "Robot Global Data.vi" "Auto Joy 0 Axis Z"(0.0 ("Auto Joy 0 Axis X")) -> ()
          n1207 = global write "Robot Global Data.vi" "Auto Gyro Hold"(TRUE ("Auto Gyro Hold")) -> ()
          n1208 = global write "Robot Global Data.vi" "Auto Close Forks"(TRUE ("Auto Gyro Hold")) -> ()
          n1209 = global write "Robot Global Data.vi" "Auto State"(10.0 ("Auto State")) -> ()
          n1210 = Wait (ms)(milliseconds to wait=u32 400) -> ()  [unwired: 1 out]
        }
        frame #12 {
          # "Crate lift was here but now taken out"
          n1211 = global write "Robot Global Data.vi" "Auto Joy 0 Axis X"(0.0 ("Auto Joy 0 Axis X")) -> ()
          n1212 = global write "Robot Global Data.vi" "Auto Joy 0 Axis Y"(0.0 ("Auto Joy 0 Axis X")) -> ()
          n1213 = global write "Robot Global Data.vi" "Auto Joy 0 Axis Z"(0.0 ("Auto Joy 0 Axis X")) -> ()
          n1214 = global write "Robot Global Data.vi" "Auto Gyro Hold"(TRUE ("Auto Gyro Hold")) -> ()
          n1215 = global write "Robot Global Data.vi" "Auto Close Forks"(FALSE ("Auto Gyro Hold")) -> ()
          n1216 = while {
            stop <- w1213 stop-if-true
            n1217 = global read "Robot Global Data.vi" "Lift Stopped"() -> (w1213:bool)
          }
          n1218 = global write "Robot Global Data.vi" "Auto Lift Encoder"(0.0 ("Auto Joy 0 Axis X")) -> ()
          n1219 = Wait (ms)(milliseconds to wait=u32 50) -> ()  [unwired: 1 out]
          n1220 = global write "Robot Global Data.vi" "Auto State"(11.0 ("Auto State")) -> ()
        }
        frame #13 {
          # "Wait for robot to finish turning"
          # "Turn robot 90 degrees clockwise"
          n1221 = global write "Robot Global Data.vi" "Auto Joy 0 Axis X"(0.0 ("Auto Joy 0 Axis X")) -> ()
          n1222 = global write "Robot Global Data.vi" "Auto Joy 0 Axis Y"(0.0 ("Auto Joy 0 Axis X")) -> ()
          n1223 = global write "Robot Global Data.vi" "Auto Joy 0 Axis Z"(0.0 ("Auto Joy 0 Axis X")) -> ()
          n1224 = global write "Robot Global Data.vi" "Auto Gyro Hold"(TRUE ("Auto Gyro Hold")) -> ()
          n1225 = global write "Robot Global Data.vi" "Auto Close Forks"(FALSE ("Auto Gyro Hold")) -> ()
          n1226 = global write "Robot Global Data.vi" "PID Target Angle"(90.0 ("Auto Joy 0 Axis Z")) -> ()
          n1227 = global write "Robot Global Data.vi" "Auto State"(12.0 ("Auto State")) -> ()
          n1228 = Wait (ms)(milliseconds to wait=u32 1300) -> ()  [unwired: 1 out]
        }
        frame #14 {
          # "Reset wheel counter since robot turned,\nhence forward count is incorrect."
          n1229 = global write "Robot Global Data.vi" "Auto Joy 0 Axis X"(0.0 ("Auto Joy 0 Axis X")) -> ()
          n1230 = global write "Robot Global Data.vi" "Auto Joy 0 Axis Y"(0.0 ("Auto Joy 0 Axis X")) -> ()
          n1231 = global write "Robot Global Data.vi" "Auto Joy 0 Axis Z"(0.0 ("Auto Joy 0 Axis X")) -> ()
          n1232 = global write "Robot Global Data.vi" "Auto Gyro Hold"(TRUE ("Auto Gyro Hold")) -> ()
          n1233 = global write "Robot Global Data.vi" "Wheel Encoder Reset"(TRUE ("Wheel Encoder Reset")) -> ()
          n1234 = global write "Robot Global Data.vi" "Auto State"(13.0 ("Auto State")) -> ()
          n1235 = Wait (ms)(milliseconds to wait=u32 50) -> ()  [unwired: 1 out]
        }
        frame #15 {
          # "Enable wheel counter."
          n1236 = global write "Robot Global Data.vi" "Auto Joy 0 Axis X"(0.0 ("Auto Joy 0 Axis X")) -> ()
          n1237 = global write "Robot Global Data.vi" "Auto Joy 0 Axis Y"(0.0 ("Auto Joy 0 Axis X")) -> ()
          n1238 = global write "Robot Global Data.vi" "Auto Joy 0 Axis Z"(0.0 ("Auto Joy 0 Axis X")) -> ()
          n1239 = global write "Robot Global Data.vi" "Auto Gyro Hold"(TRUE ("Auto Gyro Hold")) -> ()
          n1240 = global write "Robot Global Data.vi" "Wheel Encoder Reset"(FALSE ("Wheel Encoder Reset")) -> ()
          n1241 = global write "Robot Global Data.vi" "Auto State"(14.0 ("Auto State")) -> ()
          n1242 = Wait (ms)(milliseconds to wait=u32 50) -> ()  [unwired: 1 out]
        }
        frame #16 {
          # "Drive forward until count = -1950\n(was -2050)"
          n1243 = global write "Robot Global Data.vi" "Auto Joy 0 Axis X"(0.0 ("Auto Joy 0 Axis X")) -> ()
          n1244 = global write "Robot Global Data.vi" "Auto Joy 0 Axis Y"(-0.4 ("Auto Joy 0 Axis Y")) -> ()
          n1245 = global write "Robot Global Data.vi" "Auto Joy 0 Axis Z"(0.0 ("Auto Joy 0 Axis X")) -> ()
          n1246 = global write "Robot Global Data.vi" "Auto Gyro Hold"(TRUE ("Auto Gyro Hold")) -> ()
          n1247 = global write "Robot Global Data.vi" "Wheel Encoder Reset"(FALSE ("Wheel Encoder Reset")) -> ()
          n1248 = while {
            stop <- w1243 stop-if-true
            n1249 = global read "Robot Global Data.vi" "Wheel Encoder Distance"() -> (w1244:dbl)
            n1250 = Less Or Equal?(x=w1244, y=-1950.0) -> (x <= y?=w1243:bool)
          }
          n1251 = global write "Robot Global Data.vi" "Auto State"(15.0 ("Auto State")) -> ()
        }
        frame #17 {
          # "100 is an inch above bottom limit switch\nNote: Trash Can keeps forks from engaing bottom limit\nswitch so use encoder!!!!"
          # "Stop robot, lower crate"
          n1252 = global write "Robot Global Data.vi" "Auto Joy 0 Axis X"(0.0 ("Auto Joy 0 Axis X")) -> ()
          n1253 = global write "Robot Global Data.vi" "Auto Joy 0 Axis Y"(0.0 ("Auto Joy 0 Axis X")) -> ()
          n1254 = global write "Robot Global Data.vi" "Auto Joy 0 Axis Z"(0.0 ("Auto Joy 0 Axis X")) -> ()
          n1255 = global write "Robot Global Data.vi" "Auto Gyro Hold"(TRUE ("Auto Gyro Hold")) -> ()
          n1256 = while {
            stop <- w1251 stop-if-true
            n1257 = global read "Robot Global Data.vi" "Lift Encoder Distance"() -> (w1253:dbl)
            n1258 = Less Or Equal?(x=w1253, y=100.0) -> (x <= y?=w1251:bool)
          }
          n1259 = global write "Robot Global Data.vi" "Auto Lift Encoder"(-200.0 ("Auto Joy 0 Axis X")) -> ()
          n1260 = global write "Robot Global Data.vi" "Auto State"(16.0 ("Auto State")) -> ()
        }
        frame #18 {
          # "Open lift, wait 0.3 sec for lift to open"
          n1261 = global write "Robot Global Data.vi" "Auto Joy 0 Axis X"(0.0 ("Auto Joy 0 Axis X")) -> ()
          n1262 = global write "Robot Global Data.vi" "Auto Joy 0 Axis Y"(0.0 ("Auto Joy 0 Axis X")) -> ()
          n1263 = global write "Robot Global Data.vi" "Auto Joy 0 Axis Z"(0.0 ("Auto Joy 0 Axis X")) -> ()
          n1264 = global write "Robot Global Data.vi" "Auto Gyro Hold"(TRUE ("Auto Gyro Hold")) -> ()
          n1265 = global write "Robot Global Data.vi" "Auto Open Forks"(TRUE ("Auto Gyro Hold")) -> ()
          n1266 = global write "Robot Global Data.vi" "Auto State"(17.0 ("Auto State")) -> ()
          n1267 = Wait (ms)(milliseconds to wait=u32 300) -> ()  [unwired: 1 out]
        }
        frame #19 {
          # "Drive backward until count = -2050\n(was -2250)"
          n1268 = global write "Robot Global Data.vi" "Auto Joy 0 Axis X"(0.0 ("Auto Joy 0 Axis X")) -> ()
          n1269 = global write "Robot Global Data.vi" "Auto Joy 0 Axis Y"(0.2 ("Auto Joy 0 Axis X")) -> ()
          n1270 = global write "Robot Global Data.vi" "Auto Joy 0 Axis Z"(0.0 ("Auto Joy 0 Axis X")) -> ()
          n1271 = global write "Robot Global Data.vi" "Auto Gyro Hold"(TRUE ("Auto Gyro Hold")) -> ()
          n1272 = global write "Robot Global Data.vi" "Auto Open Forks"(FALSE ("Auto Gyro Hold")) -> ()
          n1273 = while {
            stop <- w1269 stop-if-true
            n1274 = global read "Robot Global Data.vi" "Wheel Encoder Distance"() -> (w1268:dbl)
            n1275 = Greater Or Equal?(x=w1268, y=-2050.0) -> (x >= y?=w1269:bool)
          }
          n1276 = global write "Robot Global Data.vi" "Auto State"(18.0 ("Auto State")) -> ()
        }
        frame #20 {
          # "Stop and wait until teleop"
          n1277 = global write "Robot Global Data.vi" "Auto Joy 0 Axis X"(0.0 ("Auto Joy 0 Axis X")) -> ()
          n1278 = global write "Robot Global Data.vi" "Auto Joy 0 Axis Y"(0.0 ("Auto Joy 0 Axis X")) -> ()
          n1279 = global write "Robot Global Data.vi" "Auto Joy 0 Axis Z"(0.0 ("Auto Joy 0 Axis X")) -> ()
          n1280 = global write "Robot Global Data.vi" "Auto Gyro Hold"(FALSE ("Auto Gyro Hold")) -> ()
          n1281 = global write "Robot Global Data.vi" "Auto State"(19.0 ("Auto State")) -> ()
          n1282 = Wait (ms)(milliseconds to wait=u32 15000) -> ()  [unwired: 1 out]
        }
      }
    }
  }
  n1283 = case shown="True" w16 {
    frame False {
    }
    frame True {
      n1284 = stacked-sequence {
        frame #0 {
          # "Reset encoders"
          # "Reset Gyro"
          # "Initialize"
          n1285 = global write "Robot Global Data.vi" "Auto Joy 1 Axis Y"(0.0 ("Auto Joy 0 Axis X")) -> ()
          n1286 = global write "Robot Global Data.vi" "Auto Joy 0 Axis X"(0.0 ("Auto Joy 0 Axis X")) -> ()
          n1287 = global write "Robot Global Data.vi" "Auto Joy 0 Axis Y"(0.0 ("Auto Joy 0 Axis X")) -> ()
          n1288 = global write "Robot Global Data.vi" "Auto Joy 0 Axis Z"(0.0 ("Auto Joy 0 Axis X")) -> ()
          n1289 = global write "Robot Global Data.vi" "Gyro Reset"(TRUE ("Auto Gyro Hold")) -> ()
          n1290 = global write "Robot Global Data.vi" "Lift Encoder Reset"(TRUE ("Auto Gyro Hold")) -> ()
          n1291 = global write "Robot Global Data.vi" "Wheel Encoder Reset"(TRUE ("Wheel Encoder Reset")) -> ()
          n1292 = global write "Robot Global Data.vi" "Auto Gyro Hold"(FALSE ("Auto Gyro Hold")) -> ()
          n1293 = global write "Robot Global Data.vi" "Auto Open Forks"(FALSE ("Auto Gyro Hold")) -> ()
          n1294 = global write "Robot Global Data.vi" "Auto Close Forks"(FALSE ("Auto Gyro Hold")) -> ()
          n1295 = global write "Robot Global Data.vi" "PID Target Angle"(0.0 ("Auto Joy 0 Axis Z")) -> ()
          n1296 = global write "Robot Global Data.vi" "Raw Gyro Angle"(0.0 ("Auto Joy 0 Axis Z")) -> ()
          n1297 = global write "Robot Global Data.vi" "Auto State"(0.0 ("Auto State")) -> ()
          n1298 = Wait (ms)(milliseconds to wait=u32 50) -> ()  [unwired: 1 out]
        }
        frame #1 {
          # "Reset encoders"
          # "Reset Gyro"
          # "Initialize"
          n1299 = global write "Robot Global Data.vi" "Auto Joy 0 Axis X"(0.0 ("Auto Joy 0 Axis X")) -> ()
          n1300 = global write "Robot Global Data.vi" "Auto Joy 0 Axis Y"(0.0 ("Auto Joy 0 Axis X")) -> ()
          n1301 = global write "Robot Global Data.vi" "Auto Joy 0 Axis Z"(0.0 ("Auto Joy 0 Axis X")) -> ()
          n1302 = global write "Robot Global Data.vi" "Gyro Reset"(FALSE ("Auto Gyro Hold")) -> ()
          n1303 = global write "Robot Global Data.vi" "Lift Encoder Reset"(FALSE ("Auto Gyro Hold")) -> ()
          n1304 = global write "Robot Global Data.vi" "Wheel Encoder Reset"(FALSE ("Wheel Encoder Reset")) -> ()
          n1305 = global write "Robot Global Data.vi" "Auto State"(0.0 ("Auto State")) -> ()
          n1306 = Wait (ms)(milliseconds to wait=u32 50) -> ()  [unwired: 1 out]
        }
        frame #2 {
          # "Enable Gyro Hold"
          n1307 = global write "Robot Global Data.vi" "Auto Joy 0 Axis X"(0.0 ("Auto Joy 0 Axis X")) -> ()
          n1308 = global write "Robot Global Data.vi" "Auto Joy 0 Axis Z"(0.0 ("Auto Joy 0 Axis X")) -> ()
          n1309 = global write "Robot Global Data.vi" "Auto Gyro Hold"(TRUE ("Auto Gyro Hold")) -> ()
          n1310 = global write "Robot Global Data.vi" "Lift Encoder Reset"(FALSE ("Auto Gyro Hold")) -> ()
          n1311 = global write "Robot Global Data.vi" "Wheel Encoder Reset"(FALSE ("Wheel Encoder Reset")) -> ()
          n1312 = global write "Robot Global Data.vi" "Auto State"(1.0 ("Auto State")) -> ()
          n1313 = Wait (ms)(milliseconds to wait=u32 50) -> ()  [unwired: 1 out]
        }
        frame #3 {
          # "Wait 0.4sec for forks to close"
          # "Close lift"
          n1314 = global write "Robot Global Data.vi" "Auto Joy 0 Axis X"(0.0 ("Auto Joy 0 Axis X")) -> ()
          n1315 = global write "Robot Global Data.vi" "Auto Joy 0 Axis Z"(0.0 ("Auto Joy 0 Axis X")) -> ()
          n1316 = global write "Robot Global Data.vi" "Auto Gyro Hold"(TRUE ("Auto Gyro Hold")) -> ()
          n1317 = global write "Robot Global Data.vi" "Auto Close Forks"(TRUE ("Auto Gyro Hold")) -> ()
          n1318 = global write "Robot Global Data.vi" "Auto State"(2.0 ("Auto State")) -> ()
          n1319 = Wait (ms)(milliseconds to wait=u32 400) -> ()  [unwired: 1 out]
        }
        frame #4 {
          # "Turn robot 35 degrees counterclockwise\nHold wheel encoder in reset"
          n1320 = global write "Robot Global Data.vi" "Wheel Encoder Reset"(TRUE ("Wheel Encoder Reset")) -> ()
          n1321 = global write "Robot Global Data.vi" "Auto Close Forks"(FALSE ("Auto Gyro Hold")) -> ()
          n1322 = global write "Robot Global Data.vi" "PID Target Angle"(-35.0 ("Auto Joy 0 Axis Z")) -> ()
          n1323 = global write "Robot Global Data.vi" "Auto State"(3.0 ("Auto State")) -> ()
          n1324 = Wait (ms)(milliseconds to wait=u32 400) -> ()  [unwired: 1 out]
        }
        frame #5 {
          # "Drive forward"
          n1325 = global write "Robot Global Data.vi" "Auto Joy 0 Axis X"(0.0 ("Auto Joy 0 Axis X")) -> ()
          n1326 = global write "Robot Global Data.vi" "Auto Joy 0 Axis Y"(-0.3 ("Auto Joy 0 Axis Y")) -> ()
          n1327 = global write "Robot Global Data.vi" "Auto Joy 0 Axis Z"(0.0 ("Auto Joy 0 Axis X")) -> ()
          n1328 = global write "Robot Global Data.vi" "Auto Gyro Hold"(TRUE ("Auto Gyro Hold")) -> ()
          n1329 = global write "Robot Global Data.vi" "Lift Encoder Reset"(FALSE ("Auto Gyro Hold")) -> ()
          n1330 = global write "Robot Global Data.vi" "Wheel Encoder Reset"(FALSE ("Wheel Encoder Reset")) -> ()
          n1331 = while {
            stop <- w1324 stop-if-true
            n1332 = global read "Robot Global Data.vi" "Wheel Encoder Distance"() -> (w1325:dbl)
            n1333 = Less Or Equal?(x=w1325, y=-200.0) -> (x <= y?=w1324:bool)
          }
          n1334 = global write "Robot Global Data.vi" "Auto State"(4.0 ("Auto State")) -> ()
        }
        frame #6 {
          # "Drive forward, turn robot to +35 degrees clockwise, raise lift to 7000 counts"
          n1335 = global write "Robot Global Data.vi" "Auto Joy 0 Axis X"(0.0 ("Auto Joy 0 Axis X")) -> ()
          n1336 = global write "Robot Global Data.vi" "Auto Joy 0 Axis Y"(-0.3 ("Auto Joy 0 Axis Y")) -> ()
          n1337 = global write "Robot Global Data.vi" "Auto Joy 0 Axis Z"(0.0 ("Auto Joy 0 Axis X")) -> ()
          n1338 = global write "Robot Global Data.vi" "Auto Gyro Hold"(TRUE ("Auto Gyro Hold")) -> ()
          n1339 = global write "Robot Global Data.vi" "Lift Encoder Reset"(FALSE ("Auto Gyro Hold")) -> ()
          n1340 = global write "Robot Global Data.vi" "Wheel Encoder Reset"(FALSE ("Wheel Encoder Reset")) -> ()
          n1341 = while {
            stop <- w1336 stop-if-true
            n1342 = global read "Robot Global Data.vi" "Wheel Encoder Distance"() -> (w1337:dbl)
            n1343 = Less Or Equal?(x=w1337, y=-1625.0) -> (x <= y?=w1336:bool)
          }
          n1344 = global write "Robot Global Data.vi" "PID Target Angle"(35.0 ("Auto Joy 0 Axis Z")) -> ()
          n1345 = global write "Robot Global Data.vi" "Auto Lift Encoder"(7000.0 ("Auto Lift Encoder")) -> ()
          n1346 = global write "Robot Global Data.vi" "Auto State"(5.0 ("Auto State")) -> ()
        }
        frame #7 {
          # "Turn robot to 0 degrees and \ndrive forward until count = 2650"
          n1347 = global write "Robot Global Data.vi" "Auto Joy 0 Axis X"(0.0 ("Auto Joy 0 Axis X")) -> ()
          n1348 = global write "Robot Global Data.vi" "Auto Joy 0 Axis Y"(-0.4 ("Auto Joy 0 Axis Y")) -> ()
          n1349 = global write "Robot Global Data.vi" "Auto Joy 0 Axis Z"(0.0 ("Auto Joy 0 Axis X")) -> ()
          n1350 = global write "Robot Global Data.vi" "Auto Gyro Hold"(TRUE ("Auto Gyro Hold")) -> ()
          n1351 = global write "Robot Global Data.vi" "Lift Encoder Reset"(FALSE ("Auto Gyro Hold")) -> ()
          n1352 = global write "Robot Global Data.vi" "Wheel Encoder Reset"(FALSE ("Wheel Encoder Reset")) -> ()
          n1353 = while {
            stop <- w1347 stop-if-true
            n1354 = global read "Robot Global Data.vi" "Wheel Encoder Distance"() -> (w1348:dbl)
            n1355 = Less Or Equal?(x=w1348, y=-2650.0) -> (x <= y?=w1347:bool)
          }
          n1356 = global write "Robot Global Data.vi" "PID Target Angle"(0.0 ("Auto Joy 0 Axis Z")) -> ()
          n1357 = global write "Robot Global Data.vi" "Auto State"(6.0 ("Auto State")) -> ()
        }
        frame #8 {
          # "Ensure at least 0.5sec wait while crate1 gets lowered onto crate 2."
          # "Set crate1 on crate2"
          n1358 = global write "Robot Global Data.vi" "Auto Joy 0 Axis X"(0.0 ("Auto Joy 0 Axis X")) -> ()
          n1359 = global write "Robot Global Data.vi" "Auto Joy 0 Axis Y"(0.0 ("Auto Joy 0 Axis X")) -> ()
          n1360 = global write "Robot Global Data.vi" "Auto Joy 0 Axis Z"(0.0 ("Auto Joy 0 Axis X")) -> ()
          n1361 = global write "Robot Global Data.vi" "Auto Gyro Hold"(TRUE ("Auto Gyro Hold")) -> ()
          n1362 = while {
            stop <- w1356 stop-if-true
            n1363 = global read "Robot Global Data.vi" "Lift Stopped"() -> (w1356:bool)
          }
          n1364 = global write "Robot Global Data.vi" "Auto Lift Encoder"(5400.0 ("Auto Lift Encoder")) -> ()
          n1365 = Wait (ms)(milliseconds to wait=u32 400) -> ()  [unwired: 1 out]
          n1366 = global write "Robot Global Data.vi" "Auto State"(7.0 ("Auto State")) -> ()
        }
        frame #9 {
          # "Open lift, wait 0.30 sec for lift to open"
          n1367 = global write "Robot Global Data.vi" "Auto Joy 0 Axis X"(0.0 ("Auto Joy 0 Axis X")) -> ()
          n1368 = global write "Robot Global Data.vi" "Auto Joy 0 Axis Y"(0.0 ("Auto Joy 0 Axis X")) -> ()
          n1369 = global write "Robot Global Data.vi" "Auto Joy 0 Axis Z"(0.0 ("Auto Joy 0 Axis X")) -> ()
          n1370 = global write "Robot Global Data.vi" "Auto Gyro Hold"(TRUE ("Auto Gyro Hold")) -> ()
          n1371 = global write "Robot Global Data.vi" "Auto Open Forks"(TRUE ("Auto Gyro Hold")) -> ()
          n1372 = global write "Robot Global Data.vi" "Auto State"(8.0 ("Auto State")) -> ()
          n1373 = Wait (ms)(milliseconds to wait=u32 300) -> ()  [unwired: 1 out]
        }
        frame #10 {
          # "100 is an inch above bottom limit switch"
          # "Lower lift to bottom"
          n1374 = global write "Robot Global Data.vi" "Auto Joy 0 Axis X"(0.0 ("Auto Joy 0 Axis X")) -> ()
          n1375 = global write "Robot Global Data.vi" "Auto Joy 0 Axis Y"(0.0 ("Auto Joy 0 Axis X")) -> ()
          n1376 = global write "Robot Global Data.vi" "Auto Joy 0 Axis Z"(0.0 ("Auto Joy 0 Axis X")) -> ()
          n1377 = global write "Robot Global Data.vi" "Auto Gyro Hold"(TRUE ("Auto Gyro Hold")) -> ()
          n1378 = global write "Robot Global Data.vi" "Auto Open Forks"(TRUE ("Auto Gyro Hold")) -> ()
          n1379 = while {
            stop <- w1371 stop-if-true
            n1380 = global read "Robot Global Data.vi" "Lift Encoder Distance"() -> (w1373:dbl)
            n1381 = Less Or Equal?(x=w1373, y=100.0) -> (x <= y?=w1371:bool)
          }
          n1382 = global write "Robot Global Data.vi" "Auto Lift Encoder"(-200.0 ("Auto Joy 0 Axis X")) -> ()
          n1383 = global write "Robot Global Data.vi" "Auto State"(9.0 ("Auto State")) -> ()
        }
        frame #11 {
          # "Close lift, wait 0.4 sec for lift to close"
          n1384 = global write "Robot Global Data.vi" "Auto Joy 0 Axis X"(0.0 ("Auto Joy 0 Axis X")) -> ()
          n1385 = global write "Robot Global Data.vi" "Auto Joy 0 Axis Y"(0.0 ("Auto Joy 0 Axis X")) -> ()
          n1386 = global write "Robot Global Data.vi" "Auto Joy 0 Axis Z"(0.0 ("Auto Joy 0 Axis X")) -> ()
          n1387 = global write "Robot Global Data.vi" "Auto Gyro Hold"(TRUE ("Auto Gyro Hold")) -> ()
          n1388 = global write "Robot Global Data.vi" "Auto Close Forks"(TRUE ("Auto Gyro Hold")) -> ()
          n1389 = global write "Robot Global Data.vi" "Auto Open Forks"(FALSE ("Auto Gyro Hold")) -> ()
          n1390 = global write "Robot Global Data.vi" "Auto State"(10.0 ("Auto State")) -> ()
          n1391 = Wait (ms)(milliseconds to wait=u32 400) -> ()  [unwired: 1 out]
        }
        frame #12 {
          # "Crate lift was here but now taken out"
          n1392 = global write "Robot Global Data.vi" "Auto Joy 0 Axis X"(0.0 ("Auto Joy 0 Axis X")) -> ()
          n1393 = global write "Robot Global Data.vi" "Auto Joy 0 Axis Y"(0.0 ("Auto Joy 0 Axis X")) -> ()
          n1394 = global write "Robot Global Data.vi" "Auto Joy 0 Axis Z"(0.0 ("Auto Joy 0 Axis X")) -> ()
          n1395 = global write "Robot Global Data.vi" "Auto Gyro Hold"(TRUE ("Auto Gyro Hold")) -> ()
          n1396 = global write "Robot Global Data.vi" "Auto Close Forks"(FALSE ("Auto Gyro Hold")) -> ()
          n1397 = while {
            stop <- w1390 stop-if-true
            n1398 = global read "Robot Global Data.vi" "Lift Stopped"() -> (w1390:bool)
          }
          n1399 = global write "Robot Global Data.vi" "Auto Lift Encoder"(0.0 ("Auto Joy 0 Axis X")) -> ()
          n1400 = Wait (ms)(milliseconds to wait=u32 50) -> ()  [unwired: 1 out]
          n1401 = global write "Robot Global Data.vi" "Auto State"(11.0 ("Auto State")) -> ()
        }
        frame #13 {
          # "Wait for robot to finish turning"
          # "Turn robot 90 degrees clockwise"
          n1402 = global write "Robot Global Data.vi" "Auto Joy 0 Axis X"(0.0 ("Auto Joy 0 Axis X")) -> ()
          n1403 = global write "Robot Global Data.vi" "Auto Joy 0 Axis Y"(0.0 ("Auto Joy 0 Axis X")) -> ()
          n1404 = global write "Robot Global Data.vi" "Auto Joy 0 Axis Z"(0.0 ("Auto Joy 0 Axis X")) -> ()
          n1405 = global write "Robot Global Data.vi" "Auto Gyro Hold"(TRUE ("Auto Gyro Hold")) -> ()
          n1406 = global write "Robot Global Data.vi" "Auto Close Forks"(FALSE ("Auto Gyro Hold")) -> ()
          n1407 = global write "Robot Global Data.vi" "PID Target Angle"(90.0 ("Auto Joy 0 Axis Z")) -> ()
          n1408 = global write "Robot Global Data.vi" "Auto State"(12.0 ("Auto State")) -> ()
          n1409 = Wait (ms)(milliseconds to wait=u32 1300) -> ()  [unwired: 1 out]
        }
        frame #14 {
          # "Reset wheel counter since robot turned,\nhence forward count is incorrect."
          n1410 = global write "Robot Global Data.vi" "Auto Joy 0 Axis X"(0.0 ("Auto Joy 0 Axis X")) -> ()
          n1411 = global write "Robot Global Data.vi" "Auto Joy 0 Axis Y"(0.0 ("Auto Joy 0 Axis X")) -> ()
          n1412 = global write "Robot Global Data.vi" "Auto Joy 0 Axis Z"(0.0 ("Auto Joy 0 Axis X")) -> ()
          n1413 = global write "Robot Global Data.vi" "Auto Gyro Hold"(TRUE ("Auto Gyro Hold")) -> ()
          n1414 = global write "Robot Global Data.vi" "Wheel Encoder Reset"(TRUE ("Wheel Encoder Reset")) -> ()
          n1415 = global write "Robot Global Data.vi" "Auto State"(13.0 ("Auto State")) -> ()
          n1416 = Wait (ms)(milliseconds to wait=u32 50) -> ()  [unwired: 1 out]
        }
        frame #15 {
          # "Enable wheel counter."
          n1417 = global write "Robot Global Data.vi" "Auto Joy 0 Axis X"(0.0 ("Auto Joy 0 Axis X")) -> ()
          n1418 = global write "Robot Global Data.vi" "Auto Joy 0 Axis Y"(0.0 ("Auto Joy 0 Axis X")) -> ()
          n1419 = global write "Robot Global Data.vi" "Auto Joy 0 Axis Z"(0.0 ("Auto Joy 0 Axis X")) -> ()
          n1420 = global write "Robot Global Data.vi" "Auto Gyro Hold"(TRUE ("Auto Gyro Hold")) -> ()
          n1421 = global write "Robot Global Data.vi" "Wheel Encoder Reset"(FALSE ("Wheel Encoder Reset")) -> ()
          n1422 = global write "Robot Global Data.vi" "Auto State"(14.0 ("Auto State")) -> ()
          n1423 = Wait (ms)(milliseconds to wait=u32 50) -> ()  [unwired: 1 out]
        }
        frame #16 {
          # "Drive forward until count = -3400"
          n1424 = global write "Robot Global Data.vi" "Auto Joy 0 Axis X"(0.0 ("Auto Joy 0 Axis X")) -> ()
          n1425 = global write "Robot Global Data.vi" "Auto Joy 0 Axis Y"(-0.6 ("Auto Joy 0 Axis Y")) -> ()
          n1426 = global write "Robot Global Data.vi" "Auto Joy 0 Axis Z"(0.0 ("Auto Joy 0 Axis X")) -> ()
          n1427 = global write "Robot Global Data.vi" "Auto Gyro Hold"(TRUE ("Auto Gyro Hold")) -> ()
          n1428 = global write "Robot Global Data.vi" "Wheel Encoder Reset"(FALSE ("Wheel Encoder Reset")) -> ()
          n1429 = while {
            stop <- w1420 stop-if-true
            n1430 = global read "Robot Global Data.vi" "Wheel Encoder Distance"() -> (w1421:dbl)
            n1431 = Less Or Equal?(x=w1421, y=-3400.0) -> (x <= y?=w1420:bool)
          }
          n1432 = global write "Robot Global Data.vi" "Auto State"(15.0 ("Auto State")) -> ()
        }
        frame #17 {
          # "Stop and wait until teleop"
          n1433 = global write "Robot Global Data.vi" "Auto Joy 0 Axis X"(0.0 ("Auto Joy 0 Axis X")) -> ()
          n1434 = global write "Robot Global Data.vi" "Auto Joy 0 Axis Y"(0.0 ("Auto Joy 0 Axis X")) -> ()
          n1435 = global write "Robot Global Data.vi" "Auto Joy 0 Axis Z"(0.0 ("Auto Joy 0 Axis X")) -> ()
          n1436 = global write "Robot Global Data.vi" "Auto Gyro Hold"(FALSE ("Auto Gyro Hold")) -> ()
          n1437 = global write "Robot Global Data.vi" "Auto State"(16.0 ("Auto State")) -> ()
          n1438 = Wait (ms)(milliseconds to wait=u32 15000) -> ()  [unwired: 1 out]
        }
      }
    }
  }
  n1439 = case shown="True" w14 {
    frame False {
    }
    frame True {
      n1440 = stacked-sequence {
        frame #0 {
          # "Open Forks"
          # "Reset encoders"
          # "Reset Gyro"
          # "Initialize"
          n1441 = global write "Robot Global Data.vi" "Auto Joy 1 Axis Y"(0.0 ("Auto Joy 0 Axis X")) -> ()
          n1442 = global write "Robot Global Data.vi" "Auto Joy 0 Axis X"(0.0 ("Auto Joy 0 Axis X")) -> ()
          n1443 = global write "Robot Global Data.vi" "Auto Joy 0 Axis Y"(0.0 ("Auto Joy 0 Axis X")) -> ()
          n1444 = global write "Robot Global Data.vi" "Auto Joy 0 Axis Z"(0.0 ("Auto Joy 0 Axis X")) -> ()
          n1445 = global write "Robot Global Data.vi" "Gyro Reset"(TRUE ("Auto Gyro Hold")) -> ()
          n1446 = global write "Robot Global Data.vi" "Lift Encoder Reset"(TRUE ("Auto Gyro Hold")) -> ()
          n1447 = global write "Robot Global Data.vi" "Wheel Encoder Reset"(TRUE ("Wheel Encoder Reset")) -> ()
          n1448 = global write "Robot Global Data.vi" "Auto Gyro Hold"(FALSE ("Auto Gyro Hold")) -> ()
          n1449 = global write "Robot Global Data.vi" "Auto Open Forks"(TRUE ("Auto Gyro Hold")) -> ()
          n1450 = global write "Robot Global Data.vi" "Auto Close Forks"(FALSE ("Auto Gyro Hold")) -> ()
          n1451 = global write "Robot Global Data.vi" "PID Target Angle"(0.0 ("Auto Joy 0 Axis Z")) -> ()
          n1452 = global write "Robot Global Data.vi" "Raw Gyro Angle"(0.0 ("Auto Joy 0 Axis Z")) -> ()
          n1453 = global write "Robot Global Data.vi" "Auto State"(0.0 ("Auto State")) -> ()
          n1454 = Wait (ms)(milliseconds to wait=u32 100) -> ()  [unwired: 1 out]
        }
        frame #1 {
          n1455 = global write "Robot Global Data.vi" "Auto Joy 0 Axis X"(0.0 ("Auto Joy 0 Axis X")) -> ()
          n1456 = global write "Robot Global Data.vi" "Auto Joy 0 Axis Y"(0.0 ("Auto Joy 0 Axis X")) -> ()
          n1457 = global write "Robot Global Data.vi" "Auto Joy 0 Axis Z"(0.0 ("Auto Joy 0 Axis X")) -> ()
          n1458 = global write "Robot Global Data.vi" "Gyro Reset"(FALSE ("Auto Gyro Hold")) -> ()
          n1459 = global write "Robot Global Data.vi" "Lift Encoder Reset"(FALSE ("Auto Gyro Hold")) -> ()
          n1460 = global write "Robot Global Data.vi" "Wheel Encoder Reset"(FALSE ("Wheel Encoder Reset")) -> ()
          n1461 = global write "Robot Global Data.vi" "Auto Open Forks"(FALSE ("Auto Gyro Hold")) -> ()
          n1462 = global write "Robot Global Data.vi" "Auto State"(1.0 ("Auto State")) -> ()
          n1463 = Wait (ms)(milliseconds to wait=u32 100) -> ()  [unwired: 1 out]
        }
        frame #2 {
          # "Lower lift to bottom"
          n1464 = global write "Robot Global Data.vi" "Auto Joy 0 Axis X"(0.0 ("Auto Joy 0 Axis X")) -> ()
          n1465 = global write "Robot Global Data.vi" "Auto Joy 0 Axis Y"(0.0 ("Auto Joy 0 Axis X")) -> ()
          n1466 = global write "Robot Global Data.vi" "Auto Joy 0 Axis Z"(0.0 ("Auto Joy 0 Axis X")) -> ()
          n1467 = while {
            stop <- w1456 stop-if-true
            n1468 = global read "Robot Global Data.vi" "Bottom Limit"() -> (w1456:bool)
          }
          n1469 = global write "Robot Global Data.vi" "Auto Lift Encoder"(-30000.0 ("Auto Joy 0 Axis X")) -> ()
          n1470 = global write "Robot Global Data.vi" "Auto State"(2.0 ("Auto State")) -> ()
        }
        frame #3 {
          # "Ensure at least 0.5sec wait"
          n1471 = Wait (ms)(milliseconds to wait=u32 500) -> ()  [unwired: 1 out]
          n1472 = global write "Robot Global Data.vi" "Auto State"(3.0 ("Auto State")) -> ()
        }
        frame #4 {
          # "Ensure at least 0.5sec wait"
          # "Raise lift to +3500 counts"
          n1473 = while {
            stop <- w1462 stop-if-true
            n1474 = global read "Robot Global Data.vi" "Lift Stopped"() -> (w1462:bool)
          }
          n1475 = global write "Robot Global Data.vi" "Auto Lift Encoder"(3500.0 ("Auto Lift Encoder")) -> ()
          n1476 = Wait (ms)(milliseconds to wait=u32 500) -> ()  [unwired: 1 out]
          n1477 = global write "Robot Global Data.vi" "Auto State"(4.0 ("Auto State")) -> ()
        }
        frame #5 {
          # "Ensure at least 0.5sec wait"
          n1478 = Wait (ms)(milliseconds to wait=u32 500) -> ()  [unwired: 1 out]
          n1479 = global write "Robot Global Data.vi" "Auto State"(5.0 ("Auto State")) -> ()
        }
      }
    }
  }
  n1480 = case shown="True" w7 {
    frame False {
    }
    frame True {
      n1481 = stacked-sequence {
        frame #0 {
          # "Reset encoders"
          # "Reset Gyro"
          # "Initialize"
          n1482 = global write "Robot Global Data.vi" "Auto Joy 1 Axis Y"(0.0 ("Auto Joy 0 Axis X")) -> ()
          n1483 = global write "Robot Global Data.vi" "Auto Joy 0 Axis X"(0.0 ("Auto Joy 0 Axis X")) -> ()
          n1484 = global write "Robot Global Data.vi" "Auto Joy 0 Axis Y"(0.0 ("Auto Joy 0 Axis X")) -> ()
          n1485 = global write "Robot Global Data.vi" "Auto Joy 0 Axis Z"(0.0 ("Auto Joy 0 Axis X")) -> ()
          n1486 = global write "Robot Global Data.vi" "Gyro Reset"(TRUE ("Auto Gyro Hold")) -> ()
          n1487 = global write "Robot Global Data.vi" "Lift Encoder Reset"(TRUE ("Auto Gyro Hold")) -> ()
          n1488 = global write "Robot Global Data.vi" "Wheel Encoder Reset"(TRUE ("Wheel Encoder Reset")) -> ()
          n1489 = global write "Robot Global Data.vi" "Auto Gyro Hold"(FALSE ("Auto Gyro Hold")) -> ()
          n1490 = global write "Robot Global Data.vi" "Auto Open Forks"(FALSE ("Auto Gyro Hold")) -> ()
          n1491 = global write "Robot Global Data.vi" "Auto Close Forks"(FALSE ("Auto Gyro Hold")) -> ()
          n1492 = global write "Robot Global Data.vi" "PID Target Angle"(0.0 ("Auto Joy 0 Axis Z")) -> ()
          n1493 = global write "Robot Global Data.vi" "Raw Gyro Angle"(0.0 ("Auto Joy 0 Axis Z")) -> ()
          n1494 = global write "Robot Global Data.vi" "Auto State"(0.0 ("Auto State")) -> ()
          n1495 = Wait (ms)(milliseconds to wait=u32 50) -> ()  [unwired: 1 out]
        }
        frame #1 {
          # "Reset encoders"
          # "Reset Gyro"
          # "Initialize"
          n1496 = global write "Robot Global Data.vi" "Auto Joy 0 Axis X"(0.0 ("Auto Joy 0 Axis X")) -> ()
          n1497 = global write "Robot Global Data.vi" "Auto Joy 0 Axis Y"(0.0 ("Auto Joy 0 Axis X")) -> ()
          n1498 = global write "Robot Global Data.vi" "Auto Joy 0 Axis Z"(0.0 ("Auto Joy 0 Axis X")) -> ()
          n1499 = global write "Robot Global Data.vi" "Gyro Reset"(FALSE ("Auto Gyro Hold")) -> ()
          n1500 = global write "Robot Global Data.vi" "Lift Encoder Reset"(FALSE ("Auto Gyro Hold")) -> ()
          n1501 = global write "Robot Global Data.vi" "Wheel Encoder Reset"(FALSE ("Wheel Encoder Reset")) -> ()
          n1502 = global write "Robot Global Data.vi" "Auto State"(0.0 ("Auto State")) -> ()
          n1503 = Wait (ms)(milliseconds to wait=u32 50) -> ()  [unwired: 1 out]
        }
        frame #2 {
          # "Enable Gyro Hold"
          n1504 = global write "Robot Global Data.vi" "Auto Joy 0 Axis X"(0.0 ("Auto Joy 0 Axis X")) -> ()
          n1505 = global write "Robot Global Data.vi" "Auto Joy 0 Axis Z"(0.0 ("Auto Joy 0 Axis X")) -> ()
          n1506 = global write "Robot Global Data.vi" "Auto Gyro Hold"(TRUE ("Auto Gyro Hold")) -> ()
          n1507 = global write "Robot Global Data.vi" "Lift Encoder Reset"(FALSE ("Auto Gyro Hold")) -> ()
          n1508 = global write "Robot Global Data.vi" "Wheel Encoder Reset"(FALSE ("Wheel Encoder Reset")) -> ()
          n1509 = global write "Robot Global Data.vi" "Auto State"(1.0 ("Auto State")) -> ()
          n1510 = Wait (ms)(milliseconds to wait=u32 50) -> ()  [unwired: 1 out]
        }
        frame #3 {
          # "Wait 0.4sec for forks to close"
          # "Close lift"
          n1511 = global write "Robot Global Data.vi" "Auto Joy 0 Axis X"(0.0 ("Auto Joy 0 Axis X")) -> ()
          n1512 = global write "Robot Global Data.vi" "Auto Joy 0 Axis Z"(0.0 ("Auto Joy 0 Axis X")) -> ()
          n1513 = global write "Robot Global Data.vi" "Auto Gyro Hold"(TRUE ("Auto Gyro Hold")) -> ()
          n1514 = global write "Robot Global Data.vi" "Auto Close Forks"(TRUE ("Auto Gyro Hold")) -> ()
          n1515 = global write "Robot Global Data.vi" "Auto State"(2.0 ("Auto State")) -> ()
          n1516 = Wait (ms)(milliseconds to wait=u32 400) -> ()  [unwired: 1 out]
        }
        frame #4 {
          # "Turn robot 35 degrees counterclockwise\nHold wheel encoder in reset"
          n1517 = global write "Robot Global Data.vi" "Wheel Encoder Reset"(TRUE ("Wheel Encoder Reset")) -> ()
          n1518 = global write "Robot Global Data.vi" "Auto Close Forks"(FALSE ("Auto Gyro Hold")) -> ()
          n1519 = global write "Robot Global Data.vi" "PID Target Angle"(-35.0 ("Auto Joy 0 Axis Z")) -> ()
          n1520 = global write "Robot Global Data.vi" "Auto State"(3.0 ("Auto State")) -> ()
          n1521 = Wait (ms)(milliseconds to wait=u32 400) -> ()  [unwired: 1 out]
        }
        frame #5 {
          # "Drive forward"
          n1522 = global write "Robot Global Data.vi" "Auto Joy 0 Axis X"(0.0 ("Auto Joy 0 Axis X")) -> ()
          n1523 = global write "Robot Global Data.vi" "Auto Joy 0 Axis Y"(-0.3 ("Auto Joy 0 Axis Y")) -> ()
          n1524 = global write "Robot Global Data.vi" "Auto Joy 0 Axis Z"(0.0 ("Auto Joy 0 Axis X")) -> ()
          n1525 = global write "Robot Global Data.vi" "Auto Gyro Hold"(TRUE ("Auto Gyro Hold")) -> ()
          n1526 = global write "Robot Global Data.vi" "Lift Encoder Reset"(FALSE ("Auto Gyro Hold")) -> ()
          n1527 = global write "Robot Global Data.vi" "Wheel Encoder Reset"(FALSE ("Wheel Encoder Reset")) -> ()
          n1528 = while {
            stop <- w1513 stop-if-true
            n1529 = global read "Robot Global Data.vi" "Wheel Encoder Distance"() -> (w1514:dbl)
            n1530 = Less Or Equal?(x=w1514, y=-200.0) -> (x <= y?=w1513:bool)
          }
          n1531 = global write "Robot Global Data.vi" "Auto State"(4.0 ("Auto State")) -> ()
        }
        frame #6 {
          # "Drive forward, turn robot to +35 degrees clockwise, raise lift to 7000 counts"
          n1532 = global write "Robot Global Data.vi" "Auto Joy 0 Axis X"(0.0 ("Auto Joy 0 Axis X")) -> ()
          n1533 = global write "Robot Global Data.vi" "Auto Joy 0 Axis Y"(-0.3 ("Auto Joy 0 Axis Y")) -> ()
          n1534 = global write "Robot Global Data.vi" "Auto Joy 0 Axis Z"(0.0 ("Auto Joy 0 Axis X")) -> ()
          n1535 = global write "Robot Global Data.vi" "Auto Gyro Hold"(TRUE ("Auto Gyro Hold")) -> ()
          n1536 = global write "Robot Global Data.vi" "Lift Encoder Reset"(FALSE ("Auto Gyro Hold")) -> ()
          n1537 = global write "Robot Global Data.vi" "Wheel Encoder Reset"(FALSE ("Wheel Encoder Reset")) -> ()
          n1538 = while {
            stop <- w1525 stop-if-true
            n1539 = global read "Robot Global Data.vi" "Wheel Encoder Distance"() -> (w1526:dbl)
            n1540 = Less Or Equal?(x=w1526, y=-1625.0) -> (x <= y?=w1525:bool)
          }
          n1541 = global write "Robot Global Data.vi" "PID Target Angle"(35.0 ("Auto Joy 0 Axis Z")) -> ()
          n1542 = global write "Robot Global Data.vi" "Auto Lift Encoder"(7000.0 ("Auto Lift Encoder")) -> ()
          n1543 = global write "Robot Global Data.vi" "Auto State"(5.0 ("Auto State")) -> ()
        }
        frame #7 {
          # "Turn robot to 0 degrees and \ndrive forward until count = -1800"
          n1544 = global write "Robot Global Data.vi" "Auto Joy 0 Axis X"(0.0 ("Auto Joy 0 Axis X")) -> ()
          n1545 = global write "Robot Global Data.vi" "Auto Joy 0 Axis Z"(0.0 ("Auto Joy 0 Axis X")) -> ()
          n1546 = global write "Robot Global Data.vi" "Auto Gyro Hold"(TRUE ("Auto Gyro Hold")) -> ()
          n1547 = global write "Robot Global Data.vi" "Lift Encoder Reset"(FALSE ("Auto Gyro Hold")) -> ()
          n1548 = global write "Robot Global Data.vi" "Wheel Encoder Reset"(FALSE ("Wheel Encoder Reset")) -> ()
          n1549 = while {
            stop <- w1535 stop-if-true
            n1550 = global read "Robot Global Data.vi" "Wheel Encoder Distance"() -> (w1536:dbl)
            n1551 = Less Or Equal?(x=w1536, y=-1800.0) -> (x <= y?=w1535:bool)
          }
          n1552 = global write "Robot Global Data.vi" "PID Target Angle"(0.0 ("Auto Joy 0 Axis Z")) -> ()
          n1553 = global write "Robot Global Data.vi" "Auto State"(6.0 ("Auto State")) -> ()
        }
        frame #8 {
          # "Ensure at least 0.5sec wait while crate1 gets lowered onto crate 2."
          # "Set crate1 on crate2"
          n1554 = global write "Robot Global Data.vi" "Auto Joy 0 Axis X"(0.0 ("Auto Joy 0 Axis X")) -> ()
          n1555 = global write "Robot Global Data.vi" "Auto Joy 0 Axis Y"(0.0 ("Auto Joy 0 Axis X")) -> ()
          n1556 = global write "Robot Global Data.vi" "Auto Joy 0 Axis Z"(0.0 ("Auto Joy 0 Axis X")) -> ()
          n1557 = global write "Robot Global Data.vi" "Auto Gyro Hold"(TRUE ("Auto Gyro Hold")) -> ()
          n1558 = while {
            stop <- w1544 stop-if-true
            n1559 = global read "Robot Global Data.vi" "Lift Stopped"() -> (w1544:bool)
          }
          n1560 = global write "Robot Global Data.vi" "Auto Lift Encoder"(5400.0 ("Auto Lift Encoder")) -> ()
          n1561 = Wait (ms)(milliseconds to wait=u32 400) -> ()  [unwired: 1 out]
          n1562 = global write "Robot Global Data.vi" "Auto State"(7.0 ("Auto State")) -> ()
        }
        frame #9 {
          # "Open lift, wait 0.25 sec for lift to open"
          n1563 = global write "Robot Global Data.vi" "Auto Joy 0 Axis X"(0.0 ("Auto Joy 0 Axis X")) -> ()
          n1564 = global write "Robot Global Data.vi" "Auto Joy 0 Axis Y"(0.0 ("Auto Joy 0 Axis X")) -> ()
          n1565 = global write "Robot Global Data.vi" "Auto Joy 0 Axis Z"(0.0 ("Auto Joy 0 Axis X")) -> ()
          n1566 = global write "Robot Global Data.vi" "Auto Gyro Hold"(TRUE ("Auto Gyro Hold")) -> ()
          n1567 = global write "Robot Global Data.vi" "Auto Open Forks"(TRUE ("Auto Gyro Hold")) -> ()
          n1568 = global write "Robot Global Data.vi" "Auto State"(8.0 ("Auto State")) -> ()
          n1569 = Wait (ms)(milliseconds to wait=u32 250) -> ()  [unwired: 1 out]
        }
        frame #10 {
          # "100 is an inch above bottom limit switch"
          # "Lower lift to bottom"
          n1570 = global write "Robot Global Data.vi" "Auto Joy 0 Axis X"(0.0 ("Auto Joy 0 Axis X")) -> ()
          n1571 = global write "Robot Global Data.vi" "Auto Joy 0 Axis Y"(0.0 ("Auto Joy 0 Axis X")) -> ()
          n1572 = global write "Robot Global Data.vi" "Auto Joy 0 Axis Z"(0.0 ("Auto Joy 0 Axis X")) -> ()
          n1573 = global write "Robot Global Data.vi" "Auto Gyro Hold"(TRUE ("Auto Gyro Hold")) -> ()
          n1574 = global write "Robot Global Data.vi" "Auto Open Forks"(FALSE ("Auto Gyro Hold")) -> ()
          n1575 = while {
            stop <- w1559 stop-if-true
            n1576 = global read "Robot Global Data.vi" "Lift Encoder Distance"() -> (w1561:dbl)
            n1577 = Less Or Equal?(x=w1561, y=100.0) -> (x <= y?=w1559:bool)
          }
          n1578 = global write "Robot Global Data.vi" "Auto Lift Encoder"(-200.0 ("Auto Joy 0 Axis X")) -> ()
          n1579 = global write "Robot Global Data.vi" "Auto State"(9.0 ("Auto State")) -> ()
        }
        frame #11 {
          # "Close lift, wait 0.4 sec for lift to close"
          n1580 = global write "Robot Global Data.vi" "Auto Joy 0 Axis X"(0.0 ("Auto Joy 0 Axis X")) -> ()
          n1581 = global write "Robot Global Data.vi" "Auto Joy 0 Axis Y"(0.0 ("Auto Joy 0 Axis X")) -> ()
          n1582 = global write "Robot Global Data.vi" "Auto Joy 0 Axis Z"(0.0 ("Auto Joy 0 Axis X")) -> ()
          n1583 = global write "Robot Global Data.vi" "Auto Gyro Hold"(TRUE ("Auto Gyro Hold")) -> ()
          n1584 = global write "Robot Global Data.vi" "Auto Close Forks"(TRUE ("Auto Gyro Hold")) -> ()
          n1585 = global write "Robot Global Data.vi" "Auto State"(10.0 ("Auto State")) -> ()
          n1586 = Wait (ms)(milliseconds to wait=u32 400) -> ()  [unwired: 1 out]
        }
        frame #12 {
          # "Crate lift was here but now taken out"
          n1587 = global write "Robot Global Data.vi" "Auto Joy 0 Axis X"(0.0 ("Auto Joy 0 Axis X")) -> ()
          n1588 = global write "Robot Global Data.vi" "Auto Joy 0 Axis Y"(0.0 ("Auto Joy 0 Axis X")) -> ()
          n1589 = global write "Robot Global Data.vi" "Auto Joy 0 Axis Z"(0.0 ("Auto Joy 0 Axis X")) -> ()
          n1590 = global write "Robot Global Data.vi" "Auto Gyro Hold"(TRUE ("Auto Gyro Hold")) -> ()
          n1591 = global write "Robot Global Data.vi" "Auto Close Forks"(FALSE ("Auto Gyro Hold")) -> ()
          n1592 = while {
            stop <- w1577 stop-if-true
            n1593 = global read "Robot Global Data.vi" "Lift Stopped"() -> (w1577:bool)
          }
          n1594 = global write "Robot Global Data.vi" "Auto Lift Encoder"(0.0 ("Auto Joy 0 Axis X")) -> ()
          n1595 = Wait (ms)(milliseconds to wait=u32 50) -> ()  [unwired: 1 out]
          n1596 = global write "Robot Global Data.vi" "Auto State"(11.0 ("Auto State")) -> ()
        }
        frame #13 {
          # "Wait for robot to finish turning"
          # "Turn robot 90 degrees clockwise"
          n1597 = global write "Robot Global Data.vi" "Auto Joy 0 Axis X"(0.0 ("Auto Joy 0 Axis X")) -> ()
          n1598 = global write "Robot Global Data.vi" "Auto Joy 0 Axis Y"(0.0 ("Auto Joy 0 Axis X")) -> ()
          n1599 = global write "Robot Global Data.vi" "Auto Joy 0 Axis Z"(0.0 ("Auto Joy 0 Axis X")) -> ()
          n1600 = global write "Robot Global Data.vi" "Auto Gyro Hold"(TRUE ("Auto Gyro Hold")) -> ()
          n1601 = global write "Robot Global Data.vi" "Auto Close Forks"(FALSE ("Auto Gyro Hold")) -> ()
          n1602 = global write "Robot Global Data.vi" "PID Target Angle"(90.0 ("Auto Joy 0 Axis Z")) -> ()
          n1603 = global write "Robot Global Data.vi" "Auto State"(12.0 ("Auto State")) -> ()
          n1604 = Wait (ms)(milliseconds to wait=u32 1300) -> ()  [unwired: 1 out]
        }
        frame #14 {
          # "Reset wheel counter since robot turned,\nhence forward count is incorrect."
          n1605 = global write "Robot Global Data.vi" "Auto Joy 0 Axis X"(0.0 ("Auto Joy 0 Axis X")) -> ()
          n1606 = global write "Robot Global Data.vi" "Auto Joy 0 Axis Y"(0.0 ("Auto Joy 0 Axis X")) -> ()
          n1607 = global write "Robot Global Data.vi" "Auto Joy 0 Axis Z"(0.0 ("Auto Joy 0 Axis X")) -> ()
          n1608 = global write "Robot Global Data.vi" "Auto Gyro Hold"(TRUE ("Auto Gyro Hold")) -> ()
          n1609 = global write "Robot Global Data.vi" "Wheel Encoder Reset"(TRUE ("Wheel Encoder Reset")) -> ()
          n1610 = global write "Robot Global Data.vi" "Auto State"(13.0 ("Auto State")) -> ()
          n1611 = Wait (ms)(milliseconds to wait=u32 50) -> ()  [unwired: 1 out]
        }
        frame #15 {
          # "Enable wheel counter."
          n1612 = global write "Robot Global Data.vi" "Auto Joy 0 Axis X"(0.0 ("Auto Joy 0 Axis X")) -> ()
          n1613 = global write "Robot Global Data.vi" "Auto Joy 0 Axis Y"(0.0 ("Auto Joy 0 Axis X")) -> ()
          n1614 = global write "Robot Global Data.vi" "Auto Joy 0 Axis Z"(0.0 ("Auto Joy 0 Axis X")) -> ()
          n1615 = global write "Robot Global Data.vi" "Auto Gyro Hold"(TRUE ("Auto Gyro Hold")) -> ()
          n1616 = global write "Robot Global Data.vi" "Wheel Encoder Reset"(FALSE ("Wheel Encoder Reset")) -> ()
          n1617 = global write "Robot Global Data.vi" "Auto State"(14.0 ("Auto State")) -> ()
          n1618 = Wait (ms)(milliseconds to wait=u32 50) -> ()  [unwired: 1 out]
        }
        frame #16 {
          # "Drive forward until count = -1850\n(was -1750)"
          n1619 = global write "Robot Global Data.vi" "Auto Joy 0 Axis X"(0.0 ("Auto Joy 0 Axis X")) -> ()
          n1620 = global write "Robot Global Data.vi" "Auto Joy 0 Axis Y"(-0.4 ("Auto Joy 0 Axis Y")) -> ()
          n1621 = global write "Robot Global Data.vi" "Auto Joy 0 Axis Z"(0.0 ("Auto Joy 0 Axis X")) -> ()
          n1622 = global write "Robot Global Data.vi" "Auto Gyro Hold"(TRUE ("Auto Gyro Hold")) -> ()
          n1623 = global write "Robot Global Data.vi" "Wheel Encoder Reset"(FALSE ("Wheel Encoder Reset")) -> ()
          n1624 = while {
            stop <- w1607 stop-if-true
            n1625 = global read "Robot Global Data.vi" "Wheel Encoder Distance"() -> (w1608:dbl)
            n1626 = Less Or Equal?(x=w1608, y=-1850.0) -> (x <= y?=w1607:bool)
          }
          n1627 = global write "Robot Global Data.vi" "Auto State"(15.0 ("Auto State")) -> ()
        }
        frame #17 {
          # "100 is an inch above bottom limit switch\nNote: Trash Can keeps forks from engaing bottom limit\nswitch so use encoder!!!!"
          # "Stop robot, lower crate"
          n1628 = global write "Robot Global Data.vi" "Auto Joy 0 Axis X"(0.0 ("Auto Joy 0 Axis X")) -> ()
          n1629 = global write "Robot Global Data.vi" "Auto Joy 0 Axis Y"(0.0 ("Auto Joy 0 Axis X")) -> ()
          n1630 = global write "Robot Global Data.vi" "Auto Joy 0 Axis Z"(0.0 ("Auto Joy 0 Axis X")) -> ()
          n1631 = global write "Robot Global Data.vi" "Auto Gyro Hold"(TRUE ("Auto Gyro Hold")) -> ()
          n1632 = while {
            stop <- w1615 stop-if-true
            n1633 = global read "Robot Global Data.vi" "Lift Encoder Distance"() -> (w1617:dbl)
            n1634 = Less Or Equal?(x=w1617, y=100.0) -> (x <= y?=w1615:bool)
          }
          n1635 = global write "Robot Global Data.vi" "Auto Lift Encoder"(-200.0 ("Auto Joy 0 Axis X")) -> ()
          n1636 = global write "Robot Global Data.vi" "Auto State"(16.0 ("Auto State")) -> ()
        }
        frame #18 {
          # "Open lift, wait 0.3 sec for lift to open"
          n1637 = global write "Robot Global Data.vi" "Auto Joy 0 Axis X"(0.0 ("Auto Joy 0 Axis X")) -> ()
          n1638 = global write "Robot Global Data.vi" "Auto Joy 0 Axis Y"(0.0 ("Auto Joy 0 Axis X")) -> ()
          n1639 = global write "Robot Global Data.vi" "Auto Joy 0 Axis Z"(0.0 ("Auto Joy 0 Axis X")) -> ()
          n1640 = global write "Robot Global Data.vi" "Auto Gyro Hold"(TRUE ("Auto Gyro Hold")) -> ()
          n1641 = global write "Robot Global Data.vi" "Auto Open Forks"(TRUE ("Auto Gyro Hold")) -> ()
          n1642 = global write "Robot Global Data.vi" "Auto State"(17.0 ("Auto State")) -> ()
          n1643 = Wait (ms)(milliseconds to wait=u32 300) -> ()  [unwired: 1 out]
        }
        frame #19 {
          # "Drive backward until count = -1950\n(was -1850)"
          n1644 = global write "Robot Global Data.vi" "Auto Joy 0 Axis X"(0.0 ("Auto Joy 0 Axis X")) -> ()
          n1645 = global write "Robot Global Data.vi" "Auto Joy 0 Axis Y"(0.2 ("Auto Joy 0 Axis X")) -> ()
          n1646 = global write "Robot Global Data.vi" "Auto Joy 0 Axis Z"(0.0 ("Auto Joy 0 Axis X")) -> ()
          n1647 = global write "Robot Global Data.vi" "Auto Gyro Hold"(TRUE ("Auto Gyro Hold")) -> ()
          n1648 = global write "Robot Global Data.vi" "Auto Open Forks"(FALSE ("Auto Gyro Hold")) -> ()
          n1649 = while {
            stop <- w1633 stop-if-true
            n1650 = global read "Robot Global Data.vi" "Wheel Encoder Distance"() -> (w1632:dbl)
            n1651 = Greater Or Equal?(x=w1632, y=-1950.0) -> (x >= y?=w1633:bool)
          }
          n1652 = global write "Robot Global Data.vi" "Auto State"(18.0 ("Auto State")) -> ()
        }
        frame #20 {
          # "Stop and wait until teleop"
          n1653 = global write "Robot Global Data.vi" "Auto Joy 0 Axis X"(0.0 ("Auto Joy 0 Axis X")) -> ()
          n1654 = global write "Robot Global Data.vi" "Auto Joy 0 Axis Y"(0.0 ("Auto Joy 0 Axis X")) -> ()
          n1655 = global write "Robot Global Data.vi" "Auto Joy 0 Axis Z"(0.0 ("Auto Joy 0 Axis X")) -> ()
          n1656 = global write "Robot Global Data.vi" "Auto Gyro Hold"(FALSE ("Auto Gyro Hold")) -> ()
          n1657 = global write "Robot Global Data.vi" "Auto State"(19.0 ("Auto State")) -> ()
          n1658 = Wait (ms)(milliseconds to wait=u32 15000) -> ()  [unwired: 1 out]
        }
      }
    }
  }
  n1659 = case shown="True" w2 {
    frame False {
    }
    frame True {
      n1660 = stacked-sequence {
        frame #0 {
          # "Reset encoders"
          # "Reset Gyro"
          # "Initialize"
          n1661 = global write "Robot Global Data.vi" "Auto Joy 1 Axis Y"(0.0 ("Auto Joy 0 Axis X")) -> ()
          n1662 = global write "Robot Global Data.vi" "Auto Joy 0 Axis X"(0.0 ("Auto Joy 0 Axis X")) -> ()
          n1663 = global write "Robot Global Data.vi" "Auto Joy 0 Axis Y"(0.0 ("Auto Joy 0 Axis X")) -> ()
          n1664 = global write "Robot Global Data.vi" "Auto Joy 0 Axis Z"(0.0 ("Auto Joy 0 Axis X")) -> ()
          n1665 = global write "Robot Global Data.vi" "Gyro Reset"(TRUE ("Auto Gyro Hold")) -> ()
          n1666 = global write "Robot Global Data.vi" "Lift Encoder Reset"(TRUE ("Auto Gyro Hold")) -> ()
          n1667 = global write "Robot Global Data.vi" "Wheel Encoder Reset"(TRUE ("Wheel Encoder Reset")) -> ()
          n1668 = global write "Robot Global Data.vi" "Auto Gyro Hold"(FALSE ("Auto Gyro Hold")) -> ()
          n1669 = global write "Robot Global Data.vi" "Auto Open Forks"(FALSE ("Auto Gyro Hold")) -> ()
          n1670 = global write "Robot Global Data.vi" "Auto Close Forks"(FALSE ("Auto Gyro Hold")) -> ()
          n1671 = global write "Robot Global Data.vi" "PID Target Angle"(0.0 ("Auto Joy 0 Axis Z")) -> ()
          n1672 = global write "Robot Global Data.vi" "Raw Gyro Angle"(0.0 ("Auto Joy 0 Axis Z")) -> ()
          n1673 = global write "Robot Global Data.vi" "Auto State"(0.0 ("Auto State")) -> ()
          n1674 = Wait (ms)(milliseconds to wait=u32 50) -> ()  [unwired: 1 out]
        }
        frame #1 {
          # "Reset encoders"
          # "Reset Gyro"
          # "Initialize"
          n1675 = global write "Robot Global Data.vi" "Auto Joy 0 Axis X"(0.0 ("Auto Joy 0 Axis X")) -> ()
          n1676 = global write "Robot Global Data.vi" "Auto Joy 0 Axis Y"(0.0 ("Auto Joy 0 Axis X")) -> ()
          n1677 = global write "Robot Global Data.vi" "Auto Joy 0 Axis Z"(0.0 ("Auto Joy 0 Axis X")) -> ()
          n1678 = global write "Robot Global Data.vi" "Gyro Reset"(FALSE ("Auto Gyro Hold")) -> ()
          n1679 = global write "Robot Global Data.vi" "Lift Encoder Reset"(FALSE ("Auto Gyro Hold")) -> ()
          n1680 = global write "Robot Global Data.vi" "Wheel Encoder Reset"(FALSE ("Wheel Encoder Reset")) -> ()
          n1681 = global write "Robot Global Data.vi" "Auto State"(0.0 ("Auto State")) -> ()
          n1682 = Wait (ms)(milliseconds to wait=u32 50) -> ()  [unwired: 1 out]
        }
        frame #2 {
          # "Enable Gyro Hold"
          n1683 = global write "Robot Global Data.vi" "Auto Joy 0 Axis X"(0.0 ("Auto Joy 0 Axis X")) -> ()
          n1684 = global write "Robot Global Data.vi" "Auto Joy 0 Axis Z"(0.0 ("Auto Joy 0 Axis X")) -> ()
          n1685 = global write "Robot Global Data.vi" "Auto Gyro Hold"(TRUE ("Auto Gyro Hold")) -> ()
          n1686 = global write "Robot Global Data.vi" "Lift Encoder Reset"(FALSE ("Auto Gyro Hold")) -> ()
          n1687 = global write "Robot Global Data.vi" "Wheel Encoder Reset"(FALSE ("Wheel Encoder Reset")) -> ()
          n1688 = global write "Robot Global Data.vi" "Auto State"(1.0 ("Auto State")) -> ()
          n1689 = Wait (ms)(milliseconds to wait=u32 10) -> ()  [unwired: 1 out]
        }
        frame #3 {
          # "Wait 0.4sec for forks to close"
          # "Close lift"
          n1690 = global write "Robot Global Data.vi" "Auto Joy 0 Axis X"(0.0 ("Auto Joy 0 Axis X")) -> ()
          n1691 = global write "Robot Global Data.vi" "Auto Joy 0 Axis Z"(0.0 ("Auto Joy 0 Axis X")) -> ()
          n1692 = global write "Robot Global Data.vi" "Auto Gyro Hold"(TRUE ("Auto Gyro Hold")) -> ()
          n1693 = global write "Robot Global Data.vi" "Auto Close Forks"(TRUE ("Auto Gyro Hold")) -> ()
          n1694 = global write "Robot Global Data.vi" "Auto State"(2.0 ("Auto State")) -> ()
          n1695 = Wait (ms)(milliseconds to wait=u32 400) -> ()  [unwired: 1 out]
        }
        frame #4 {
          # "Turn robot 25 degrees clockwise\nHold wheel encoder in reset"
          n1696 = global write "Robot Global Data.vi" "Wheel Encoder Reset"(TRUE ("Wheel Encoder Reset")) -> ()
          n1697 = global write "Robot Global Data.vi" "Auto Close Forks"(FALSE ("Auto Gyro Hold")) -> ()
          n1698 = global write "Robot Global Data.vi" "PID Target Angle"(25.0 ("Auto Joy 0 Axis Z")) -> ()
          n1699 = global write "Robot Global Data.vi" "Auto State"(3.0 ("Auto State")) -> ()
          n1700 = Wait (ms)(milliseconds to wait=u32 400) -> ()  [unwired: 1 out]
        }
        frame #5 {
          # "Drive forward, raise lift to 6800 counts"
          n1701 = global write "Robot Global Data.vi" "Auto Joy 0 Axis X"(0.0 ("Auto Joy 0 Axis X")) -> ()
          n1702 = global write "Robot Global Data.vi" "Auto Joy 0 Axis Y"(-0.38 ("Auto Joy 0 Axis Y")) -> ()
          n1703 = global write "Robot Global Data.vi" "Auto Joy 0 Axis Z"(0.0 ("Auto Joy 0 Axis X")) -> ()
          n1704 = global write "Robot Global Data.vi" "Auto Gyro Hold"(TRUE ("Auto Gyro Hold")) -> ()
          n1705 = global write "Robot Global Data.vi" "Lift Encoder Reset"(FALSE ("Auto Gyro Hold")) -> ()
          n1706 = global write "Robot Global Data.vi" "Wheel Encoder Reset"(FALSE ("Wheel Encoder Reset")) -> ()
          n1707 = while {
            stop <- w1689 stop-if-true
            n1708 = global read "Robot Global Data.vi" "Wheel Encoder Distance"() -> (w1690:dbl)
            n1709 = Less Or Equal?(x=w1690, y=-200.0) -> (x <= y?=w1689:bool)
          }
          n1710 = global write "Robot Global Data.vi" "Auto Lift Encoder"(6800.0 ("Auto Lift Encoder")) -> ()
          n1711 = global write "Robot Global Data.vi" "Auto State"(4.0 ("Auto State")) -> ()
        }
        frame #6 {
          # "Drive forward, turn robot to -25 degrees clockwise"
          n1712 = global write "Robot Global Data.vi" "Auto Joy 0 Axis X"(0.0 ("Auto Joy 0 Axis X")) -> ()
          n1713 = global write "Robot Global Data.vi" "Auto Joy 0 Axis Y"(-0.4 ("Auto Joy 0 Axis Y")) -> ()
          n1714 = global write "Robot Global Data.vi" "Auto Joy 0 Axis Z"(0.0 ("Auto Joy 0 Axis X")) -> ()
          n1715 = global write "Robot Global Data.vi" "Auto Gyro Hold"(TRUE ("Auto Gyro Hold")) -> ()
          n1716 = global write "Robot Global Data.vi" "Lift Encoder Reset"(FALSE ("Auto Gyro Hold")) -> ()
          n1717 = global write "Robot Global Data.vi" "Wheel Encoder Reset"(FALSE ("Wheel Encoder Reset")) -> ()
          n1718 = while {
            stop <- w1700 stop-if-true
            n1719 = global read "Robot Global Data.vi" "Wheel Encoder Distance"() -> (w1701:dbl)
            n1720 = Less Or Equal?(x=w1701, y=-900.0) -> (x <= y?=w1700:bool)
          }
          n1721 = global write "Robot Global Data.vi" "PID Target Angle"(-25.0 ("Auto Joy 0 Axis Z")) -> ()
          n1722 = global write "Robot Global Data.vi" "Auto State"(5.0 ("Auto State")) -> ()
        }
        frame #7 {
          # "Turn robot to 0 degrees and \ndrive forward until count = -1000"
          n1723 = global write "Robot Global Data.vi" "Auto Joy 0 Axis X"(0.0 ("Auto Joy 0 Axis X")) -> ()
          n1724 = global write "Robot Global Data.vi" "Auto Joy 0 Axis Z"(0.0 ("Auto Joy 0 Axis X")) -> ()
          n1725 = global write "Robot Global Data.vi" "Auto Gyro Hold"(TRUE ("Auto Gyro Hold")) -> ()
          n1726 = global write "Robot Global Data.vi" "Lift Encoder Reset"(FALSE ("Auto Gyro Hold")) -> ()
          n1727 = global write "Robot Global Data.vi" "Wheel Encoder Reset"(FALSE ("Wheel Encoder Reset")) -> ()
          n1728 = while {
            stop <- w1710 stop-if-true
            n1729 = global read "Robot Global Data.vi" "Wheel Encoder Distance"() -> (w1711:dbl)
            n1730 = Less Or Equal?(x=w1711, y=-1000.0) -> (x <= y?=w1710:bool)
          }
          n1731 = global write "Robot Global Data.vi" "PID Target Angle"(0.0 ("Auto Joy 0 Axis Z")) -> ()
          n1732 = global write "Robot Global Data.vi" "Auto State"(6.0 ("Auto State")) -> ()
        }
        frame #8 {
          # "Ensure at least 0.35sec wait while crate1 gets lowered onto crate 2."
          # "Set crate1 on crate2"
          n1733 = global write "Robot Global Data.vi" "Auto Joy 0 Axis X"(0.0 ("Auto Joy 0 Axis X")) -> ()
          n1734 = global write "Robot Global Data.vi" "Auto Joy 0 Axis Y"(0.0 ("Auto Joy 0 Axis X")) -> ()
          n1735 = global write "Robot Global Data.vi" "Auto Joy 0 Axis Z"(0.0 ("Auto Joy 0 Axis X")) -> ()
          n1736 = global write "Robot Global Data.vi" "Auto Gyro Hold"(TRUE ("Auto Gyro Hold")) -> ()
          n1737 = while {
            stop <- w1719 stop-if-true
            n1738 = global read "Robot Global Data.vi" "Lift Stopped"() -> (w1719:bool)
          }
          n1739 = global write "Robot Global Data.vi" "Auto Lift Encoder"(5100.0 ("Auto Lift Encoder")) -> ()
          n1740 = Wait (ms)(milliseconds to wait=u32 350) -> ()  [unwired: 1 out]
          n1741 = global write "Robot Global Data.vi" "Auto State"(7.0 ("Auto State")) -> ()
        }
        frame #9 {
          # "Open lift, wait 0.1 sec for lift to open"
          n1742 = global write "Robot Global Data.vi" "Auto Joy 0 Axis X"(0.0 ("Auto Joy 0 Axis X")) -> ()
          n1743 = global write "Robot Global Data.vi" "Auto Joy 0 Axis Y"(0.0 ("Auto Joy 0 Axis X")) -> ()
          n1744 = global write "Robot Global Data.vi" "Auto Joy 0 Axis Z"(0.0 ("Auto Joy 0 Axis X")) -> ()
          n1745 = global write "Robot Global Data.vi" "Auto Gyro Hold"(TRUE ("Auto Gyro Hold")) -> ()
          n1746 = global write "Robot Global Data.vi" "Auto Open Forks"(TRUE ("Auto Gyro Hold")) -> ()
          n1747 = global write "Robot Global Data.vi" "Auto State"(8.0 ("Auto State")) -> ()
          n1748 = Wait (ms)(milliseconds to wait=u32 100) -> ()  [unwired: 1 out]
        }
        frame #10 {
          # "500 is an 5 inches above bottom limit switch"
          # "Lower lift to bottom"
          n1749 = global write "Robot Global Data.vi" "Auto Joy 0 Axis X"(0.0 ("Auto Joy 0 Axis X")) -> ()
          n1750 = global write "Robot Global Data.vi" "Auto Joy 0 Axis Y"(0.0 ("Auto Joy 0 Axis X")) -> ()
          n1751 = global write "Robot Global Data.vi" "Auto Joy 0 Axis Z"(0.0 ("Auto Joy 0 Axis X")) -> ()
          n1752 = global write "Robot Global Data.vi" "Auto Gyro Hold"(TRUE ("Auto Gyro Hold")) -> ()
          n1753 = global write "Robot Global Data.vi" "Auto Open Forks"(FALSE ("Auto Gyro Hold")) -> ()
          n1754 = while {
            stop <- w1734 stop-if-true
            n1755 = global read "Robot Global Data.vi" "Lift Encoder Distance"() -> (w1736:dbl)
            n1756 = Less Or Equal?(x=w1736, y=500.0) -> (x <= y?=w1734:bool)
          }
          n1757 = global write "Robot Global Data.vi" "Auto Lift Encoder"(-200.0 ("Auto Joy 0 Axis X")) -> ()
          n1758 = global write "Robot Global Data.vi" "Auto State"(9.0 ("Auto State")) -> ()
        }
        frame #11 {
          # "Close lift, wait 0.55 sec for lift to close"
          n1759 = global write "Robot Global Data.vi" "Auto Joy 0 Axis X"(0.0 ("Auto Joy 0 Axis X")) -> ()
          n1760 = global write "Robot Global Data.vi" "Auto Joy 0 Axis Y"(0.0 ("Auto Joy 0 Axis X")) -> ()
          n1761 = global write "Robot Global Data.vi" "Auto Joy 0 Axis Z"(0.0 ("Auto Joy 0 Axis X")) -> ()
          n1762 = global write "Robot Global Data.vi" "Auto Gyro Hold"(TRUE ("Auto Gyro Hold")) -> ()
          n1763 = global write "Robot Global Data.vi" "Auto Close Forks"(TRUE ("Auto Gyro Hold")) -> ()
          n1764 = global write "Robot Global Data.vi" "Auto State"(10.0 ("Auto State")) -> ()
          n1765 = Wait (ms)(milliseconds to wait=u32 550) -> ()  [unwired: 1 out]
        }
        frame #12 {
          # "Drive forward, raise lift to 6800 counts"
          n1766 = global write "Robot Global Data.vi" "Auto Joy 0 Axis X"(0.0 ("Auto Joy 0 Axis X")) -> ()
          n1767 = global write "Robot Global Data.vi" "Auto Joy 0 Axis Y"(-0.38 ("Auto Joy 0 Axis Y")) -> ()
          n1768 = global write "Robot Global Data.vi" "Auto Joy 0 Axis Z"(0.0 ("Auto Joy 0 Axis X")) -> ()
          n1769 = global write "Robot Global Data.vi" "Auto Gyro Hold"(TRUE ("Auto Gyro Hold")) -> ()
          n1770 = global write "Robot Global Data.vi" "Lift Encoder Reset"(FALSE ("Auto Gyro Hold")) -> ()
          n1771 = global write "Robot Global Data.vi" "Wheel Encoder Reset"(FALSE ("Wheel Encoder Reset")) -> ()
          n1772 = global write "Robot Global Data.vi" "Auto Close Forks"(FALSE ("Auto Gyro Hold")) -> ()
          n1773 = while {
            stop <- w1754 stop-if-true
            n1774 = global read "Robot Global Data.vi" "Wheel Encoder Distance"() -> (w1755:dbl)
            n1775 = Less Or Equal?(x=w1755, y=-2600.0) -> (x <= y?=w1754:bool)
          }
          n1776 = global write "Robot Global Data.vi" "Auto Lift Encoder"(6800.0 ("Auto Lift Encoder")) -> ()
          n1777 = global write "Robot Global Data.vi" "Auto State"(4.0 ("Auto State")) -> ()
        }
        frame #13 {
          # "Ensure at least 0.3sec wait while crate1 gets lowered onto crate 2."
          # "Stack 3"
          n1778 = global write "Robot Global Data.vi" "Auto Joy 0 Axis X"(0.0 ("Auto Joy 0 Axis X")) -> ()
          n1779 = global write "Robot Global Data.vi" "Auto Joy 0 Axis Y"(0.0 ("Auto Joy 0 Axis X")) -> ()
          n1780 = global write "Robot Global Data.vi" "Auto Joy 0 Axis Z"(0.0 ("Auto Joy 0 Axis X")) -> ()
          n1781 = global write "Robot Global Data.vi" "Auto Gyro Hold"(TRUE ("Auto Gyro Hold")) -> ()
          n1782 = while {
            stop <- w1763 stop-if-true
            n1783 = global read "Robot Global Data.vi" "Lift Stopped"() -> (w1763:bool)
          }
          n1784 = global write "Robot Global Data.vi" "Auto Lift Encoder"(5100.0 ("Auto Lift Encoder")) -> ()
          n1785 = Wait (ms)(milliseconds to wait=u32 300) -> ()  [unwired: 1 out]
          n1786 = global write "Robot Global Data.vi" "Auto State"(7.0 ("Auto State")) -> ()
        }
        frame #14 {
          # "Open lift, wait 0.1 sec for lift to open"
          n1787 = global write "Robot Global Data.vi" "Auto Joy 0 Axis X"(0.0 ("Auto Joy 0 Axis X")) -> ()
          n1788 = global write "Robot Global Data.vi" "Auto Joy 0 Axis Y"(0.0 ("Auto Joy 0 Axis X")) -> ()
          n1789 = global write "Robot Global Data.vi" "Auto Joy 0 Axis Z"(0.0 ("Auto Joy 0 Axis X")) -> ()
          n1790 = global write "Robot Global Data.vi" "Auto Gyro Hold"(TRUE ("Auto Gyro Hold")) -> ()
          n1791 = global write "Robot Global Data.vi" "Auto Open Forks"(TRUE ("Auto Gyro Hold")) -> ()
          n1792 = global write "Robot Global Data.vi" "Auto State"(8.0 ("Auto State")) -> ()
          n1793 = Wait (ms)(milliseconds to wait=u32 100) -> ()  [unwired: 1 out]
        }
        frame #15 {
          # "500 is an 5 inches above bottom limit switch"
          # "Lower lift to bottom"
          n1794 = global write "Robot Global Data.vi" "Auto Joy 0 Axis X"(0.0 ("Auto Joy 0 Axis X")) -> ()
          n1795 = global write "Robot Global Data.vi" "Auto Joy 0 Axis Y"(0.0 ("Auto Joy 0 Axis X")) -> ()
          n1796 = global write "Robot Global Data.vi" "Auto Joy 0 Axis Z"(0.0 ("Auto Joy 0 Axis X")) -> ()
          n1797 = global write "Robot Global Data.vi" "Auto Gyro Hold"(TRUE ("Auto Gyro Hold")) -> ()
          n1798 = global write "Robot Global Data.vi" "Auto Open Forks"(FALSE ("Auto Gyro Hold")) -> ()
          n1799 = while {
            stop <- w1778 stop-if-true
            n1800 = global read "Robot Global Data.vi" "Lift Encoder Distance"() -> (w1780:dbl)
            n1801 = Less Or Equal?(x=w1780, y=500.0) -> (x <= y?=w1778:bool)
          }
          n1802 = global write "Robot Global Data.vi" "Auto Lift Encoder"(-200.0 ("Auto Joy 0 Axis X")) -> ()
          n1803 = global write "Robot Global Data.vi" "Auto State"(9.0 ("Auto State")) -> ()
        }
        frame #16 {
          # "Wait for robot to finish turning"
          # "Turn robot 85 degrees clockwise"
          n1804 = global write "Robot Global Data.vi" "Auto Joy 0 Axis X"(0.0 ("Auto Joy 0 Axis X")) -> ()
          n1805 = global write "Robot Global Data.vi" "Auto Joy 0 Axis Y"(0.0 ("Auto Joy 0 Axis X")) -> ()
          n1806 = global write "Robot Global Data.vi" "Auto Joy 0 Axis Z"(0.0 ("Auto Joy 0 Axis X")) -> ()
          n1807 = global write "Robot Global Data.vi" "Auto Gyro Hold"(TRUE ("Auto Gyro Hold")) -> ()
          n1808 = global write "Robot Global Data.vi" "Auto Close Forks"(FALSE ("Auto Gyro Hold")) -> ()
          n1809 = global write "Robot Global Data.vi" "PID Target Angle"(85.0 ("Auto Joy 0 Axis Z")) -> ()
          n1810 = global write "Robot Global Data.vi" "Auto State"(12.0 ("Auto State")) -> ()
          n1811 = Wait (ms)(milliseconds to wait=u32 1300) -> ()  [unwired: 1 out]
        }
        frame #17 {
          # "Reset wheel counter since robot turned,\nhence forward count is incorrect."
          n1812 = global write "Robot Global Data.vi" "Auto Joy 0 Axis X"(0.0 ("Auto Joy 0 Axis X")) -> ()
          n1813 = global write "Robot Global Data.vi" "Auto Joy 0 Axis Y"(0.0 ("Auto Joy 0 Axis X")) -> ()
          n1814 = global write "Robot Global Data.vi" "Auto Joy 0 Axis Z"(0.0 ("Auto Joy 0 Axis X")) -> ()
          n1815 = global write "Robot Global Data.vi" "Auto Gyro Hold"(TRUE ("Auto Gyro Hold")) -> ()
          n1816 = global write "Robot Global Data.vi" "Wheel Encoder Reset"(TRUE ("Wheel Encoder Reset")) -> ()
          n1817 = global write "Robot Global Data.vi" "Auto State"(13.0 ("Auto State")) -> ()
          n1818 = Wait (ms)(milliseconds to wait=u32 50) -> ()  [unwired: 1 out]
        }
        frame #18 {
          # "Enable wheel counter."
          n1819 = global write "Robot Global Data.vi" "Auto Joy 0 Axis X"(0.0 ("Auto Joy 0 Axis X")) -> ()
          n1820 = global write "Robot Global Data.vi" "Auto Joy 0 Axis Y"(0.0 ("Auto Joy 0 Axis X")) -> ()
          n1821 = global write "Robot Global Data.vi" "Auto Joy 0 Axis Z"(0.0 ("Auto Joy 0 Axis X")) -> ()
          n1822 = global write "Robot Global Data.vi" "Auto Gyro Hold"(TRUE ("Auto Gyro Hold")) -> ()
          n1823 = global write "Robot Global Data.vi" "Wheel Encoder Reset"(FALSE ("Wheel Encoder Reset")) -> ()
          n1824 = global write "Robot Global Data.vi" "Auto State"(14.0 ("Auto State")) -> ()
          n1825 = Wait (ms)(milliseconds to wait=u32 50) -> ()  [unwired: 1 out]
        }
        frame #19 {
          # "Drive forward until count = -1950"
          n1826 = global write "Robot Global Data.vi" "Auto Joy 0 Axis X"(0.0 ("Auto Joy 0 Axis X")) -> ()
          n1827 = global write "Robot Global Data.vi" "Auto Joy 0 Axis Y"(-0.6 ("Auto Joy 0 Axis Y")) -> ()
          n1828 = global write "Robot Global Data.vi" "Auto Joy 0 Axis Z"(0.0 ("Auto Joy 0 Axis X")) -> ()
          n1829 = global write "Robot Global Data.vi" "Auto Gyro Hold"(TRUE ("Auto Gyro Hold")) -> ()
          n1830 = global write "Robot Global Data.vi" "Wheel Encoder Reset"(FALSE ("Wheel Encoder Reset")) -> ()
          n1831 = while {
            stop <- w1810 stop-if-true
            n1832 = global read "Robot Global Data.vi" "Wheel Encoder Distance"() -> (w1811:dbl)
            n1833 = Less Or Equal?(x=w1811, y=-1950.0) -> (x <= y?=w1810:bool)
          }
          n1834 = global write "Robot Global Data.vi" "Auto State"(15.0 ("Auto State")) -> ()
        }
        frame #20 {
          # "Stop robot, lower crate"
          n1835 = global write "Robot Global Data.vi" "Auto Joy 0 Axis X"(0.0 ("Auto Joy 0 Axis X")) -> ()
          n1836 = global write "Robot Global Data.vi" "Auto Joy 0 Axis Y"(0.0 ("Auto Joy 0 Axis X")) -> ()
          n1837 = global write "Robot Global Data.vi" "Auto Joy 0 Axis Z"(0.0 ("Auto Joy 0 Axis X")) -> ()
          n1838 = global write "Robot Global Data.vi" "Auto Gyro Hold"(TRUE ("Auto Gyro Hold")) -> ()
          n1839 = global write "Robot Global Data.vi" "Auto State"(16.0 ("Auto State")) -> ()
          n1840 = Wait (ms)(milliseconds to wait=u32 400) -> ()  [unwired: 1 out]
        }
        frame #21 {
          # "Drive backward until count = -2150\nTurn robot to 80 degrees"
          n1841 = global write "Robot Global Data.vi" "Auto Joy 0 Axis X"(0.0 ("Auto Joy 0 Axis X")) -> ()
          n1842 = global write "Robot Global Data.vi" "Auto Joy 0 Axis Y"(0.2 ("Auto Joy 0 Axis X")) -> ()
          n1843 = global write "Robot Global Data.vi" "Auto Joy 0 Axis Z"(0.0 ("Auto Joy 0 Axis X")) -> ()
          n1844 = global write "Robot Global Data.vi" "Auto Gyro Hold"(TRUE ("Auto Gyro Hold")) -> ()
          n1845 = while {
            stop <- w1826 stop-if-true
            n1846 = global read "Robot Global Data.vi" "Wheel Encoder Distance"() -> (w1825:dbl)
            n1847 = Greater Or Equal?(x=w1825, y=-2150.0) -> (x >= y?=w1826:bool)
          }
          n1848 = global write "Robot Global Data.vi" "PID Target Angle"(80.0 ("Auto Joy 0 Axis Z")) -> ()
          n1849 = global write "Robot Global Data.vi" "Auto State"(18.0 ("Auto State")) -> ()
        }
        frame #22 {
          # "Stop and wait until teleop"
          n1850 = global write "Robot Global Data.vi" "Auto Joy 0 Axis X"(0.0 ("Auto Joy 0 Axis X")) -> ()
          n1851 = global write "Robot Global Data.vi" "Auto Joy 0 Axis Y"(0.0 ("Auto Joy 0 Axis X")) -> ()
          n1852 = global write "Robot Global Data.vi" "Auto Joy 0 Axis Z"(0.0 ("Auto Joy 0 Axis X")) -> ()
          n1853 = global write "Robot Global Data.vi" "Auto Gyro Hold"(FALSE ("Auto Gyro Hold")) -> ()
          n1854 = global write "Robot Global Data.vi" "Auto State"(19.0 ("Auto State")) -> ()
          n1855 = Wait (ms)(milliseconds to wait=u32 10000) -> ()  [unwired: 1 out]
        }
      }
    }
  }
  n1856 = case shown="True" w11 {
    frame False {
    }
    frame True {
      n1857 = stacked-sequence {
        frame #0 {
          # "Pre-set Lift Encoder to +3500 before starting!!!!!!!!!!!"
          # "Reset encoders"
          # "Reset Gyro"
          # "Initialize"
          n1858 = global write "Robot Global Data.vi" "Auto Joy 0 Axis X"(0.0 ("Auto Joy 0 Axis X")) -> ()
          n1859 = global write "Robot Global Data.vi" "Auto Joy 0 Axis Y"(0.0 ("Auto Joy 0 Axis X")) -> ()
          n1860 = global write "Robot Global Data.vi" "Auto Joy 0 Axis Z"(0.0 ("Auto Joy 0 Axis X")) -> ()
          n1861 = global write "Robot Global Data.vi" "Auto Joy 1 Axis Y"(0.0 ("Auto Joy 0 Axis X")) -> ()
          n1862 = global write "Robot Global Data.vi" "Auto Open Forks"(FALSE ("Auto Gyro Hold")) -> ()
          n1863 = global write "Robot Global Data.vi" "Lift Encoder Reset"(TRUE ("Auto Gyro Hold")) -> ()
          n1864 = global write "Robot Global Data.vi" "Wheel Encoder Reset"(TRUE ("Wheel Encoder Reset")) -> ()
          n1865 = global write "Robot Global Data.vi" "Auto Close Forks"(FALSE ("Auto Gyro Hold")) -> ()
          n1866 = global write "Robot Global Data.vi" "Auto Gyro Hold"(FALSE ("Auto Gyro Hold")) -> ()
          n1867 = global write "Robot Global Data.vi" "Gyro Reset"(TRUE ("Auto Gyro Hold")) -> ()
          n1868 = global write "Robot Global Data.vi" "Auto Lift Encoder"(0.0 ("Auto Joy 0 Axis X")) -> ()
          n1869 = global write "Robot Global Data.vi" "Auto Gyro Hold"(FALSE ("Auto Gyro Hold")) -> ()
          n1870 = global write "Robot Global Data.vi" "PID Target Angle"(0.0 ("Auto Joy 0 Axis Z")) -> ()
          n1871 = global write "Robot Global Data.vi" "Raw Gyro Angle"(0.0 ("Auto Joy 0 Axis Z")) -> ()
          n1872 = global write "Robot Global Data.vi" "Auto State"(0.0 ("Auto State")) -> ()
          n1873 = Wait (ms)(milliseconds to wait=u32 50) -> ()  [unwired: 1 out]
        }
        frame #1 {
          # "Initialize"
          n1874 = global write "Robot Global Data.vi" "Auto Joy 0 Axis X"(0.0 ("Auto Joy 0 Axis X")) -> ()
          n1875 = global write "Robot Global Data.vi" "Auto Joy 0 Axis Y"(0.0 ("Auto Joy 0 Axis X")) -> ()
          n1876 = global write "Robot Global Data.vi" "Auto Joy 0 Axis Z"(0.0 ("Auto Joy 0 Axis X")) -> ()
          n1877 = global write "Robot Global Data.vi" "Lift Encoder Reset"(FALSE ("Auto Gyro Hold")) -> ()
          n1878 = global write "Robot Global Data.vi" "Wheel Encoder Reset"(FALSE ("Wheel Encoder Reset")) -> ()
          n1879 = global write "Robot Global Data.vi" "Gyro Reset"(FALSE ("Auto Gyro Hold")) -> ()
          n1880 = global write "Robot Global Data.vi" "Auto State"(1.0 ("Auto State")) -> ()
          n1881 = Wait (ms)(milliseconds to wait=u32 50) -> ()  [unwired: 1 out]
        }
        frame #2 {
          # "Close lift, wait 0.5 sec for lift to close"
          n1882 = global write "Robot Global Data.vi" "Auto Joy 0 Axis X"(0.0 ("Auto Joy 0 Axis X")) -> ()
          n1883 = global write "Robot Global Data.vi" "Auto Joy 0 Axis Y"(0.0 ("Auto Joy 0 Axis X")) -> ()
          n1884 = global write "Robot Global Data.vi" "Auto Joy 0 Axis Z"(0.0 ("Auto Joy 0 Axis X")) -> ()
          n1885 = global write "Robot Global Data.vi" "Auto Gyro Hold"(TRUE ("Auto Gyro Hold")) -> ()
          n1886 = global write "Robot Global Data.vi" "Auto Close Forks"(TRUE ("Auto Gyro Hold")) -> ()
          n1887 = global write "Robot Global Data.vi" "Auto State"(2.0 ("Auto State")) -> ()
          n1888 = Wait (ms)(milliseconds to wait=u32 500) -> ()  [unwired: 1 out]
        }
        frame #3 {
          # "Ensure at least 1.0sec wait"
          # "Lift up can for 1500 counts"
          n1889 = global write "Robot Global Data.vi" "Auto Joy 0 Axis X"(0.0 ("Auto Joy 0 Axis X")) -> ()
          n1890 = global write "Robot Global Data.vi" "Auto Joy 0 Axis Y"(0.0 ("Auto Joy 0 Axis X")) -> ()
          n1891 = global write "Robot Global Data.vi" "Auto Joy 0 Axis Z"(0.0 ("Auto Joy 0 Axis X")) -> ()
          n1892 = global write "Robot Global Data.vi" "Auto Gyro Hold"(TRUE ("Auto Gyro Hold")) -> ()
          n1893 = global write "Robot Global Data.vi" "Auto Close Forks"(FALSE ("Auto Gyro Hold")) -> ()
          n1894 = while {
            stop <- w1872 stop-if-true
            n1895 = global read "Robot Global Data.vi" "Lift Stopped"() -> (w1872:bool)
          }
          n1896 = global write "Robot Global Data.vi" "Auto Lift Encoder"(1500.0 ("Auto Joy 0 Axis X")) -> ()
          n1897 = Wait (ms)(milliseconds to wait=u32 1000) -> ()  [unwired: 1 out]
          n1898 = global write "Robot Global Data.vi" "Auto State"(3.0 ("Auto State")) -> ()
        }
        frame #4 {
          # "Drive backward until count = 1500"
          n1899 = global write "Robot Global Data.vi" "Auto Joy 0 Axis X"(0.0 ("Auto Joy 0 Axis X")) -> ()
          n1900 = global write "Robot Global Data.vi" "Auto Joy 0 Axis Y"(0.33 ("Auto Joy 0 Axis X")) -> ()
          n1901 = global write "Robot Global Data.vi" "Auto Joy 0 Axis Z"(0.0 ("Auto Joy 0 Axis X")) -> ()
          n1902 = global write "Robot Global Data.vi" "Auto Gyro Hold"(TRUE ("Auto Gyro Hold")) -> ()
          n1903 = while {
            stop <- w1880 stop-if-true
            n1904 = global read "Robot Global Data.vi" "Wheel Encoder Distance"() -> (w1878:dbl)
            n1905 = Greater Or Equal?(x=w1878, y=1500.0) -> (x >= y?=w1880:bool)
          }
          n1906 = global write "Robot Global Data.vi" "Auto State"(4.0 ("Auto State")) -> ()
        }
        frame #5 {
          # "Ensure at least 1.0sec wait"
          # "Stop robot and wait for it to stop coasting"
          n1907 = global write "Robot Global Data.vi" "Auto Joy 0 Axis X"(0.0 ("Auto Joy 0 Axis X")) -> ()
          n1908 = global write "Robot Global Data.vi" "Auto Joy 0 Axis Y"(0.0 ("Auto Joy 0 Axis X")) -> ()
          n1909 = global write "Robot Global Data.vi" "Auto Joy 0 Axis Z"(0.0 ("Auto Joy 0 Axis X")) -> ()
          n1910 = global write "Robot Global Data.vi" "Auto Gyro Hold"(TRUE ("Auto Gyro Hold")) -> ()
          n1911 = global write "Robot Global Data.vi" "Auto State"(5.0 ("Auto State")) -> ()
          n1912 = Wait (ms)(milliseconds to wait=u32 1000) -> ()  [unwired: 1 out]
        }
        frame #6 {
          # "Ensure at least 1.0sec wait"
          # "85 gets can back on floor"
          # "Lower crate"
          n1913 = global write "Robot Global Data.vi" "Auto Joy 0 Axis X"(0.0 ("Auto Joy 0 Axis X")) -> ()
          n1914 = global write "Robot Global Data.vi" "Auto Joy 0 Axis Y"(0.0 ("Auto Joy 0 Axis X")) -> ()
          n1915 = global write "Robot Global Data.vi" "Auto Joy 0 Axis Z"(0.0 ("Auto Joy 0 Axis X")) -> ()
          n1916 = global write "Robot Global Data.vi" "Auto Gyro Hold"(TRUE ("Auto Gyro Hold")) -> ()
          n1917 = while {
            stop <- w1894 stop-if-true
            n1918 = global read "Robot Global Data.vi" "Lift Encoder Distance"() -> (w1896:dbl)
            n1919 = Less Or Equal?(x=w1896, y=85.0) -> (x <= y?=w1894:bool)
          }
          n1920 = global write "Robot Global Data.vi" "Auto Lift Encoder"(85.0 ("Auto Joy 0 Axis X")) -> ()
          n1921 = Wait (ms)(milliseconds to wait=u32 1000) -> ()  [unwired: 1 out]
          n1922 = global write "Robot Global Data.vi" "Auto State"(6.0 ("Auto State")) -> ()
        }
        frame #7 {
          # "Open lift, wait 0.3 sec for lift to open"
          n1923 = global write "Robot Global Data.vi" "Auto Joy 0 Axis X"(0.0 ("Auto Joy 0 Axis X")) -> ()
          n1924 = global write "Robot Global Data.vi" "Auto Joy 0 Axis Y"(0.0 ("Auto Joy 0 Axis X")) -> ()
          n1925 = global write "Robot Global Data.vi" "Auto Joy 0 Axis Z"(0.0 ("Auto Joy 0 Axis X")) -> ()
          n1926 = global write "Robot Global Data.vi" "Auto Gyro Hold"(TRUE ("Auto Gyro Hold")) -> ()
          n1927 = global write "Robot Global Data.vi" "Auto Open Forks"(TRUE ("Auto Gyro Hold")) -> ()
          n1928 = global write "Robot Global Data.vi" "Auto State"(6.0 ("Auto State")) -> ()
          n1929 = Wait (ms)(milliseconds to wait=u32 300) -> ()  [unwired: 1 out]
        }
        frame #8 {
          # "Drive backward until count = 1850"
          n1930 = global write "Robot Global Data.vi" "Auto Joy 0 Axis X"(0.0 ("Auto Joy 0 Axis X")) -> ()
          n1931 = global write "Robot Global Data.vi" "Auto Joy 0 Axis Y"(0.3 ("Auto Joy 0 Axis X")) -> ()
          n1932 = global write "Robot Global Data.vi" "Auto Joy 0 Axis Z"(0.0 ("Auto Joy 0 Axis X")) -> ()
          n1933 = global write "Robot Global Data.vi" "Auto Gyro Hold"(TRUE ("Auto Gyro Hold")) -> ()
          n1934 = global write "Robot Global Data.vi" "Auto Open Forks"(FALSE ("Auto Gyro Hold")) -> ()
          n1935 = while {
            stop <- w1912 stop-if-true
            n1936 = global read "Robot Global Data.vi" "Wheel Encoder Distance"() -> (w1911:dbl)
            n1937 = Greater Or Equal?(x=w1911, y=1850.0) -> (x >= y?=w1912:bool)
          }
          n1938 = global write "Robot Global Data.vi" "Auto State"(8.0 ("Auto State")) -> ()
        }
        frame #9 {
          # "Stop and wait until teleop"
          n1939 = global write "Robot Global Data.vi" "Auto Joy 0 Axis X"(0.0 ("Auto Joy 0 Axis X")) -> ()
          n1940 = global write "Robot Global Data.vi" "Auto Joy 0 Axis Y"(0.0 ("Auto Joy 0 Axis X")) -> ()
          n1941 = global write "Robot Global Data.vi" "Auto Joy 0 Axis Z"(0.0 ("Auto Joy 0 Axis X")) -> ()
          n1942 = global write "Robot Global Data.vi" "Auto Gyro Hold"(FALSE ("Auto Gyro Hold")) -> ()
          n1943 = global write "Robot Global Data.vi" "Auto State"(9.0 ("Auto State")) -> ()
          n1944 = Wait (ms)(milliseconds to wait=u32 15000) -> ()  [unwired: 1 out]
        }
      }
    }
  }
  n1945 = case shown="True" w9 {
    frame False {
    }
    frame True {
      n1946 = stacked-sequence {
        frame #0 {
          # "Pre-set Lift Encoder to +3500 before starting!!!!!!!!!!!"
          # "Reset encoders"
          # "Reset Gyro"
          # "Initialize"
          n1947 = global write "Robot Global Data.vi" "Auto Joy 0 Axis X"(0.0 ("Auto Joy 0 Axis X")) -> ()
          n1948 = global write "Robot Global Data.vi" "Auto Joy 0 Axis Y"(0.0 ("Auto Joy 0 Axis X")) -> ()
          n1949 = global write "Robot Global Data.vi" "Auto Joy 0 Axis Z"(0.0 ("Auto Joy 0 Axis X")) -> ()
          n1950 = global write "Robot Global Data.vi" "Auto Joy 1 Axis Y"(0.0 ("Auto Joy 0 Axis X")) -> ()
          n1951 = global write "Robot Global Data.vi" "Auto Open Forks"(FALSE ("Auto Gyro Hold")) -> ()
          n1952 = global write "Robot Global Data.vi" "Lift Encoder Reset"(TRUE ("Auto Gyro Hold")) -> ()
          n1953 = global write "Robot Global Data.vi" "Wheel Encoder Reset"(TRUE ("Wheel Encoder Reset")) -> ()
          n1954 = global write "Robot Global Data.vi" "Auto Close Forks"(FALSE ("Auto Gyro Hold")) -> ()
          n1955 = global write "Robot Global Data.vi" "Auto Gyro Hold"(FALSE ("Auto Gyro Hold")) -> ()
          n1956 = global write "Robot Global Data.vi" "Gyro Reset"(TRUE ("Auto Gyro Hold")) -> ()
          n1957 = global write "Robot Global Data.vi" "Auto Lift Encoder"(0.0 ("Auto Joy 0 Axis X")) -> ()
          n1958 = global write "Robot Global Data.vi" "Auto Gyro Hold"(FALSE ("Auto Gyro Hold")) -> ()
          n1959 = global write "Robot Global Data.vi" "PID Target Angle"(0.0 ("Auto Joy 0 Axis Z")) -> ()
          n1960 = global write "Robot Global Data.vi" "Raw Gyro Angle"(0.0 ("Auto Joy 0 Axis Z")) -> ()
          n1961 = global write "Robot Global Data.vi" "Auto State"(0.0 ("Auto State")) -> ()
          n1962 = Wait (ms)(milliseconds to wait=u32 50) -> ()  [unwired: 1 out]
        }
        frame #1 {
          # "Initialize"
          n1963 = global write "Robot Global Data.vi" "Auto Joy 0 Axis X"(0.0 ("Auto Joy 0 Axis X")) -> ()
          n1964 = global write "Robot Global Data.vi" "Auto Joy 0 Axis Y"(0.0 ("Auto Joy 0 Axis X")) -> ()
          n1965 = global write "Robot Global Data.vi" "Auto Joy 0 Axis Z"(0.0 ("Auto Joy 0 Axis X")) -> ()
          n1966 = global write "Robot Global Data.vi" "Lift Encoder Reset"(FALSE ("Auto Gyro Hold")) -> ()
          n1967 = global write "Robot Global Data.vi" "Wheel Encoder Reset"(FALSE ("Wheel Encoder Reset")) -> ()
          n1968 = global write "Robot Global Data.vi" "Gyro Reset"(FALSE ("Auto Gyro Hold")) -> ()
          n1969 = global write "Robot Global Data.vi" "Auto State"(1.0 ("Auto State")) -> ()
          n1970 = Wait (ms)(milliseconds to wait=u32 50) -> ()  [unwired: 1 out]
        }
        frame #2 {
          # "Close lift, wait 0.5 sec for lift to close"
          n1971 = global write "Robot Global Data.vi" "Auto Joy 0 Axis X"(0.0 ("Auto Joy 0 Axis X")) -> ()
          n1972 = global write "Robot Global Data.vi" "Auto Joy 0 Axis Y"(0.0 ("Auto Joy 0 Axis X")) -> ()
          n1973 = global write "Robot Global Data.vi" "Auto Joy 0 Axis Z"(0.0 ("Auto Joy 0 Axis X")) -> ()
          n1974 = global write "Robot Global Data.vi" "Auto Gyro Hold"(TRUE ("Auto Gyro Hold")) -> ()
          n1975 = global write "Robot Global Data.vi" "Auto Close Forks"(TRUE ("Auto Gyro Hold")) -> ()
          n1976 = global write "Robot Global Data.vi" "Auto State"(2.0 ("Auto State")) -> ()
          n1977 = Wait (ms)(milliseconds to wait=u32 500) -> ()  [unwired: 1 out]
        }
        frame #3 {
          # "Ensure at least 1.0sec wait"
          # "Lift up can for 2100 counts"
          n1978 = global write "Robot Global Data.vi" "Auto Joy 0 Axis X"(0.0 ("Auto Joy 0 Axis X")) -> ()
          n1979 = global write "Robot Global Data.vi" "Auto Joy 0 Axis Y"(0.0 ("Auto Joy 0 Axis X")) -> ()
          n1980 = global write "Robot Global Data.vi" "Auto Joy 0 Axis Z"(0.0 ("Auto Joy 0 Axis X")) -> ()
          n1981 = global write "Robot Global Data.vi" "Auto Gyro Hold"(TRUE ("Auto Gyro Hold")) -> ()
          n1982 = global write "Robot Global Data.vi" "Auto Close Forks"(FALSE ("Auto Gyro Hold")) -> ()
          n1983 = while {
            stop <- w1958 stop-if-true
            n1984 = global read "Robot Global Data.vi" "Lift Stopped"() -> (w1958:bool)
          }
          n1985 = global write "Robot Global Data.vi" "Auto Lift Encoder"(2100.0 ("Auto Joy 0 Axis X")) -> ()
          n1986 = Wait (ms)(milliseconds to wait=u32 1000) -> ()  [unwired: 1 out]
          n1987 = global write "Robot Global Data.vi" "Auto State"(3.0 ("Auto State")) -> ()
        }
        frame #4 {
          # "Drive backward until count = 1650"
          n1988 = global write "Robot Global Data.vi" "Auto Joy 0 Axis X"(0.0 ("Auto Joy 0 Axis X")) -> ()
          n1989 = global write "Robot Global Data.vi" "Auto Joy 0 Axis Y"(0.33 ("Auto Joy 0 Axis X")) -> ()
          n1990 = global write "Robot Global Data.vi" "Auto Joy 0 Axis Z"(0.0 ("Auto Joy 0 Axis X")) -> ()
          n1991 = global write "Robot Global Data.vi" "Auto Gyro Hold"(TRUE ("Auto Gyro Hold")) -> ()
          n1992 = while {
            stop <- w1966 stop-if-true
            n1993 = global read "Robot Global Data.vi" "Wheel Encoder Distance"() -> (w1964:dbl)
            n1994 = Greater Or Equal?(x=w1964, y=1650.0) -> (x >= y?=w1966:bool)
          }
          n1995 = global write "Robot Global Data.vi" "Auto State"(4.0 ("Auto State")) -> ()
        }
        frame #5 {
          # "Ensure at least 1.0sec wait"
          # "Stop robot and wait for it to stop coasting"
          n1996 = global write "Robot Global Data.vi" "Auto Joy 0 Axis X"(0.0 ("Auto Joy 0 Axis X")) -> ()
          n1997 = global write "Robot Global Data.vi" "Auto Joy 0 Axis Y"(0.0 ("Auto Joy 0 Axis X")) -> ()
          n1998 = global write "Robot Global Data.vi" "Auto Joy 0 Axis Z"(0.0 ("Auto Joy 0 Axis X")) -> ()
          n1999 = global write "Robot Global Data.vi" "Auto Gyro Hold"(TRUE ("Auto Gyro Hold")) -> ()
          n2000 = global write "Robot Global Data.vi" "Auto State"(5.0 ("Auto State")) -> ()
          n2001 = Wait (ms)(milliseconds to wait=u32 1000) -> ()  [unwired: 1 out]
        }
        frame #6 {
          # "Ensure at least 1.0sec wait"
          # "85 gets can back on floor"
          # "Lower crate"
          n2002 = global write "Robot Global Data.vi" "Auto Joy 0 Axis X"(0.0 ("Auto Joy 0 Axis X")) -> ()
          n2003 = global write "Robot Global Data.vi" "Auto Joy 0 Axis Y"(0.0 ("Auto Joy 0 Axis X")) -> ()
          n2004 = global write "Robot Global Data.vi" "Auto Joy 0 Axis Z"(0.0 ("Auto Joy 0 Axis X")) -> ()
          n2005 = global write "Robot Global Data.vi" "Auto Gyro Hold"(TRUE ("Auto Gyro Hold")) -> ()
          n2006 = while {
            stop <- w1980 stop-if-true
            n2007 = global read "Robot Global Data.vi" "Lift Encoder Distance"() -> (w1982:dbl)
            n2008 = Less Or Equal?(x=w1982, y=85.0) -> (x <= y?=w1980:bool)
          }
          n2009 = global write "Robot Global Data.vi" "Auto Lift Encoder"(85.0 ("Auto Joy 0 Axis X")) -> ()
          n2010 = Wait (ms)(milliseconds to wait=u32 1000) -> ()  [unwired: 1 out]
          n2011 = global write "Robot Global Data.vi" "Auto State"(6.0 ("Auto State")) -> ()
        }
        frame #7 {
          # "Open lift, wait 0.3 sec for lift to open"
          n2012 = global write "Robot Global Data.vi" "Auto Joy 0 Axis X"(0.0 ("Auto Joy 0 Axis X")) -> ()
          n2013 = global write "Robot Global Data.vi" "Auto Joy 0 Axis Y"(0.0 ("Auto Joy 0 Axis X")) -> ()
          n2014 = global write "Robot Global Data.vi" "Auto Joy 0 Axis Z"(0.0 ("Auto Joy 0 Axis X")) -> ()
          n2015 = global write "Robot Global Data.vi" "Auto Gyro Hold"(TRUE ("Auto Gyro Hold")) -> ()
          n2016 = global write "Robot Global Data.vi" "Auto Open Forks"(TRUE ("Auto Gyro Hold")) -> ()
          n2017 = global write "Robot Global Data.vi" "Auto State"(6.0 ("Auto State")) -> ()
          n2018 = Wait (ms)(milliseconds to wait=u32 300) -> ()  [unwired: 1 out]
        }
        frame #8 {
          # "Drive backward until count = 1850\n(was 2000)"
          n2019 = global write "Robot Global Data.vi" "Auto Joy 0 Axis X"(0.0 ("Auto Joy 0 Axis X")) -> ()
          n2020 = global write "Robot Global Data.vi" "Auto Joy 0 Axis Y"(0.3 ("Auto Joy 0 Axis X")) -> ()
          n2021 = global write "Robot Global Data.vi" "Auto Joy 0 Axis Z"(0.0 ("Auto Joy 0 Axis X")) -> ()
          n2022 = global write "Robot Global Data.vi" "Auto Gyro Hold"(TRUE ("Auto Gyro Hold")) -> ()
          n2023 = global write "Robot Global Data.vi" "Auto Open Forks"(FALSE ("Auto Gyro Hold")) -> ()
          n2024 = while {
            stop <- w1998 stop-if-true
            n2025 = global read "Robot Global Data.vi" "Wheel Encoder Distance"() -> (w1997:dbl)
            n2026 = Greater Or Equal?(x=w1997, y=1850.0) -> (x >= y?=w1998:bool)
          }
          n2027 = global write "Robot Global Data.vi" "Auto State"(8.0 ("Auto State")) -> ()
        }
        frame #9 {
          # "Stop and wait until teleop"
          n2028 = global write "Robot Global Data.vi" "Auto Joy 0 Axis X"(0.0 ("Auto Joy 0 Axis X")) -> ()
          n2029 = global write "Robot Global Data.vi" "Auto Joy 0 Axis Y"(0.0 ("Auto Joy 0 Axis X")) -> ()
          n2030 = global write "Robot Global Data.vi" "Auto Joy 0 Axis Z"(0.0 ("Auto Joy 0 Axis X")) -> ()
          n2031 = global write "Robot Global Data.vi" "Auto Gyro Hold"(FALSE ("Auto Gyro Hold")) -> ()
          n2032 = global write "Robot Global Data.vi" "Auto State"(9.0 ("Auto State")) -> ()
          n2033 = Wait (ms)(milliseconds to wait=u32 15000) -> ()  [unwired: 1 out]
        }
      }
    }
  }
  n2034 = case shown="True" w4 {
    frame False {
    }
    frame True {
      n2035 = stacked-sequence {
        frame #0 {
          # "Pre-set Lift Encoder to +3500 before starting!!!!!!!!!!!"
          # "Reset encoders"
          # "Reset Gyro"
          # "Initialize"
          n2036 = global write "Robot Global Data.vi" "Auto Joy 0 Axis X"(0.0 ("Auto Joy 0 Axis X")) -> ()
          n2037 = global write "Robot Global Data.vi" "Auto Joy 0 Axis Y"(0.0 ("Auto Joy 0 Axis X")) -> ()
          n2038 = global write "Robot Global Data.vi" "Auto Joy 0 Axis Z"(0.0 ("Auto Joy 0 Axis X")) -> ()
          n2039 = global write "Robot Global Data.vi" "Auto Joy 1 Axis Y"(0.0 ("Auto Joy 0 Axis X")) -> ()
          n2040 = global write "Robot Global Data.vi" "Auto Open Forks"(FALSE ("Auto Gyro Hold")) -> ()
          n2041 = global write "Robot Global Data.vi" "Lift Encoder Reset"(TRUE ("Auto Gyro Hold")) -> ()
          n2042 = global write "Robot Global Data.vi" "Wheel Encoder Reset"(TRUE ("Wheel Encoder Reset")) -> ()
          n2043 = global write "Robot Global Data.vi" "Auto Close Forks"(FALSE ("Auto Gyro Hold")) -> ()
          n2044 = global write "Robot Global Data.vi" "Auto Gyro Hold"(FALSE ("Auto Gyro Hold")) -> ()
          n2045 = global write "Robot Global Data.vi" "Gyro Reset"(TRUE ("Auto Gyro Hold")) -> ()
          n2046 = global write "Robot Global Data.vi" "Auto Lift Encoder"(0.0 ("Auto Joy 0 Axis X")) -> ()
          n2047 = global write "Robot Global Data.vi" "Auto Gyro Hold"(FALSE ("Auto Gyro Hold")) -> ()
          n2048 = global write "Robot Global Data.vi" "PID Target Angle"(0.0 ("Auto Joy 0 Axis Z")) -> ()
          n2049 = global write "Robot Global Data.vi" "Raw Gyro Angle"(0.0 ("Auto Joy 0 Axis Z")) -> ()
          n2050 = global write "Robot Global Data.vi" "Auto State"(0.0 ("Auto State")) -> ()
          n2051 = Wait (ms)(milliseconds to wait=u32 50) -> ()  [unwired: 1 out]
        }
        frame #1 {
          # "Initialize"
          n2052 = global write "Robot Global Data.vi" "Auto Joy 0 Axis X"(0.0 ("Auto Joy 0 Axis X")) -> ()
          n2053 = global write "Robot Global Data.vi" "Auto Joy 0 Axis Y"(0.0 ("Auto Joy 0 Axis X")) -> ()
          n2054 = global write "Robot Global Data.vi" "Auto Joy 0 Axis Z"(0.0 ("Auto Joy 0 Axis X")) -> ()
          n2055 = global write "Robot Global Data.vi" "Lift Encoder Reset"(FALSE ("Auto Gyro Hold")) -> ()
          n2056 = global write "Robot Global Data.vi" "Wheel Encoder Reset"(FALSE ("Wheel Encoder Reset")) -> ()
          n2057 = global write "Robot Global Data.vi" "Gyro Reset"(FALSE ("Auto Gyro Hold")) -> ()
          n2058 = global write "Robot Global Data.vi" "Auto State"(1.0 ("Auto State")) -> ()
          n2059 = Wait (ms)(milliseconds to wait=u32 50) -> ()  [unwired: 1 out]
        }
        frame #2 {
          # "Close lift, wait 0.5 sec for lift to close"
          n2060 = global write "Robot Global Data.vi" "Auto Joy 0 Axis X"(0.0 ("Auto Joy 0 Axis X")) -> ()
          n2061 = global write "Robot Global Data.vi" "Auto Joy 0 Axis Y"(0.0 ("Auto Joy 0 Axis X")) -> ()
          n2062 = global write "Robot Global Data.vi" "Auto Joy 0 Axis Z"(0.0 ("Auto Joy 0 Axis X")) -> ()
          n2063 = global write "Robot Global Data.vi" "Auto Gyro Hold"(TRUE ("Auto Gyro Hold")) -> ()
          n2064 = global write "Robot Global Data.vi" "Auto Close Forks"(TRUE ("Auto Gyro Hold")) -> ()
          n2065 = global write "Robot Global Data.vi" "Auto State"(2.0 ("Auto State")) -> ()
          n2066 = Wait (ms)(milliseconds to wait=u32 500) -> ()  [unwired: 1 out]
        }
        frame #3 {
          # "Ensure at least 6.0sec wait"
          # "Lift up can for 13000 counts"
          n2067 = global write "Robot Global Data.vi" "Auto Joy 0 Axis X"(0.0 ("Auto Joy 0 Axis X")) -> ()
          n2068 = global write "Robot Global Data.vi" "Auto Joy 0 Axis Y"(0.0 ("Auto Joy 0 Axis X")) -> ()
          n2069 = global write "Robot Global Data.vi" "Auto Joy 0 Axis Z"(0.0 ("Auto Joy 0 Axis X")) -> ()
          n2070 = global write "Robot Global Data.vi" "Auto Gyro Hold"(TRUE ("Auto Gyro Hold")) -> ()
          n2071 = global write "Robot Global Data.vi" "Auto Close Forks"(FALSE ("Auto Gyro Hold")) -> ()
          n2072 = while {
            stop <- w2044 stop-if-true
            n2073 = global read "Robot Global Data.vi" "Lift Stopped"() -> (w2044:bool)
          }
          n2074 = global write "Robot Global Data.vi" "Auto Lift Encoder"(13000.0 ("Auto Joy 0 Axis X")) -> ()
          n2075 = Wait (ms)(milliseconds to wait=u32 6000) -> ()  [unwired: 1 out]
          n2076 = global write "Robot Global Data.vi" "Auto State"(3.0 ("Auto State")) -> ()
        }
        frame #4 {
          # "Drive forward until count = 450"
          n2077 = global write "Robot Global Data.vi" "Auto Joy 0 Axis X"(0.0 ("Auto Joy 0 Axis X")) -> ()
          n2078 = global write "Robot Global Data.vi" "Auto Joy 0 Axis Y"(-0.25 ("Auto Joy 0 Axis X")) -> ()
          n2079 = global write "Robot Global Data.vi" "Auto Joy 0 Axis Z"(0.0 ("Auto Joy 0 Axis X")) -> ()
          n2080 = global write "Robot Global Data.vi" "Auto Gyro Hold"(TRUE ("Auto Gyro Hold")) -> ()
          n2081 = while {
            stop <- w2052 stop-if-true
            n2082 = global read "Robot Global Data.vi" "Wheel Encoder Distance"() -> (w2051:dbl)
            n2083 = Less Or Equal?(x=w2051, y=-450.0) -> (x <= y?=w2052:bool)
          }
          n2084 = global write "Robot Global Data.vi" "Auto State"(4.0 ("Auto State")) -> ()
        }
        frame #5 {
          # "Stop and wait until teleop"
          n2085 = global write "Robot Global Data.vi" "Auto Joy 0 Axis X"(0.0 ("Auto Joy 0 Axis X")) -> ()
          n2086 = global write "Robot Global Data.vi" "Auto Joy 0 Axis Y"(0.0 ("Auto Joy 0 Axis X")) -> ()
          n2087 = global write "Robot Global Data.vi" "Auto Joy 0 Axis Z"(0.0 ("Auto Joy 0 Axis X")) -> ()
          n2088 = global write "Robot Global Data.vi" "Auto Gyro Hold"(FALSE ("Auto Gyro Hold")) -> ()
          n2089 = global write "Robot Global Data.vi" "Auto State"(5.0 ("Auto State")) -> ()
          n2090 = Wait (ms)(milliseconds to wait=u32 15000) -> ()  [unwired: 1 out]
        }
      }
    }
  }
